vi "FP_Tracker_2.2.vi"() -> ()   [LabVIEW 2018, in "Tracker.lvlib"]
uses:
  Tracker.lvlib
  SubVi's/Controls/CTL_IO_status_indicator.ctl
  SubVi's/Controls/CTL_Zones_control_and_indicator.ctl
  SubVi's/Controls/CTL_Zone_indicator.ctl
  SubVi's/Controls/CTL_All_References.ctl
  Common/Typedefs/CTL_Controls_References.ctl
  Common/Typedefs/CTL_Indicators_References.ctl
  Common/Typedefs/CTL_Panes_and_VIs_References.ctl
  SubVi's/Controls/CTL_Cage_radial_segmentation.ctl
  SubVi's/Controls/CTL_Image_Geometrical_and_scaling_parameters.ctl
  <vilib>/ProgressBar/Progress Bar Dialog.lvclass
  SubVi's/Controls/CTL_Calibration_parameters.ctl
  SubVi's/Controls/CTL_Dispenser_calibration_info.ctl
  SubVi's/Controls/CTL_Pre-filter_params.ctl
  SubVi's/Controls/CTL_Mouse_Draw_Params.ctl
  SubVi's/Controls/CTL_IO_params_cluster.ctl
  SubVi's/Controls/CTL_Overlays_cluster.ctl
  SubVi's/Controls/CTL_Animal_Coordinates_and_Speed.ctl
  SubVi's/Controls/CTL_Settings_cluster.ctl
  SubVi's/Controls/CTL_Histogram_parameters.ctl
  SubVi's/Controls/CTL_Filter_selector.ctl
  SubVi's/Controls/CTL_Acquisition_speed_selector.ctl
  Common/Typedefs/CTL_Segmented_plot_parameters_2.ctl
  Libraries/Cage Diagram/Typedefs/CTL_Cage_type.ctl
  SubVi's/Controls/CTL_Cage_all_segmentation_params_set.ctl
  SubVi's/Controls/CTL_Conditions_Array.ctl
  SubVi's/Controls/CTL_Conditions_Cluster.ctl
  SubVi's/Controls/CTL_Condition_type.ctl
  SubVi's/Controls/CTL_Comparison_type.ctl
  SubVi's/Controls/CTL_Validity_check_criteria.ctl
  SubVi's/Controls/CTL_Response_info.ctl
  SubVi's/Controls/CTL_Condition_response_type.ctl
  SubVi's/Controls/CTL_Reponse_port_info.ctl
  SubVi's/Controls/CTL_Pixel_to_Zone_array.ctl
  SubVi's/Controls/CTL_Stats_parameters_(online).ctl
  SubVi's/Controls/CTL_Control_States.ctl
  SubVi's/Controls/CTL_States_cluster.ctl
  <vilib>/Platform/TimedLoop/XDataNode/timing_clust.ctl
  <vilib>/Platform/TimedLoop/XDataNode/nitl_modes.ctl
  <vilib>/Platform/TimedLoop/XDataNode/wakeup.ctl
  <vilib>/Utility/error.llb/DialogType.ctl
  SubVi's/Controls/CTL_Settings_parameters_groups.ctl
  Libraries/TTL IO/Typedefs/CTL_Parameter_transfer_name.ctl
  SubVi's/Controls/CTL_Post-processing_params.ctl
  <vilib>/vision/Image Controls.llb/IMAQ Image.ctl
  <vilib>/Utility/miscctls.llb/LVBoundsTypeDef.ctl
  SubVi's/Controls/CTL_Color_ramp.ctl
  <vilib>/Instr/_visa.llb/VISA Flush IO Buffer Mask.ctl
  SubVi's/Controls/CTL_Full_data_frame.ctl
  SubVi's/Controls/CTL_Measurements_and_Statistics.ctl
  <extravilib>/ChannelInstances/Stream-t'Tracker.lvlib-CTL_Full_data_frame.ctl'/Read With Abort.vi
  <extravilib>/ChannelInstances/Lossy Stream-t'Tracker.lvlib-CTL_Measurements_and_Statistics.ctl'/Write With Abort.vi
  <extravilib>/ChannelInstances/Lossy Stream-t'Tracker.lvlib-CTL_Animal_Coordinates_and_Speed.ctl'/Read With Abort.vi
  <extravilib>/ChannelInstances/Lossy Stream-a[.](dbl)/Read With Abort.vi
  <extravilib>/ChannelInstances/Lossy Stream-t'Tracker.lvlib-CTL_Measurements_and_Statistics.ctl'/Read With Abort.vi
  <extravilib>/ChannelInstances/Lossy Stream-a[.](dbl)/Write With Abort.vi
  <extravilib>/ChannelInstances/Lossy Stream-t'Tracker.lvlib-CTL_Animal_Coordinates_and_Speed.ctl'/Write With Abort.vi
  <extravilib>/ChannelInstances/Stream-t'Tracker.lvlib-CTL_Full_data_frame.ctl'/Write With Abort.vi
  <extravilib>/ChannelInstances/Stream-t'Tracker.lvlib-CTL_Full_data_frame.ctl'/EndpointRead.vi
  <extravilib>/ChannelInstances/Lossy Stream-t'Tracker.lvlib-CTL_Measurements_and_Statistics.ctl'/Endpoint.vi
  <extravilib>/ChannelInstances/Lossy Stream-t'Tracker.lvlib-CTL_Animal_Coordinates_and_Speed.ctl'/EndpointRead.vi
  <extravilib>/ChannelInstances/Lossy Stream-a[.](dbl)/EndpointRead.vi
  <extravilib>/ChannelInstances/Lossy Stream-t'Tracker.lvlib-CTL_Measurements_and_Statistics.ctl'/EndpointRead.vi
  <extravilib>/ChannelInstances/Lossy Stream-a[.](dbl)/Endpoint.vi
  <extravilib>/ChannelInstances/Lossy Stream-t'Tracker.lvlib-CTL_Animal_Coordinates_and_Speed.ctl'/Endpoint.vi
  <extravilib>/ChannelInstances/Stream-t'Tracker.lvlib-CTL_Full_data_frame.ctl'/Endpoint.vi
  <extravilib>/ChannelInstances/Lossy Stream-t'Tracker.lvlib-CTL_Measurements_and_Statistics.ctl'/Instantiate.vi
  <extravilib>/ChannelInstances/Stream-t'Tracker.lvlib-CTL_Full_data_frame.ctl'/Instantiate.vi
  <extravilib>/ChannelInstances/Lossy Stream-t'Tracker.lvlib-CTL_Animal_Coordinates_and_Speed.ctl'/Instantiate.vi
  <extravilib>/ChannelInstances/Lossy Stream-a[.](dbl)/Instantiate.vi
  SubVi's/SW_Globals_2.2+.vi
  <vilib>/Platform/TimedLoop/scheduler/LVUserAPI/_suppVIs/Create_1kHz_TSource.vi
  <extravilib>/ChannelInstances/Stream-t'Tracker.lvlib-CTL_Full_data_frame.ctl'/)Channel.vi
  <resource>/ChannelSupport/_ChannelSupport/WaitIfNeeded.vi
  <extravilib>/ChannelInstances/Lossy Stream-t'Tracker.lvlib-CTL_Measurements_and_Statistics.ctl'/)Channel.vi
  <extravilib>/ChannelInstances/Lossy Stream-t'Tracker.lvlib-CTL_Animal_Coordinates_and_Speed.ctl'/)Channel.vi
  <extravilib>/ChannelInstances/Lossy Stream-a[.](dbl)/)Channel.vi
  <vilib>/nisyscfg/Close (Resources).vi
  <vilib>/nisyscfg/Close (System).vi
  <userlib>/_OpenG.lib/file/file.llb/Valid Path - Traditional__ogtk.vi
  <vilib>/Utility/file.llb/Write Delimited Spreadsheet (DBL).vi
  <userlib>/_OpenG.lib/file/file.llb/File Exists - Scalar__ogtk.vi
  <vilib>/Platform/TimedLoop/XDataNode/XDataNode.xnode
  <vilib>/Platform/TimedLoop/XDataNode/XDNodeRunTimeDep.lvlib
  Common_Resources.lvlib
  <vilib>/nisyscfg/nisyscfg.lvlib
  <resource>/objmgr/nicontrollersysapi.rc
  <vilib>/Utility/config.llb/NI_LVConfig.lvlib
  <resource>/objmgr/nisysapi.rc
  Device low-level comms.lvlib
  <vilib>/Analysis/NI_AALBase.lvlib
  <extravilib>/ChannelInstances/Lossy Stream-a[.](dbl).lvlib
  <extravilib>/ChannelInstances/Stream-t'Tracker.lvlib-CTL_Full_data_frame.ctl'.lvlib
  <extravilib>/ChannelInstances/Lossy Stream-t'Tracker.lvlib-CTL_Animal_Coordinates_and_Speed.ctl'.lvlib
  <extravilib>/ChannelInstances/Lossy Stream-t'Tracker.lvlib-CTL_Measurements_and_Statistics.ctl'.lvlib
  <vilib>/ptbypt/NI_PtbyPt.lvlib
  Libraries/Tracks Repair/Tracks Repair.lvlib
  Libraries/Stream Data/Stream Data.lvlib
  Libraries/TTL IO/TTL IO.lvlib
  Libraries/Cage Diagram/Cage Diagram.lvlib
panel:
  out "VISA resource name out":refnum<visa-resource-name>
  in  "Load custom? (F)":bool
  out "Settings path to load":path
  out "Loaded.TDMS.path":path
  out "Frame #":u32
  in  "Start over":bool
  out "Active speed chunk":dbl[](array[numeric])
  out "Active part of track":cluster{"Numeric":dbl, "Numeric":dbl}[](array[cluster])
  in  "Stats parameters (online)":T1={"Mouse drawing parameters"={"Trace length, samples"=0, "Rainbow track"=FALSE, "Rainbow track is speed"=FALSE, "Bright mouse lineout"=FALSE, "Colors array"=[], "Pixels per mm"=0.0}, "Size of the image (480x480)"={"Numeric Control"=480.0, "Numeric Control"=480.0}, "Array of the pixel to zone correspondences"=[], "Hist. bins array"=[], "Histogram parameters"={"max"=300.0, "min"=0.0, "# bins"=10, "threshold"=8.0, "thr. type"=enum."higher accepted"}}
  out "Hist. X axis":dbl[](array[numeric])
  out "Loaded.zones":i8[](array[numeric])
  out "Pixel to zone":T3
  out "Current zone":T5
  in  "Save settings":bool
  in  "Reset zones":bool
  in  "Reset stimuli":bool
  out "Array of conditions":T6 {"Specifier(s)"."Validity criteria(s)"."Validity value" min=0.0 step=0.1 format="%.2g"; "Specifier(s)"."Value" step=1.0 format="%#.2g"}
  out "Ready":bool=TRUE
  in  "Check HW connection":bool
  in  "Set IO config":bool
  in  "Cage radial segmentation":T14={"CENTER"={"Radius, mm CENTER"=30}, "MIDFIELD"={"Radius, mm MIDFIELD"=75, "N segments MIDFIELD"=2, "Starting angle MIDFIELD"=0}, "BORDER"={"N segments BORDER"=4, "Starting angle BORDER"=0}} caption="Radial segmentation" {"BORDER"."N segments BORDER" min=1 max=12; "MIDFIELD"."N segments MIDFIELD" max=8; "CENTER"."Radius, mm CENTER" min=5 step=1}
  in  "Diagram (generated)":T15(plugin-control)=refnum
  out "Act. frame time, s":dbl
  out "Settings cluster (local)":T16={"Defaults"={"Default User"=0.0, "VISA Resource Name "="", "Histogram parameters"={"max"=300.0, "min"=0.0, "# bins"=10, "threshold"=8.0, "thr. type"=enum."higher accepted"}}, "Recording and saving"={"Researcher name"="", "Name prefix"="", "Data post-processing"={"Filter type"=enum."Savitzky-Golay", "Length"=31, "Order"=3}, "Stop at"=0.0, "\"Stop at\" enabled"=FALSE, "Default save folder path"=path "", "Acquisition FPS"=enum."Max"}, "Geometry"={"Sensor board size"=enum."", "Bridge swap"=FALSE, "Twisted neck"=FALSE, "Bridge H. offset"=0.0, "Bridge V. offset"=0.0, "Magnets orientation"=0.0, "Cage type"=0, "Cage parameters"={"Round"=variant(i16 0), "Square"=variant(u16 0), "Donut-maze"=variant(u16 0), "T-maze"=variant(u8 0), "Sociability-maze"=variant(u8 0)}}, "IO parameters"={"IO general config."=0, "IO 1 configuration"=0, "IO 2 configuration"=0, "IO 3 configuration"=0, "IO 4 configuration"=0, "Activate ext. RS-232"=0, "IO inversion config."=0, "Sync capability"=1}, "Conditions presets array"=[{"Enabled"=FALSE, "Name"="", "Specifier(s)"=[], "Response"={"Response type"=enum."Air puff", "TTL port"=enum."Port 1", "TTL pulse length, ms"=0.0}, "Has been set"=FALSE}, {"Enabled"=FALSE, "Name"="", "Specifier(s)"=[], "Response"={"Response type"=enum."Air puff", "TTL port"=enum."Port 1", "TTL pulse length, ms"=0.0}, "Has been set"=FALSE}, {"Enabled"=FALSE, "Name"="", "Specifier(s)"=[], "Response"={"Response type"=enum."Air puff", "TTL port"=enum."Port 1", "TTL pulse length, ms"=0.0}, "Has been set"=FALSE}, {"Enabled"=FALSE, "Name"="", "Specifier(s)"=[], "Response"={"Response type"=enum."Air puff", "TTL port"=enum."Port 1", "TTL pulse length, ms"=0.0}, "Has been set"=FALSE}, {"Enabled"=FALSE, "Name"="", "Specifier(s)"=[], "Response"={"Response type"=enum."Air puff", "TTL port"=enum."Port 1", "TTL pulse length, ms"=0.0}, "Has been set"=FALSE}, {"Enabled"=FALSE, "Name"="", "Specifier(s)"=[], "Response"={"Response type"=enum."Air puff", "TTL port"=enum."Port 1", "TTL pulse length, ms"=0.0}, "Has been set"=FALSE}, {"Enabled"=FALSE, "Name"="", "Specifier(s)"=[], "Response"={"Response type"=enum."Air puff", "TTL port"=enum."Port 1", "TTL pulse length, ms"=0.0}, "Has been set"=FALSE}, {"Enabled"=FALSE, "Name"="", "Specifier(s)"=[], "Response"={"Response type"=enum."Air puff", "TTL port"=enum."Port 1", "TTL pulse length, ms"=0.0}, "Has been set"=FALSE}, {"Enabled"=FALSE, "Name"="", "Specifier(s)"=[], "Response"={"Response type"=enum."Air puff", "TTL port"=enum."Port 1", "TTL pulse length, ms"=0.0}, "Has been set"=FALSE}, {"Enabled"=FALSE, "Name"="", "Specifier(s)"=[], "Response"={"Response type"=enum."Air puff", "TTL port"=enum."Port 1", "TTL pulse length, ms"=0.0}, "Has been set"=FALSE}, {"Enabled"=FALSE, "Name"="", "Specifier(s)"=[], "Response"={"Response type"=enum."Air puff", "TTL port"=enum."Port 1", "TTL pulse length, ms"=0.0}, "Has been set"=FALSE}, {"Enabled"=FALSE, "Name"="", "Specifier(s)"=[], "Response"={"Response type"=enum."Air puff", "TTL port"=enum."Port 1", "TTL pulse length, ms"=0.0}, "Has been set"=FALSE}, {"Enabled"=FALSE, "Name"="", "Specifier(s)"=[], "Response"={"Response type"=enum."Air puff", "TTL port"=enum."Port 1", "TTL pulse length, ms"=0.0}, "Has been set"=FALSE}, {"Enabled"=FALSE, "Name"="", "Specifier(s)"=[], "Response"={"Response type"=enum."Air puff", "TTL port"=enum."Port 1", "TTL pulse length, ms"=0.0}, "Has been set"=FALSE}], "Calibration parameters"={"Timing calibration sw/hw"=1.0, "True FPS"=80.0, "True frame time, s"=80.0, "Disp. calibration info"=[]}, "Settings loaded OK"=FALSE} {"Calibration parameters"."True frame time, s" format="%.10g"; "Calibration parameters"."Disp. calibration info"."Speed, µl per ms" format="%.3g"; "Calibration parameters"."True FPS" format="%.10g"; "Calibration parameters"."Timing calibration sw/hw" format="%.10g"; "Conditions presets array"."Specifier(s)"."Validity criteria(s)"."Validity value" min=0.0 step=0.1 format="%.2g"; "Conditions presets array"."Specifier(s)"."Value" step=1.0 format="%#.2g"; "Recording and saving"."Data post-processing"."Order" min=3 max=11 step=2; "Recording and saving"."Data post-processing"."Length" min=5 max=301 step=2; "Geometry"."Cage type" items=["Round", "Square", "Donut-maze", "T-maze", "Sociability maze", ""]}
  out "Loaded.TTL IO and Key":string[][](array[string])
  out "Loaded.HW ts and Frame HW time":u32[][](array[numeric])
  out "Loaded.Properties":string[][](array[string])
  out "Current position":T25
  out "Update timeline index?":bool
  out "Cur. pos. slider index":i32
  out "Timeline absolute min&max indices":T26
  out "Timeline absolute min&max":cluster{"Tl. min":dbl, "TL. max":dbl}
  out "Timeline min&max indices":T26
  out "Loaded.timeline":dbl[](array[numeric])
  out "Loaded.speed":dbl[](array[numeric])
  out "Loaded.alpha":dbl[](array[numeric])
  out "Loaded.Y":dbl[](array[numeric])
  out "Loaded.X":dbl[](array[numeric])
  out "Timeline min&max":cluster{"Tl. min":dbl, "TL. max":dbl}
  in  "Reset buffers?":bool
  out "Overlays cluster":T27
  out "Track show state":u32
  out "Start time (HW)":u32
  out "TTL in time (HW)":u32
  out "Key_pressed":string caption="Key"
  out "TDMS ref.":refnum<k34>
  out "TTL in time (SW)":timestamp
  out "IO parameters":T22
  out "Start time (SW)":timestamp
  out "Mouse drawing parameters":T2
  out "Pre-filter params.":T28
  out "Sensor board size":string
  out "FPS status":i32=80
  out "Rainbow is speed":bool=TRUE
  out "Calibration parameters":T23={"Timing calibration sw/hw"=1.0, "True FPS"=80.0, "True frame time, s"=80.0, "Disp. calibration info"=[]} {"True frame time, s" format="%.10g"; "Disp. calibration info"."Speed, µl per ms" format="%.3g"; "True FPS" format="%.10g"; "Timing calibration sw/hw" format="%.10g"}
  in  "Calibration samples":i32=2000
  out "Calibration SW timings":dbl[](array[numeric])
  out "Calibration HW timings":u32[](array[numeric])
  out "Progress Bar Dialog":refnum<class "Progress Bar Dialog.lvclass">
  out "VISA Resources found":string[](array[string])
  out "CPU load":sgl(slide) scale=0.0..100.0
  in  "ROIs list":i32(listbox)
  out "ROIs":T29
  out "Rainbow track":bool=TRUE
  out "Colors array":u32[](array[colorbox])
  out "UI update period":i64=53
  out "Trace length, samples":u16(slide)=20 scale=0.0..2000.0
  out "Bright mouse lineout":bool
  out "Img geom and scaling":T30
  out "Ports IO config":bool[](array[boolean])
  out "SB size":u8
  out "VISA resource name":refnum<visa-resource-name>
  out "Cage size":string="Large" caption="Cage diameter"
  in  "Set/Rec and Analyse Tab":enum32{"Settings", "Recording and Analysis"}(tab)
  in  "Reward and stimulation":string(tree) caption="Reward and stimulation conditions"
  in  "Add Reward":bool=TRUE
  in  "Modify Reward":bool=TRUE
  in  "Remove Reward":bool=TRUE
  out "Active rules":T31
  out "Average speed, mm/s":dbl caption="Avg., mm/s" format="%05.1f"
  out "Run distance, m":dbl caption="Distance, m" format="%0.3f"
  in  "Speed threshold":dbl=8.0 caption="@ mm/s >" format="%05.1f"
  in  "Rainbow (speed)":bool caption="Spdcode"
  in  "Rainbow (time)":bool caption="Timecode"
  in  "Show magnets":bool=TRUE caption="Magnets"
  in  "Playback speed":u16(ring)=3 caption="Speed" items=["5"=24, "4"=30, "3"=40, "2"=60, "1"=120, "1/2"=240, "1/3"=360, "1/4"=480, "1/5"=600]
  in  "Show heatmap":bool caption="Heat map"
  in  "Show full track":bool caption="Full track"
  in  "Show zones":bool=TRUE caption="Zones"
  in  "Trace, s":u16(slide)=5 max=30 step=1 scale=0.0..30.0
  in  "Multiplyer of chart RX":u8(slide)=1 max=9 step=1 scale=0.0..9.0
  out "Running, perc. of time":dbl caption="Run time, %" format="%05.2f"
  out "Histograms":T32(graph) caption="Speed histogram"
  in  "Reset barplot":bool
  out "Mouse speed":waveform(dbl)(graph)
  out "Mouse speed, mm/s":dbl caption="Speed, mm/s" format="%05.1f"
  out "Timing Source":string
  in  "Panes references":T33
  in  "Indicators references":T34
  in  "Controls references":T35
  in  "All references":T36
  in  "Diagram (display)":T15(plugin-control)=refnum
  out "HW info":string
  out "Port":string="Large"
  in  "Timeline":T37(slide)={"Slider"=0.0, "Slider"=648.2670807453416, "Slider"=2749.5465838509317} scale=0.0..60.0 scale format="%<%H:%M:%S>t"
  in  "Play/Pause":bool
  in  "Open File":bool
  out "Since track start":dbl format="%<%H:%M:%S%1u>t"
  out "Current Time":timestamp=timestamp(3680686800.229 s since 1904-01-01) format="%<%H:%M:%S %d.%m.%Y>T"
  in  "Record/Stop":bool
  in  "By Zone stim. setup":T38=enum."Zone 13"
  out "IO status indicator":T39
  in  "error in (no error)":errorcluster
  out "error out":errorcluster={"status"=TRUE, "code"=1, "source"="Dequeue Element in NI_LVConfig.lvlib:Read Value Without Comment.vi->NI_LVConfig.lvlib:Read Key (I32).vi->SW_Load_settings_to_main_tab.vi"}
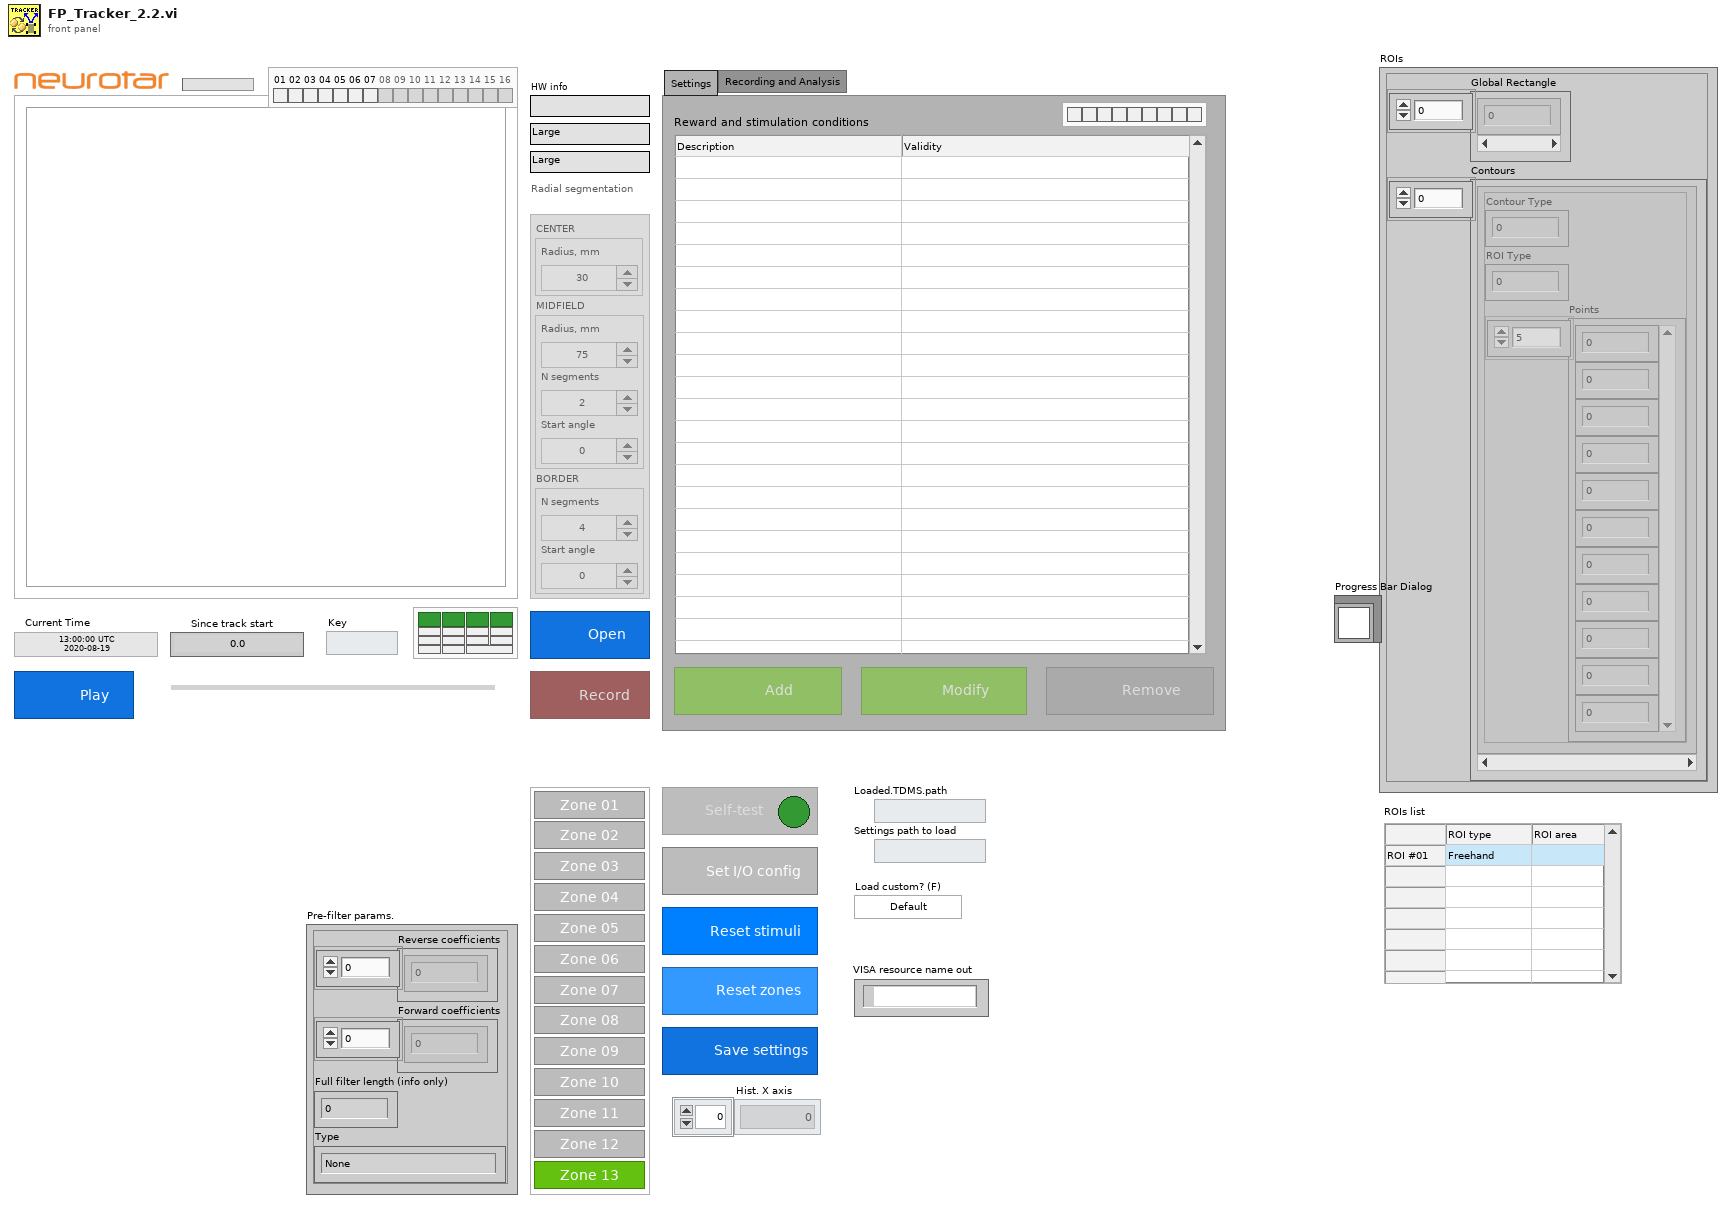
[diagram p1: front panel]
types:
  T1 = typedef "Common_Resources.lvlib/CTL_Stats_parameters_(online).ctl" = cluster{"Mouse drawing parameters":T2, "Size of the image (480x480)":cluster{"Numeric Control":dbl, "Numeric Control":dbl}, "Array of the pixel to zone correspondences":T3, "Hist. bins array":dbl[], "Histogram parameters":T4}
  T2 = typedef "Common_Resources.lvlib/CTL_Mouse_Draw_Params.ctl" = cluster{"Trace length, samples":u16, "Rainbow track":bool, "Rainbow track is speed":bool, "Bright mouse lineout":bool, "Colors array":u32[], "Pixels per mm":dbl}
  T3 = typedef "Common_Resources.lvlib/CTL_Pixel_to_Zone_array.ctl" = i8[][]
  T4 = typedef "Common_Resources.lvlib/CTL_Histogram_parameters.ctl" = cluster{"max":dbl, "min":dbl, "# bins":i32, "threshold":dbl, "thr. type":enum16{"higher accepted", "lower accepted"}}
  T5 = typedef "Common_Resources.lvlib/CTL_Zone_indicator.ctl" = cluster{"01":bool, "02":bool, "03":bool, "04":bool, "05":bool, "06":bool, "07":bool, "08":bool, "09":bool, "10":bool, "11":bool, "12":bool, "13":bool, "14":bool, "15":bool, "16":bool}
  T6 = typedef "Common_Resources.lvlib/CTL_Conditions_Array.ctl" = T7[]
  T7 = typedef "Common_Resources.lvlib/CTL_Conditions_Cluster.ctl" = cluster{"Enabled":bool, "Name":string, "Specifier(s)":cluster{"Specifier enabled":bool, "Condition type":T8, "Comparison type":T9, "Value":dbl, "Validity criteria(s)":cluster{"V. check enabled":bool, "Criteria":T10, "Validity value":dbl}[]}[], "Response":T11, "Has been set":bool}
  T8 = typedef "Common_Resources.lvlib/CTL_Condition_type.ctl" = enum16{"Speed", "Zone", "Angle to wall"}
  T9 = typedef "Common_Resources.lvlib/CTL_Comparison_type.ctl" = enum16{"Less", "Less or Equal", "Equal", "Greater or Equal", "Greater", "Not Equal"}
  T10 = typedef "Common_Resources.lvlib/CTL_Validity_check_criteria.ctl" = enum16{"Running bout (seconds)", "Running bout (meters)"}
  T11 = typedef "Common_Resources.lvlib/CTL_Response_info.ctl" = cluster{"Response type":T12, "TTL port":T13, "TTL pulse length, ms":dbl}
  T12 = typedef "Common_Resources.lvlib/CTL_Condition_response_type.ctl" = enum16{"None", "Air puff", "Liquid reward", "TTL pulse", "TTL pulse (ubr)", "TTL signal"}
  T13 = typedef "Common_Resources.lvlib/CTL_Reponse_port_info.ctl" = enum16{"Port 1", "Port 2", "Port 3", "Port 4"}
  T14 = typedef "Common_Resources.lvlib/CTL_Cage_radial_segmentation.ctl" = cluster{"CENTER":cluster{"Radius, mm CENTER":u16}, "MIDFIELD":cluster{"Radius, mm MIDFIELD":u16, "N segments MIDFIELD":u8, "Starting angle MIDFIELD":i16}, "BORDER":cluster{"N segments BORDER":u8, "Starting angle BORDER":i16}}
  T15 = typedef "IMAQ Image.ctl" = refnum<image>
  T16 = typedef "Common_Resources.lvlib/CTL_Settings_cluster.ctl" = cluster{"Defaults":cluster{"Default User":dbl, "VISA Resource Name ":string, "Histogram parameters":T4}, "Recording and saving":cluster{"Researcher name":string, "Name prefix":string, "Data post-processing":T17, "Stop at":dbl, "\"Stop at\" enabled":bool, "Default save folder path":path, "Acquisition FPS":T18}, "Geometry":T19, "IO parameters":T22, "Conditions presets array":T6, "Calibration parameters":T23, "Settings loaded OK":bool}
  T17 = typedef "Common_Resources.lvlib/CTL_Filter_selector.ctl" = cluster{"Filter type":enum16{"None", "Savitzky-Golay"}, "Length":i32, "Order":i32}
  T18 = typedef "Common_Resources.lvlib/CTL_Acquisition_speed_selector.ctl" = enum16{"Max", "Optimal", "Eco"}
  T19 = typedef "Common_Resources.lvlib/CTL_Segmented_plot_parameters_2.ctl" = cluster{"Sensor board size":enum16{"", "Large"}, "Bridge swap":bool, "Twisted neck":bool, "Bridge H. offset":sgl, "Bridge V. offset":sgl, "Magnets orientation":sgl, "Cage type":T20, "Cage parameters":T21}
  T20 = typedef "Cage Diagram.lvlib/CTL_Cage_type.ctl" = u16
  T21 = typedef "Common_Resources.lvlib/CTL_Cage_all_segmentation_params_set.ctl" = cluster{"Round":variant, "Square":variant, "Donut-maze":variant, "T-maze":variant, "Sociability-maze":variant}
  T22 = typedef "Common_Resources.lvlib/CTL_IO_params_cluster.ctl" = cluster{"IO general config.":u16, "IO 1 configuration":u16, "IO 2 configuration":u16, "IO 3 configuration":u16, "IO 4 configuration":u16, "Activate ext. RS-232":u16, "IO inversion config.":u16, "Sync capability":u8}
  T23 = typedef "Common_Resources.lvlib/CTL_Calibration_parameters.ctl" = cluster{"Timing calibration sw/hw":dbl, "True FPS":dbl, "True frame time, s":dbl, "Disp. calibration info":T24}
  T24 = typedef "Common_Resources.lvlib/CTL_Dispenser_calibration_info.ctl" = cluster{"Channel":u8, "Speed, µl per ms":dbl}[]
  T25 = typedef "Common_Resources.lvlib/CTL_Animal_Coordinates_and_Speed.ctl" = cluster{"R from center":dbl, "phi (mouse angular position in the cage)":dbl, "alpha (mouse rot. angle)":dbl, "X":dbl, "Y":dbl, "theta (from center towards mouse)":dbl, "beta (cage rot. against mouse)":dbl, "w (mouse angle to wall)":dbl, "Speed (filtered)":dbl}
  T26 = cluster{"Tl. min index":i32, "Tl. max index":i32}
  T27 = typedef "Common_Resources.lvlib/CTL_Overlays_cluster.ctl" = cluster{"Time-coded track overlay (array)":u32[][], "Speed-coded track overlay (array)":u32[][], "Plain track overlay pixmap":u32[][], "Location density map image":u32[][], "Speed density map image":u32[][], "Location density map":dbl[][], "Speed density map":dbl[][]}
  T28 = typedef "Common_Resources.lvlib/CTL_Pre-filter_params.ctl" = cluster{"Reverse coefficients":dbl[], "Forward coefficients":dbl[], "Full filter length (info only)":i32, "Type":enum16{"None", "FIR (PtbyPt)", "IIR (PtbyPt)"}}
  T29 = cluster{"Global Rectangle":i32[], "Contours":cluster{"Contour Type":u32, "ROI Type":u32, "Points":i32[]}[]}
  T30 = typedef "Common_Resources.lvlib/CTL_Image_Geometrical_and_scaling_parameters.ctl" = cluster{"Fonts scale factor":dbl, "Pixels per mm":dbl, "Radius of displayed outer segments, pix":dbl, "Radius of displayed midfield segments, pix":dbl, "Radius of displayed central segment, pix":dbl}
  T31 = cluster{"01":bool, "02":bool, "03":bool, "04":bool, "05":bool, "06":bool, "07":bool, "08":bool, "09":bool}
  T32 = cluster{"X Values":dbl[], "Histogram: h(x)":dbl[]}
  T33 = typedef "Common_Resources.lvlib/CTL_Panes_and_VIs_References.ctl" = cluster{"Pane":refnum<vi>, "This VI":refnum<vi>, "Menu":refnum<k9>}
  T34 = typedef "Common_Resources.lvlib/CTL_Indicators_References.ctl" = cluster{"HW info":refnum<vi>, "Port":refnum<vi>, "Ready":refnum<vi>, "IO status indicator":refnum<vi>, "Current Time":refnum<vi>, "Record timestamp":refnum<vi>, "Mouse speed":refnum<vi>, "Mouse speed, mm/s":refnum<vi>, "Running, perc. of time":refnum<vi>, "Histograms":refnum<vi>, "Cage size":refnum<vi>, "Reward":refnum<vi>, "Current zone":refnum<vi>, "Run length, m":refnum<vi>}
  T35 = typedef "Common_Resources.lvlib/CTL_Controls_References.ctl" = cluster{"Check HW connection":refnum<vi>, "Save settings":refnum<vi>, "Reset zones":refnum<vi>, "Reset stimuli":refnum<vi>, "Record/Stop":refnum<vi>, "Reset barplot":refnum<vi>, "Multiplyer of chart RX":refnum<vi>, "Show zones":refnum<vi>, "Show magnets":refnum<vi>, "Show heatmap":refnum<vi>, "Show full track":refnum<vi>, "Open File":refnum<vi>, "Play/Pause":refnum<vi>, "Trace, s":refnum<vi>, "Playback speed":refnum<vi>, "Timeline":refnum<vi>, "By Zone stim. setup":refnum<vi>, "Set/Rec and Analyse Tab":refnum<vi>, "Cage radial segmentation":refnum<vi>, "Set IO config":refnum<vi>, "Rainbow (time)":refnum<vi>, "Rainbow (speed)":refnum<vi>, "Add Reward":refnum<vi>, "Modify Reward":refnum<vi>, "Delete Reward":refnum<vi>, "Speed threshold, mm/s":refnum<vi>, "Start Over":refnum<vi>}
  T36 = typedef "Common_Resources.lvlib/CTL_All_References.ctl" = cluster{"Controls references":T35, "Indicators references":T34, "Service references":T33}
  T37 = cluster{"Slider":dbl, "Slider":dbl, "Slider":dbl}
  T38 = typedef "Common_Resources.lvlib/CTL_Zones_control_and_indicator.ctl" = enum32{"No Selection", "Zone 01", "Zone 02", "Zone 03", "Zone 04", "Zone 05", "Zone 06", "Zone 07", "Zone 08", "Zone 09", "Zone 10", "Zone 11", "Zone 12", "Zone 13"}
  T39 = typedef "Common_Resources.lvlib/CTL_IO_status_indicator.ctl" = cluster{"IO1":bool, "IO2":bool, "IO3":bool, "IO4":bool, "St1":bool, "St2":bool, "St3":bool, "St4":bool, "Z1":bool, "Z2":bool, "Z3":bool, "Z4":bool, "Syn1":bool, "Syn2":bool, "RS-232 ext. activated":bool}
  T40 = cluster{"[0]":bool, "[1]":bool, "[2]":bool, "[3]":bool, "[4]":bool, "[5]":bool, "[6]":bool, "[7]":bool, "[8]":bool}
  T41 = cluster{"Boolean Round":bool, "code":i32, "source":string}
  T42 = typedef "Tracks Repair.lvlib/Broadcast Events--cluster.ctl" = cluster{"Module Did Init":refnum<user-event>, "Status Updated":refnum<user-event>, "Error Reported":refnum<user-event>, "Module Did Stop":refnum<user-event>, "Update Module Execution Status":refnum<user-event>}
  T43 = typedef "Stream Data.lvlib/Broadcast Events--cluster.ctl" = cluster{"Module Did Init":refnum<user-event>, "Status Updated":refnum<user-event>, "Error Reported":refnum<user-event>, "Module Did Stop":refnum<user-event>, "Update Module Execution Status":refnum<user-event>}
  T44 = typedef "TTL IO.lvlib/Broadcast Events--cluster.ctl" = cluster{"Module Did Init":refnum<user-event>, "Status Updated":refnum<user-event>, "Error Reported":refnum<user-event>, "Module Did Stop":refnum<user-event>, "Update Module Execution Status":refnum<user-event>, "Conditions that are TRUE (active rules)":refnum<user-event>}
  T45 = typedef "Cage Diagram.lvlib/Broadcast Events--cluster.ctl" = cluster{"Module Did Init":refnum<user-event>, "Status Updated":refnum<user-event>, "Error Reported":refnum<user-event>, "Module Did Stop":refnum<user-event>, "Update Module Execution Status":refnum<user-event>, "Broadcast New Layout":refnum<user-event>}
  T46 = typedef "Common_Resources.lvlib/CTL_States_cluster.ctl" = cluster{"Acq. is ON":bool, "Playing loaded":bool, "Recording now":bool, "Has been recorded":bool, "Data saved":bool, "Data loaded":bool, "Calibration mode":bool, "Offline mode":bool, "Stop and Exit":bool, "Updating layout":bool}
  T47 = typedef "Common_Resources.lvlib/CTL_Control_States.ctl" = enum16{"SW Init", "HW Init", "Close App", "Update port info (Init OK)", "Unlock UI (init OK)", "Save HW Settings", "Re-check HW (init failed)", "Configure port(s)", "Switch to Offline mode", "Switch to Online mode", "Zones layout update", "Set I/O config (silent)", "Set I/O config", "Play Start", "Play Stop", "Upd. FPS", "Upd. trace length", "Cage and recording settings", "Update filter", "Timings calibration start", "Timings calibration finish", "Dispension calibration", "Save all settings to custom location", "Save all settings", "Start Recording", "Stop Recording", "Recording post-processing", "Timeline update", "Overlay tracks update", "Load custom settings", "Load recorded data", "Save density map(s)", "Process loaded settings", "Prepare loaded data playback", "Add Reward condition", "Modify Reward condition", "Delete Reward condition", "Check Reward condition(s)", "Location map update", "Speed map update", "Start over", "Default (test)", "IDL Error", "Recalculate track with new settings"}
  T48 = typedef "XDNodeRunTimeDep.lvlib/timing_clust.ctl" = cluster{"Expected End [f-1]":u64, "Actual End [f-1]":u64, "Finished Late? [f-1]":bool, "Expected End [i-1]":u64, "Actual End [i-1]":u64, "Finished Late? [i-1]":bool, "Expected Start [i]":u64, "Actual Start [i]":u64, "Expected Start [f]":u64, "Actual Start [f]":u64, "Source Name":string, "Structure Name":string, "Period":i64, "Deadline":i64, "Offset":i64, "Start":i64, "Priority":i32, "Timeout":i32, "Mode":T49, "Wakeup Reason":T50, "Error":errorcluster, "Source Type":string, "Secondary Source Type":string, "Global End Time":u64, "Global Start Time":u64, "Frame Duration":u64, "Iteration Duration":u64, "Assigned CPU":i32, "I/O Scan Engine Mode":u32}
  T49 = typedef "XDNodeRunTimeDep.lvlib/nitl_modes.ctl" = enum32{"No Change", "Process missed periods, maintain original phase", "Discard missed periods, maintain original phase", "Process missed periods, ignore original phase", "Discard missed periods, ignore original phase"}
  T50 = typedef "XDNodeRunTimeDep.lvlib/wakeup.ctl" = enum32{"Normal", "Aborted", "Asynchronous wakeup", "Timing source error", "Timed loop error", "Timeout"}
  T51 = cluster{"Numeric Control":u32, "Numeric Control":u32}[]
  T52 = typedef "Common_Resources.lvlib/CTL_Settings_parameters_groups.ctl" = string
  T53 = enum32{"Page Enabled", "Page Disabled", "Page Disabled & Grayed"}
  T54 = enum8{"Enabled", "Disabled", "Disabled and Grayed Out"}
  T55 = typedef "TTL IO.lvlib/CTL_Parameter_transfer_name.ctl" = enum16{"None", "All parameters", "IO parameters", "Conditions"}
  T56 = typedef "Common_Resources.lvlib/CTL_Post-processing_params.ctl" = cluster{"Defragment TDMS? (F)":bool, "Start time (SW)":timestamp, "Start time (HW)":u32, "Data filtering":T17, "Mouse drawing parameters":T2, "Size of the image (480x480)":cluster{"X size":dbl, "Y size":dbl}, "Image ref. in":T15, "Calibration parameters":T23, "Pixel to zone":T3}
  T57 = cluster{"TL. min index":i32, "TL. max index":i32}
  T58 = typedef "LVBoundsTypeDef.ctl" = cluster{"Width":u32, "Height":u32}
  T59 = typedef "DialogType.ctl" = u16
  T60 = cluster{"Previous step":T47, "error IO":errorcluster}
  T61 = enum32{"invalid app kind", "Development System", "Run Time System", "Student Edition", "Embedded LabVIEW", "Evaluation", "Custom"}
  T62 = typedef "Cage Diagram.lvlib/New Layout (instant) (Reply Payload)--cluster.ctl" = cluster{"Cage Diagram ref":T15, "Pixel <> Zone":T3, "Cage drawing parameters out":T63, "New Layout (instant)_error":errorcluster}
  T63 = typedef "Cage Diagram.lvlib/CTL_Cage_drawing_params.ctl" = cluster{"Draw Area Size":T64, "Cage External Dims.":T65, "Background color":u32, "Image Scaling info":T66, "Segments Colors":T67}
  T64 = typedef "Common_Resources.lvlib/CTL_Draw_Area_Size.ctl" = cluster{"Width, pix":i32, "Height, pix":i32}
  T65 = typedef "Cage Diagram.lvlib/CTL_Cage_External_dimensions.ctl" = cluster{"Width, mm":dbl, "Height, mm":dbl}
  T66 = typedef "Cage Diagram.lvlib/CTL_Image_Scaling_info.ctl" = cluster{"Fonts scale factor":dbl, "Pixels per mm":dbl}
  T67 = typedef "Common_Resources.lvlib/CTL_Segments_Colors_(pie).ctl" = cluster{"Colors array for outer segments":u32[], "Colors array for midfield segments":u32[], "Color for central segment":u32, "Fill color for no segments image":u32}
  T68 = typedef "Common_Resources.lvlib/CTL_Paths_cluster.ctl" = cluster{"Program settings":path, "Folder":path, "TDMS file reference":refnum<k34>, "TDMS track":path, "Track settings":path, "Layout picture":path, "Density map matrix (time)":path, "Density map picture (time)":path, "Density map matrix (speed)":path, "Density map picture (speed)":path, "ZIP":path}
  T69 = typedef "NI_LVConfig.lvlib/Config Data RefNum.ctl" = refnum<k1>
  T70 = enum16{"Left Button", "Center Button", "Right Button", "Window Close"}
  T71 = cluster{"Geometry out":T19, "Value":bool, "Value":bool}
  T72 = cluster{"Slider 1":dbl, "Slider 2":dbl, "Slider 3":dbl}
  T73 = cluster{"Numeric Control":dbl, "Numeric Control":dbl}
  T74 = typedef "Common_Resources.lvlib/CTL_Loaded_data_output_(offline).ctl" = cluster{"HW ts and Frame HW time":u32[][], "SW timestamp":dbl[], "TTL IO and Key":string[][], "Track properties":string[][], "Coords data":dbl[][], "Zone":i8[]}
  T75 = typedef "Cage Diagram.lvlib/Get Layout Image as Array (Reply Payload)--cluster.ctl" = cluster{"Layout image array (U32)":u32[][], "Get Layout Image as Array_error":errorcluster}
  T76 = typedef "imagedata.ctl" = cluster{"image type":i32, "image depth":i32, "image":u8[], "mask":u8[], "colors":u32[], "Rectangle":cluster{"left":i16, "top":i16, "right":i16, "bottom":i16}}
  T77 = typedef "Common_Resources.lvlib/CTL_Color_ramp.ctl" = u32[]
  T78 = typedef "LVNodeAndColumnTypeDef.ctl" = cluster{"Node":string, "Column":i32}
  T79 = typedef "VISA Flush IO Buffer Mask.ctl" = u16
  T80 = typedef "Common_Resources.lvlib/CTL_Full_data_frame.ctl" = cluster{"Times":cluster{"ms since ON":u32, "delta time":u32, "Frame timestamp":timestamp}, "TTLs":cluster{"TTL input":i16, "TTL output":i16}, "Animal coordinates":T25, "Magnets coords raw":cluster{"X1 raw":dbl, "Y1 raw":dbl, "X2 raw":dbl, "Y2 raw":dbl}, "Measurements and statistics":T81}
  T81 = typedef "Common_Resources.lvlib/CTL_Measurements_and_Statistics.ctl" = cluster{"Zone #":i8, "Histogram":dbl[], "Running, perc. of time":dbl, "Run, meters":dbl, "Avg. speed":dbl}
  T82 = typedef "Lossy Stream-a[.](dbl).lvlib/)Channel.ctl" = refnum<queue>
  T83 = typedef "Common_Resources.lvlib/CTL_Decoded_data_frame.ctl" = cluster{"ms since ON":u32, "delta time":u32, "X1":sgl, "Y1":sgl, "X2":sgl, "Y2":sgl, "TTL input":i16, "TTL output":i16, "Frame timestamp":timestamp, "Frame OK":bool}
  T84 = cluster{"X1 raw":dbl, "Y1 raw":dbl, "X2 raw":dbl, "Y2 raw":dbl}
  T85 = cluster{"ms since ON":u32, "delta time":u32, "Frame timestamp":timestamp}
  T86 = typedef "Common_Resources.lvlib/CTL_Cage_Coords.ctl" = cluster{"R from center":dbl, "sin(a)":dbl, "Mouse Xc":dbl, "Mouse Yc":dbl, "X1-X2":dbl, "Y1-Y2":dbl, "Cage Xc":dbl, "Cage Yc":dbl, "Frame time, s":dbl}
  T87 = typedef "Lossy Stream-t'Tracker.lvlib-CTL_Animal_Coordinates_and_Speed.ctl'.lvlib/)Channel.ctl" = refnum<queue>
  T88 = typedef "Stream-t'Tracker.lvlib-CTL_Full_data_frame.ctl'.lvlib/)Channel.ctl" = refnum<queue>
  T89 = typedef "Tracker.lvlib/CTL_States_cluster.ctl" = cluster{"Acq. is ON":bool, "Playing loaded":bool, "Recording now":bool, "Has been recorded":bool, "Data saved":bool, "Data loaded":bool, "Calibration mode":bool, "Offline mode":bool, "Stop and Exit":bool, "Updating layout":bool}
  T90 = typedef "Lossy Stream-t'Tracker.lvlib-CTL_Measurements_and_Statistics.ctl'.lvlib/)Channel.ctl" = refnum<queue>
  T91 = cluster{"Tl. min":dbl, "TL. max":dbl, "Numeric":dbl}
  T92 = cluster{"array[0]":bool, "array[1]":bool, "array[2]":bool, "array[3]":bool, "array[4]":bool, "array[5]":bool, "array[6]":bool, "array[7]":bool, "array[8]":bool, "array[9]":bool, "array[10]":bool, "array[11]":bool, "array[12]":bool, "array[13]":bool, "array[14]":bool, "array[15]":bool}
  T93 = cluster{"Contour Type":u32, "ROI Type":u32, "Points":i32[]}[]
  T94 = cluster{"Active rules[0]":bool, "Active rules[1]":bool, "Active rules[2]":bool, "Active rules[3]":bool, "Active rules[4]":bool, "Active rules[5]":bool, "Active rules[6]":bool, "Active rules[7]":bool, "Active rules[8]":bool}
  T95 = typedef "eventvkey.ctl" = enum16{"ASCII", "Enter", "Return", "Shift", "Ctrl", "Alt", "Cmd", "Opt", "Caps", "NumLock", "Clear", "Break", "Up", "Down", "Left", "Right", "Insert", "Delete", "Home", "End", "PageUp", "PageDown", "Escape", "Help", "Pause", "ScrollLock", "F1", "F2", "F3", "F4", "F5", "F6", "F7", "F8", "F9", "F10", "F11", "F12", "F13", "F14", "F15", "F16", "F17", "F18", "F19", "F20", "F21", "F22", "F23", "F24", "Play", "VolumeUp", "VolumeDown", "Mute", "Two Byte Char"}
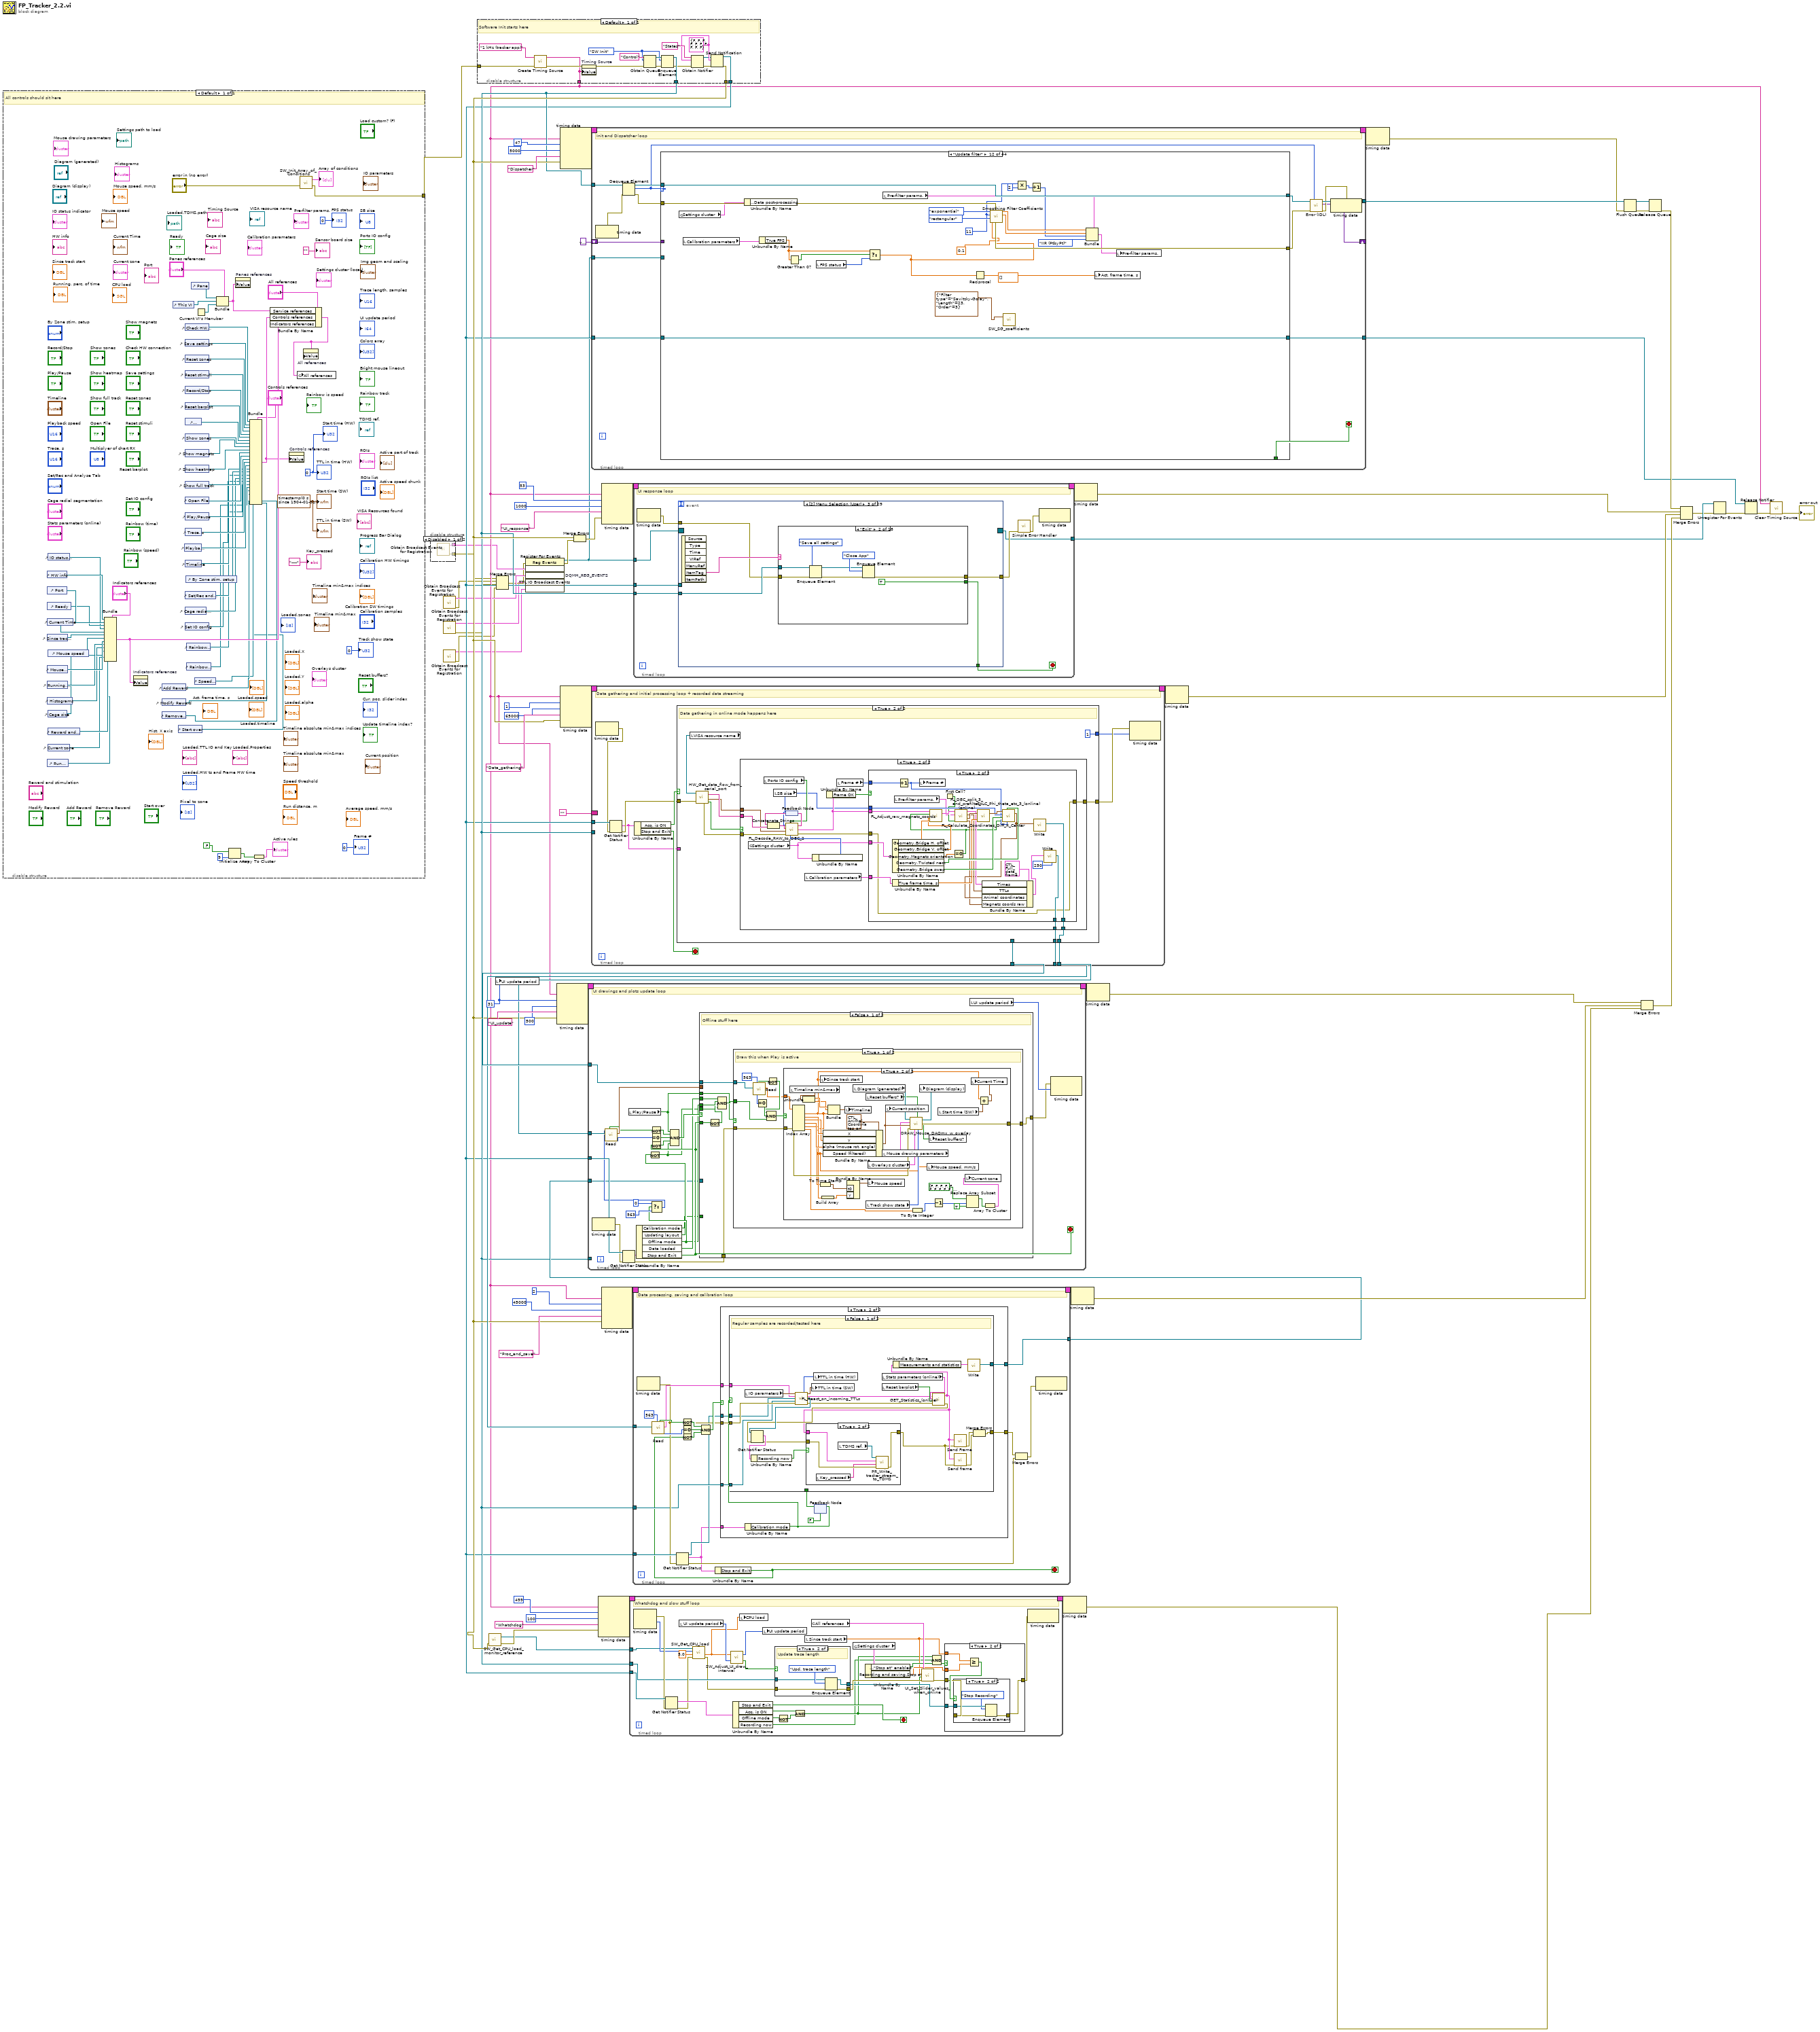
[diagram p0: block diagram]
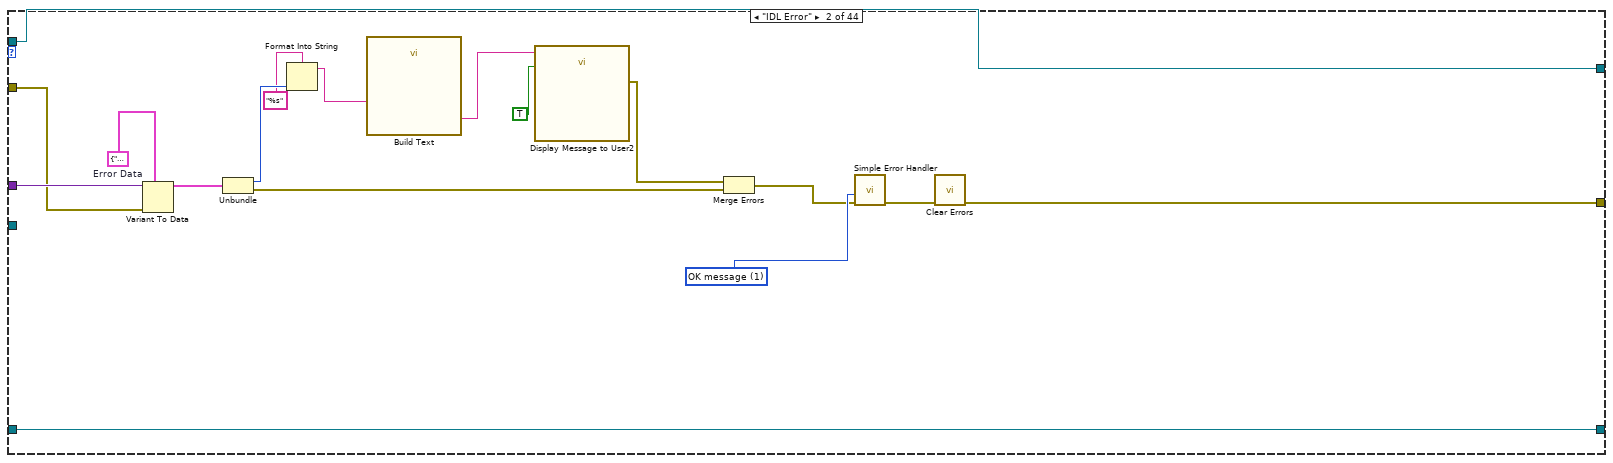
[diagram p4: hidden frame]
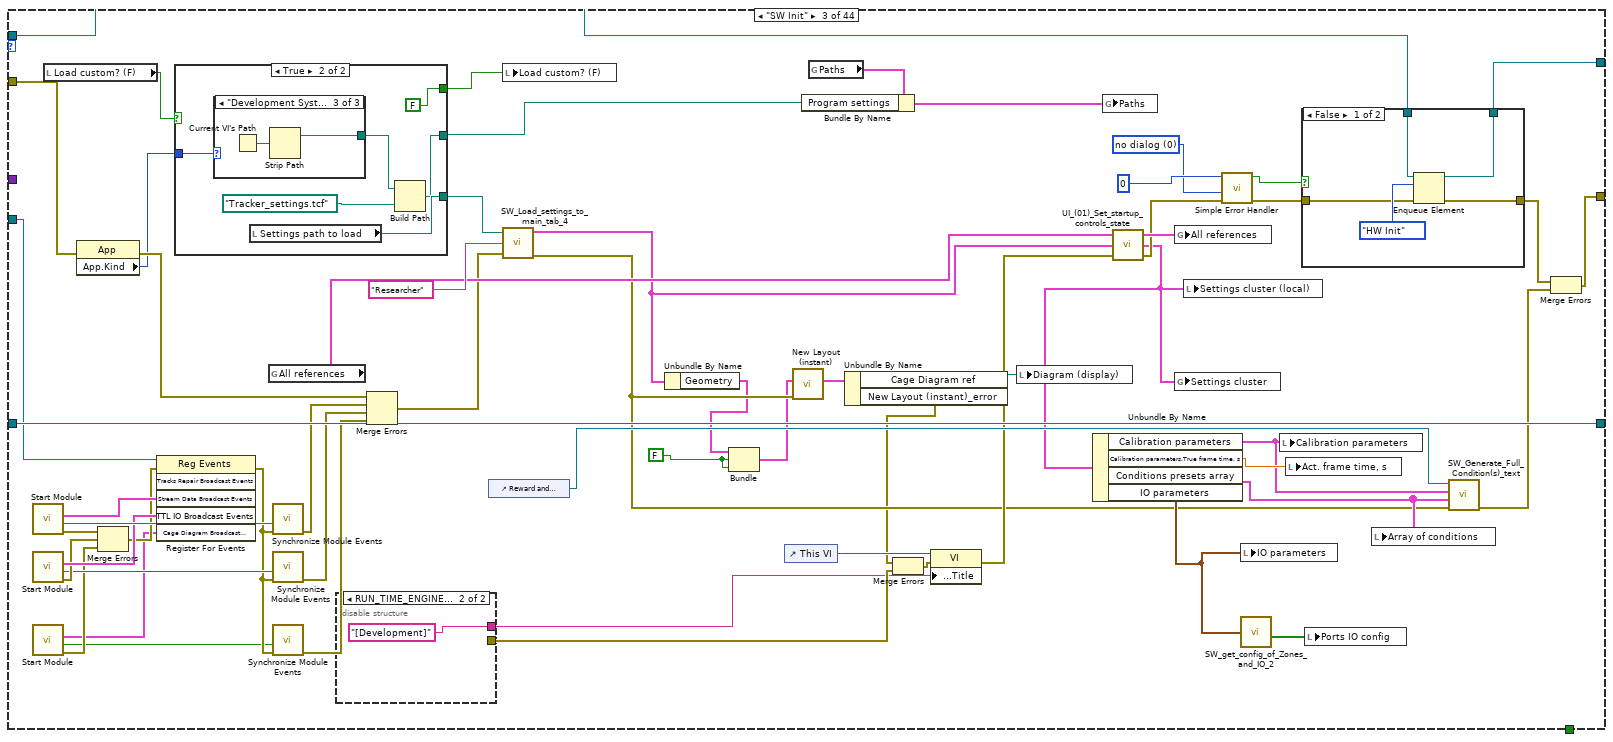
[diagram p5: hidden frame]
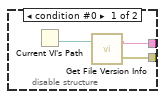
[diagram p6: hidden frame]
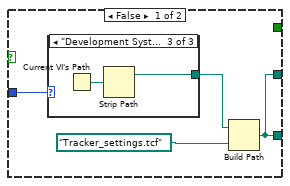
[diagram p7: hidden frame]
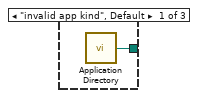
[diagram p8: hidden frame]
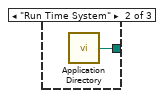
[diagram p9: hidden frame]
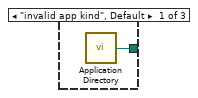
[diagram p10: hidden frame]
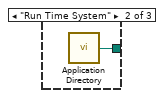
[diagram p11: hidden frame]
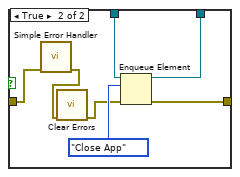
[diagram p12: hidden frame]
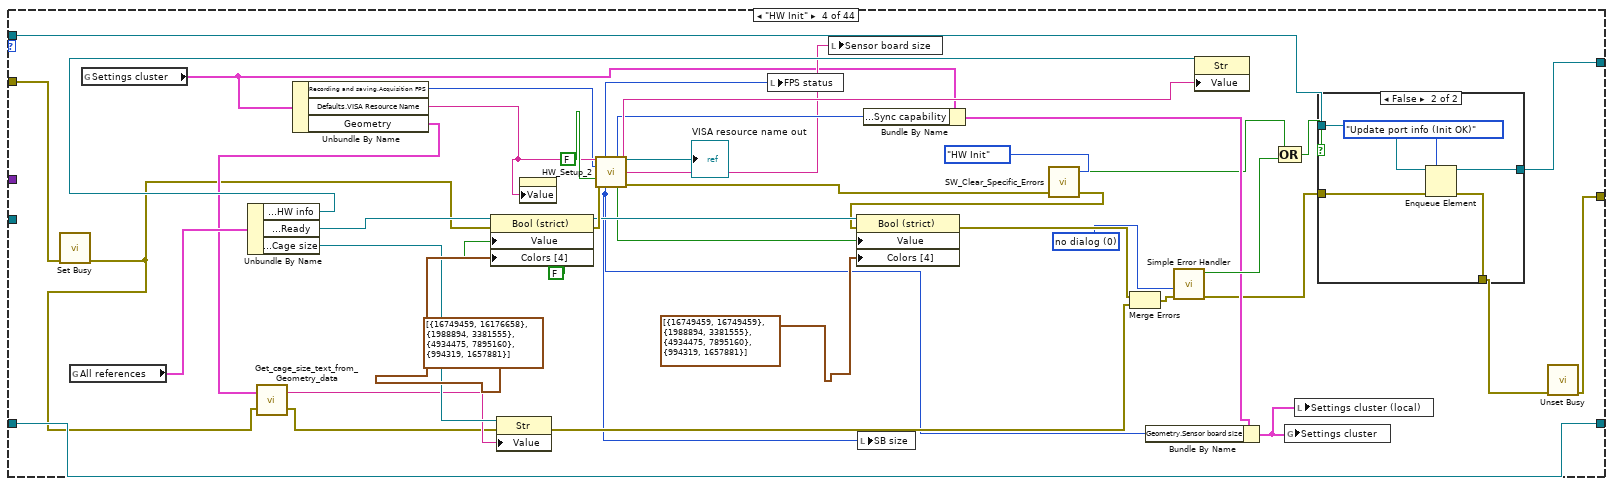
[diagram p13: hidden frame]
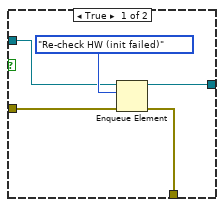
[diagram p14: hidden frame]
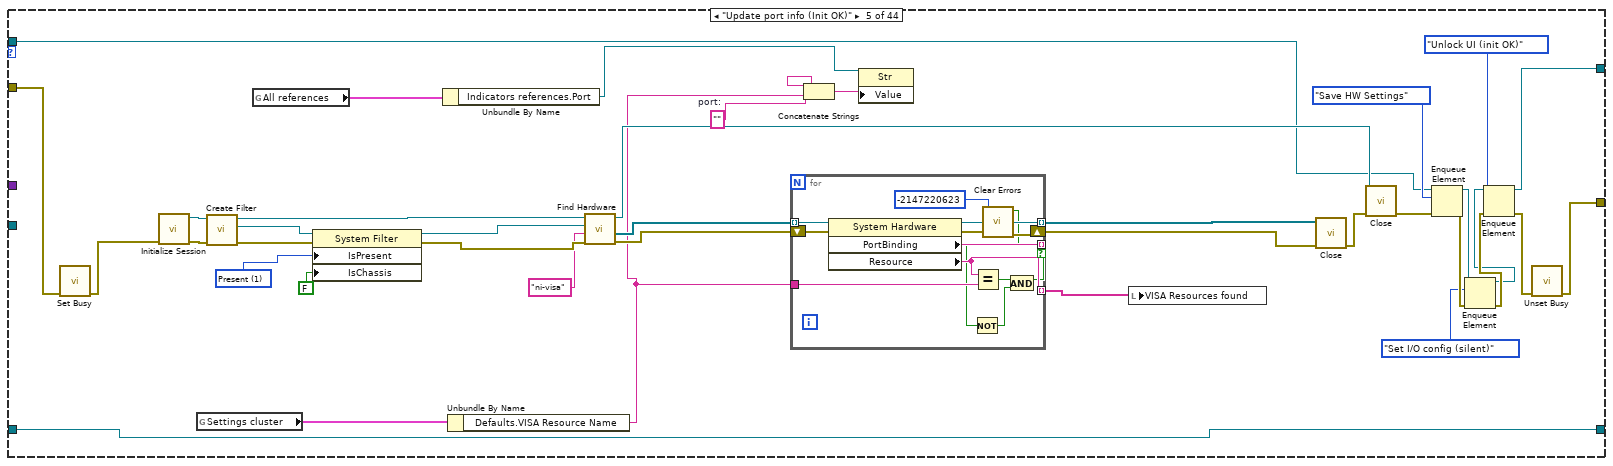
[diagram p15: hidden frame]
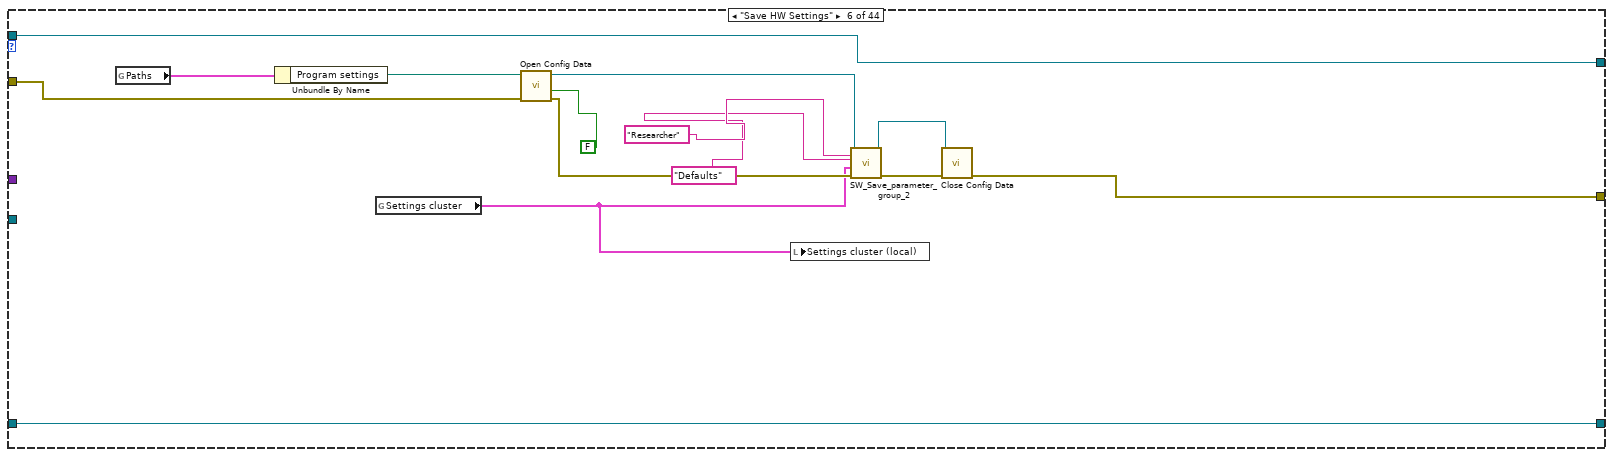
[diagram p16: hidden frame]
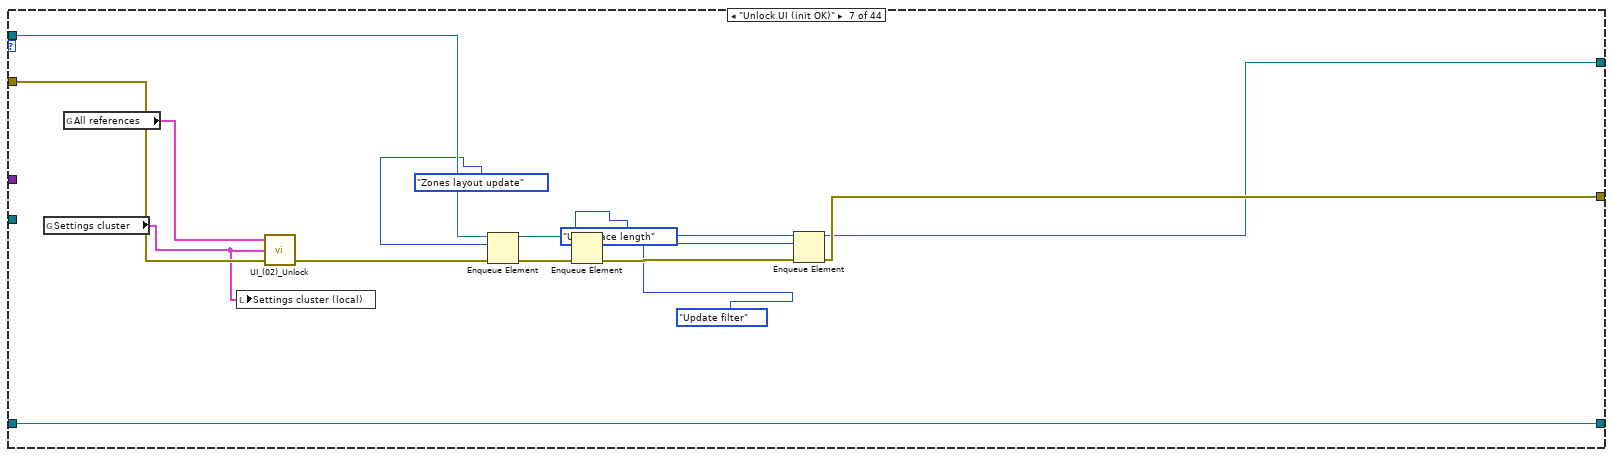
[diagram p17: hidden frame]
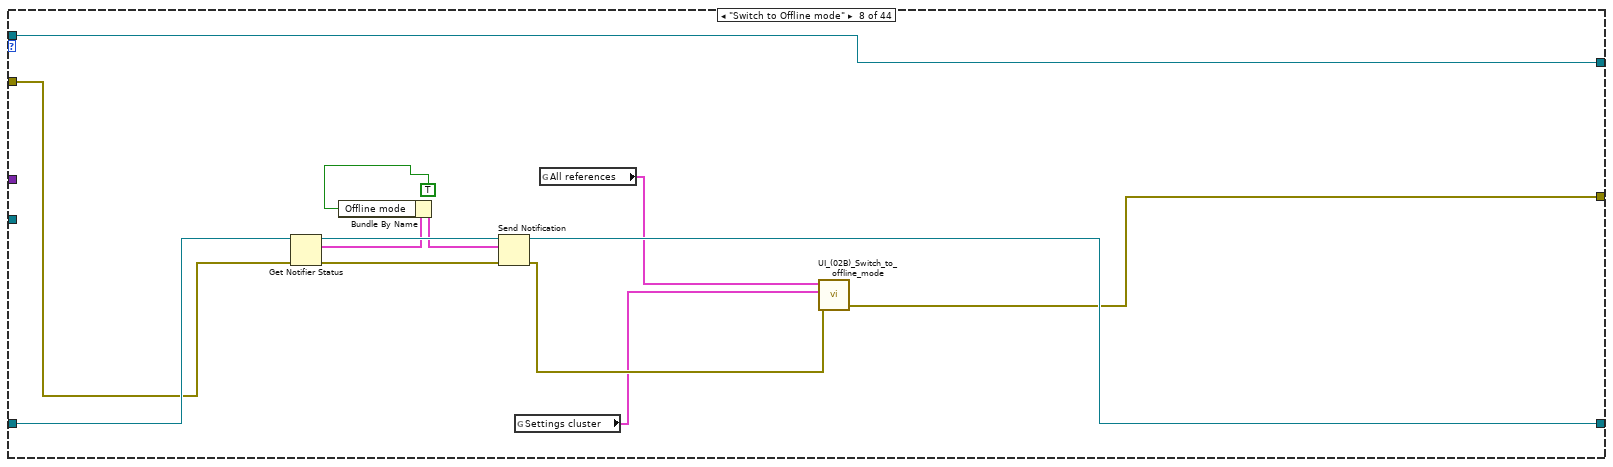
[diagram p18: hidden frame]
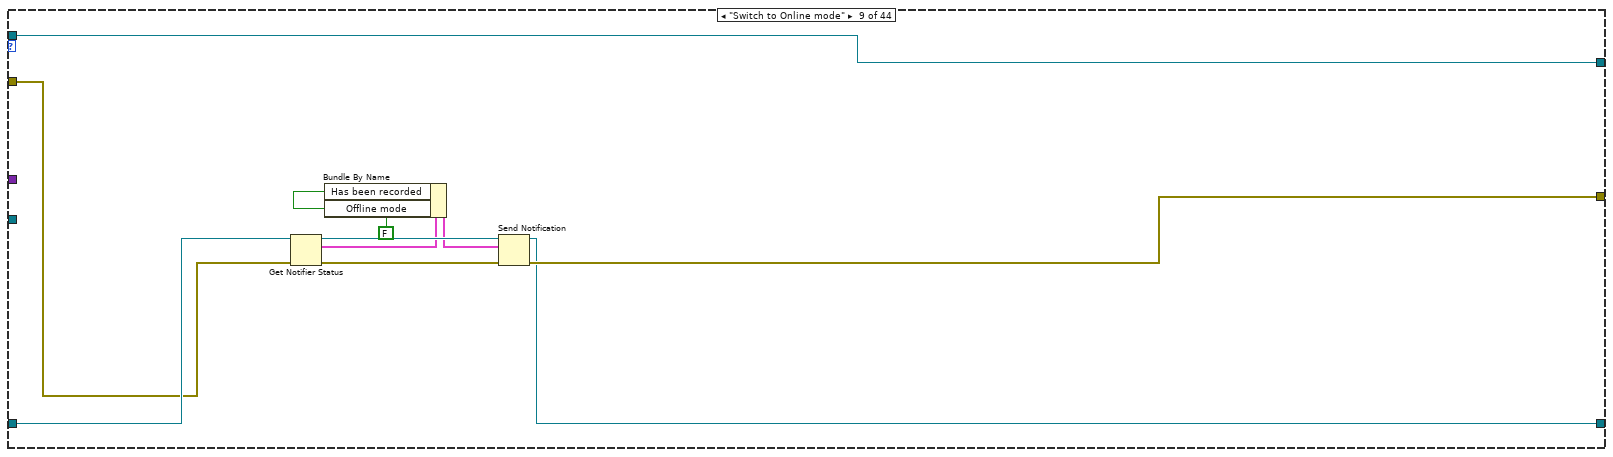
[diagram p19: hidden frame]
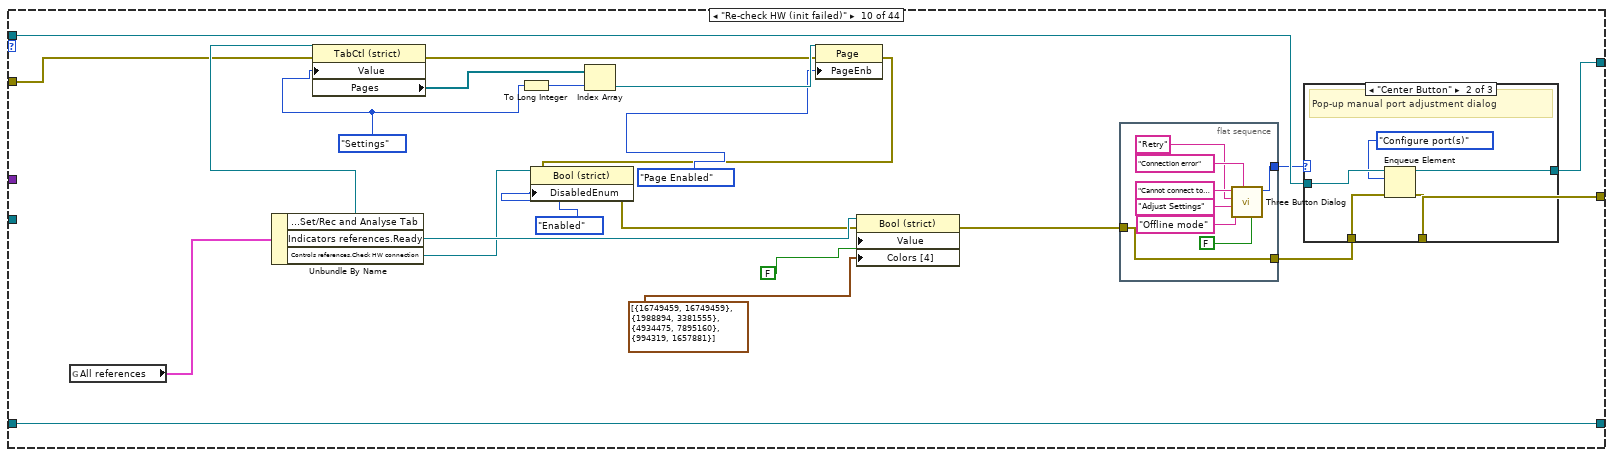
[diagram p20: hidden frame]
diagram:
  w50 = i64 31 ("Period")
  n1 = disable-structure shown="Default" {
    disable-tunnel: [w85] -> w4
    frame Enabled {
      w97 = timestamp(0 s since 1904-01-01) ("Start time (SW)")
      w96 = u32 0 ("TTL in time (HW)")
      # "All controls should sit here"
      n2 = control-ref of="Since track start"() -> (w118:refnum<vi>)
      n3 = control-ref of="Mouse speed, mm/s"() -> (w117:refnum<vi>)
      n4 = control-ref of="Running, perc. of time"() -> (w116:refnum<vi>)
      n5 = control-ref of="Histograms"() -> (w83:refnum<vi>)
      n6 = control-ref of="HW info"() -> (w122:refnum<vi>)
      n7 = control-ref of="Port"() -> (w121:refnum<vi>)
      n8 = control-ref of="Ready"() -> (w120:refnum<vi>)
      n9 = control-ref of="Current Time"() -> (w119:refnum<vi>)
      n10 = control-ref of="Run distance, m"() -> (w82:refnum<vi>)
      n11 = control-ref of="Cage size"() -> (w104:refnum<vi>)
      n12 = control-ref of="Reward and stimulation"() -> (w87:refnum<vi>)
      n13 = control-ref of="Current zone"() -> (w84:refnum<vi>)
      n14 = control-ref of="IO status indicator"() -> (w112:refnum<vi>)
      n15 = control-ref of="Mouse speed"() -> (w80:refnum<vi>)
      n16 = Bundle(cluster="Indicators references", "HW info"=w122, "Port"=w121, "Ready"=w120, "IO status indicator"=w112, "Current Time"=w119, "Record timestamp"=w118, "Mouse speed"=w80, "Mouse speed, mm/s"=w117, "Running, perc. of time"=w116, "Histograms"=w83, "Cage size"=w104, "Reward"=w87, "Current zone"=w84, "Run length, m"=w82) -> (w109:T34)
      n17 = property on="Indicators references" class="Clust (strict)"("Value"=w109) -> ()  [unwired: 2 in, 2 out]
      n18 = control-ref of="Add Reward"() -> (w90:refnum<vi>)
      n19 = control-ref of="Modify Reward"() -> (w89:refnum<vi>)
      n20 = control-ref of="Remove Reward"() -> (w88:refnum<vi>)
      n21 = control-ref of="This VI"() -> (w114:refnum<vi>)
      n22 = control-ref of="Start over"() -> (w79:refnum<vi>)
      n23 = control-ref of="Playback speed"() -> (w125:refnum<vi>)
      n24 = control-ref of="Check HW connection"() -> (w138:refnum<vi>)
      n25 = control-ref of="Save settings"() -> (w137:refnum<vi>)
      n26 = control-ref of="Reset zones"() -> (w136:refnum<vi>)
      n27 = control-ref of="Reset stimuli"() -> (w135:refnum<vi>)
      n28 = control-ref of="Record/Stop"() -> (w134:refnum<vi>)
      n29 = control-ref of="Reset barplot"() -> (w133:refnum<vi>)
      n30 = control-ref of="Multiplyer of chart RX"() -> (w132:refnum<vi>)
      n31 = control-ref of="Show zones"() -> (w131:refnum<vi>)
      n32 = control-ref of="Show magnets"() -> (w113:refnum<vi>)
      n33 = control-ref of="Show heatmap"() -> (w130:refnum<vi>)
      n34 = control-ref of="Show full track"() -> (w129:refnum<vi>)
      n35 = control-ref of="Open File"() -> (w128:refnum<vi>)
      n36 = control-ref of="Play/Pause"() -> (w127:refnum<vi>)
      n37 = control-ref of="Trace, s"() -> (w126:refnum<vi>)
      n38 = control-ref of="Timeline"() -> (w124:refnum<vi>)
      n39 = control-ref of="Cage radial segmentation"() -> (w106:refnum<vi>)
      n40 = control-ref of="Set IO config"() -> (w105:refnum<vi>)
      n41 = control-ref of="Set/Rec and Analyse Tab"() -> (w107:refnum<vi>)
      n42 = control-ref of="By Zone stim. setup"() -> (w123:refnum<vi>)
      n43 = control-ref of="Rainbow (time)"() -> (w102:refnum<vi>)
      n44 = control-ref of="Rainbow (speed)"() -> (w101:refnum<vi>)
      n45 = control-ref of="Pane"() -> (w115:refnum<vi>)
      n46 = control-ref of="Speed threshold"() -> (w81:refnum<vi>)
      n47 = Current VI's Menubar() -> (w103:refnum<k9>)
      n48 = Bundle(cluster="Panes references", "Pane"=w115, "This VI"=w114, "Menu"=w103) -> (w110:T33)
      n49 = Initialize Array(FALSE ("Activation"), 9 ("dimension size")) -> (w74:bool[])
      n50 = property on="Panes references" class="Clust (strict)"("Value"=w110) -> ()  [unwired: 2 in, 2 out]
      n51 = Bundle(cluster="Controls references", "Check HW connection"=w138, "Save settings"=w137, "Reset zones"=w136, "Reset stimuli"=w135, "Record/Stop"=w134, "Reset barplot"=w133, "Multiplyer of chart RX"=w132, "Show zones"=w131, "Show magnets"=w113, "Show heatmap"=w130, "Show full track"=w129, "Open File"=w128, "Play/Pause"=w127, "Trace, s"=w126, "Playback speed"=w125, "Timeline"=w124, "By Zone stim. setup"=w123, "Set/Rec and Analyse Tab"=w107, "Cage radial segmentation"=w106, "Set IO config"=w105, "Rainbow (time)"=w102, "Rainbow (speed)"=w101, "Add Reward"=w90, "Modify Reward"=w89, "Delete Reward"=w88, "Speed threshold, mm/s"=w81, "Start Over"=w79) -> (w94:T35)
      n52 = Array To Cluster(array=w74) -> (cluster=→"Active rules":T40)
      n53 = Bundle By Name(cluster="All references", "Service references"=w110, "Controls references"=w94, "Indicators references"=w109) -> (w108:T36)
      n54 = property on="Controls references" class="Clust (strict)"("Value"=w94) -> ()  [unwired: 2 in, 2 out]
      n55 = global write "SW_Globals_2.2+.vi" "All references"(w108) -> ()
      n56 = call "SW_Init_Array_of_Conditions.vi"("error in (no error)"="error in (no error)") -> ("error out"=w85:T41, "Array of conditions"=→"Array of conditions":T6)  [unwired: 1 in]
      n57 = property on="All references" class="Clust (strict)"("Value"=w108) -> ()  [unwired: 2 in, 2 out]
      "FPS status" <- 0 ("FPS status")
      "Sensor board size" <- "" ("Sensor board size")
      "Start time (SW)" <- w97
      "TTL in time (SW)" <- w97
      "Key_pressed" <- "----" ("Key_pressed")
      "TTL in time (HW)" <- w96
      "Start time (HW)" <- w96
      "Track show state" <- u32 0 ("Track show state")
      "Frame #" <- u32 0 ("Frame #")
    }
  }
  n58 = disable-structure shown="Disabled" {
    disable-tunnel: [w140 _] -> w16
    disable-tunnel: [w139 _] -> w15
    frame Disabled {
      n59 = call "Obtain Broadcast Events for Registration.vi"() -> ("error out"=w139:errorcluster, "Tracks Repair Broadcast Events"=w140:T42)  [unwired: 9 in, 1 out]
    }
    frame Enabled {
    }
  }
  n60 = call "Obtain Broadcast Events for Registration.vi"() -> ("error out"=w7:errorcluster, "Stream Data Broadcast Events"=w9:T43)  [unwired: 9 in, 1 out]
  n61 = call "Obtain Broadcast Events for Registration.vi"() -> ("error out"=w5:errorcluster, "TTL IO Broadcast Events"=w6:T44)  [unwired: 9 in, 1 out]
  n62 = call "Obtain Broadcast Events for Registration.vi"() -> ("error out"=w2:errorcluster, "Cage Diagram Broadcast Events"=w1:T45)  [unwired: 9 in, 1 out]
  n63 = disable-structure shown="Default" {
    disable-tunnel: w4 -> [w150]
    disable-tunnel: [w149] -> w23
    disable-tunnel: [w148] -> w19
    disable-tunnel: [w142] -> w22
    disable-tunnel: [w141] -> w24
    frame Enabled {
      w144 = T46 {"Acq. is ON"=FALSE, "Playing loaded"=FALSE, "Recording now"=FALSE, "Has been recorded"=FALSE, "Data saved"=FALSE, "Data loaded"=FALSE, "Calibration mode"=FALSE, "Offline mode"=FALSE, "Stop and Exit"=FALSE, "Updating layout"=FALSE} ("States cluster")
      w151 = CTL_Control_States."SW Init"
      # "Software Init starts here"
      n64 = call-poly <vilib>:"Create Timing Source.vi"("error in (no error)"=w150, "name (in)"="1 kHz (tracker app)") -> ("error out"=w157:errorcluster, "name (out)"=w148:string)  [unwired: 8 in]
      n65 = property on="Timing Source" class="Str"(error in=w157, "Value"=w148) -> (error out=w155:errorcluster)  [unwired: 1 in, 1 out]
      n66 = Obtain Queue(name (unnamed)="Control", element data type=w151, error in (no error)=w155) -> (queue out=w152:refnum<queue>, error out=w153:errorcluster)  [unwired: 2 in, 1 out]
      n67 = Enqueue Element(queue=w152, element=w151, error in (no error)=w153) -> (queue out=w149:refnum<queue>, error out=w147:errorcluster)  [unwired: 1 in, 1 out]
      n68 = Obtain Notifier(name (unnamed)="States", notification data type=w144, error in (no error)=w147) -> (notifier out=w143:refnum<notifier>, error out=w145:errorcluster)  [unwired: 1 in, 1 out]
      n69 = Send Notification(notification=w144, notifier=w143, error in (no error)=w145) -> (notifier out=w142:refnum<notifier>, error out=w141:errorcluster)
    }
  }
  n70 = call "SW_Get_CPU_load_monitor_reference.vi"("error in (no error)"=w24) -> ("error out"=w37:errorcluster, "CPU monitor .NET reference"=w36:refnum<k24>)  [unwired: 1 in]
  n71 = local write "UI update period"(w50) -> ()
  n72 = Merge Errors(w15, w7, w5, w2) -> (w8:errorcluster)
  n73 = register-events "DQMH_REG_EVENTS"(error in=w8, w16, w9, w6, w1) -> (reference out=w13:refnum<event-registration>, error out=w14:errorcluster)  [unwired: 1 in]
  n74 = node-c288(w19, w50, 500 ("Priority"), "UI_update" ("Structure Name"), w24) -> (w54:T48)
  n75 = node-c288(w19, i64 47 ("Period"), 5000 ("Priority"), "Dispatcher" ("Structure Name"), w24) -> (w72:T48)
  n76 = node-c288(w19, i64 1 ("Period"), 65000 ("Priority"), "Data_gathering" ("Structure Name"), w24) -> (w60:T48)
  n77 = Merge Errors(w24, w14) -> (w17:errorcluster)
  n78 = timed-loop {
    timing: w72 -> [_]
    timing-out: [_] -> w71
    tunnel: w23 -> [w172]
    tunnel: [w166] -> w67
    tunnel: w22 -> [w169]
    tunnel: [w168] -> w44
    shift-right: [w162] -> _
    shift-left: variant ("Error data") -> [w159]
    tunnel: w13 -> [w158]
    stop <- w170 stop-if-true
    # "Init and Dispatcher loop"
    n79 = node-c288() -> (w161:errorcluster)  [unwired: 1 in]
    n80 = Dequeue Element(queue=w172, error in (no error)=w161) -> (queue out=w171:refnum<queue>, element=w163:T47, error out=w160:errorcluster)  [unwired: 1 in, 1 out]
    n81 = case shown="\"Update filter\"" w163 {
      tunnel: [w175 w191 w242 w314 w353 w393 w408 w431 w441 w456 w504 w534 w586 w597 w630 w674 w715 w761 w791 w833 w881 w902 w961 w1052 w1092 w1192 w1234 w1277 w1345 w1358 w1407 w1487 w1518 w1574 w1583 w1608 w1655 w1665 w1691 w1707 w1736 w1768 w1785 w1834] -> w167
      tunnel: w171 -> [w175 w191 w231 w315 w354 w393 w415 w431 w441 w457 w505 w534 w586 w598 w630 w669 w715 w761 w791 w834 w880 w903 w962 w1053 w1093 w1193 w1235 w1278 w1345 w1359 w1426 w1487 w1519 w1574 w1583 w1609 w1655 w1666 w1692 w1708 w1736 w1768 w1785 w1834]
      tunnel: [_ _ _ _ _ _ _ _ _ _ _ _ _ _ _ _ _ _ _ _ _ _ _ _ _ _ _ _ _ _ _ _ _ _ _ _ _ _ _ _ _ _ _ TRUE] -> w170
      tunnel: [w174 w181 w233 w321 w375 w394 w409 w421 w436 w455 w503 w535 w566 w595 w629 w662 w711 w760 w786 w832 w879 w904 w958 w1054 w1094 w1194 w1236 w1279 w1343 w1357 w1408 w1451 w1521 w1572 w1586 w1612 w1649 w1664 w1683 w1709 w1727 w1765 w1782 w1807] -> w165
      tunnel: w160 -> [w174 w188 w239 w322 w376 w399 w418 w429 w439 w450 w498 w535 w572 w607 w642 w676 w716 w762 w792 w839 w877 w908 w966 w1058 w1098 w1198 w1240 w1292 w1344 w1373 w1439 w1457 w1529 w1575 w1589 w1615 w1654 w1674 w1699 w1718 w1734 w1761 w1783 w1815]
      tunnel: w169 -> [w173 w192 w238 w303 w357 w403 w405 w430 w440 w445 w493 w532 w581 w594 w634 w670 w717 w763 w793 w840 w872 w909 w967 w1059 w1099 w1199 w1241 w1286 w1346 w1367 w1406 w1477 w1530 w1554 w1590 w1616 w1656 w1675 w1700 w1724 w1728 w1762 w1779 w1826]
      tunnel: [w173 w192 w238 w303 w357 w403 w405 w426 w435 w445 w493 w532 w565 w594 w634 w670 w712 w756 w787 w835 w873 w905 w963 w1055 w1095 w1195 w1237 w1286 w1346 w1367 w1406 w1477 w1520 w1554 w1585 w1611 w1656 w1675 w1700 w1724 w1728 w1762 w1779 w1819] -> w168
      tunnel: w159 -> [_ w189 _ _ _ _ _ _ _ _ _ _ _ _ _ _ _ _ _ _ _ _ _ _ _ _ _ _ _ _ _ _ _ _ _ _ _ _ _ _ _ _ _ _]
      tunnel: w158 -> [_ _ w222 _ _ _ _ _ _ _ _ _ _ _ _ _ _ _ _ _ _ _ _ _ _ _ _ _ w1342 _ _ _ _ _ _ _ _ _ _ _ _ _ _ _]
      frame Default {
      }
      frame "IDL Error" {
        w185 = T59 1 items=["no dialog", "OK message", "continue or stop message", "OK message + warnings", "continue/stop + warnings"] ("type of dialog (OK msg:1)")
        w190 = T60 {"Previous step"=enum."SW Init", "error IO"={"status"=FALSE, "code"=0, "source"=""}}  # Error Data
        n82 = Variant To Data(error in=w188, type=w190, Variant=w189) -> (data=w187:T60)  [unwired: 1 out]
        n83 = Unbundle(w187) -> ("Previous step"=w184:T47, "error IO"=w186:errorcluster)
        n84 = Format Into String(format string="%s", w184) -> (resulting string=w180:string)  [unwired: 2 in, 1 out]
        n85 = call "Build Text"("stage"=w180) -> ("Result"=w179:string)  [unwired: 13 in, 1 out]
        n86 = call "Display Message to User2"("Enable"=TRUE, "Message"=w179) -> ("error out"=w176:errorcluster)  [unwired: 8 in, 1 out]
        n87 = Merge Errors(w176, w186) -> (w177:errorcluster)
        n88 = call <vilib>:"Simple Error Handler.vi"("type of dialog (OK msg:1)"=w185, "error in (no error)"=w177) -> ("error out"=w182:errorcluster)  [unwired: 3 in, 4 out]
        n89 = call <vilib>:"Clear Errors.vi"("error in (no error)"=w182) -> ("error out"=w181:errorcluster)  [unwired: 5 in, 1 out]
      }
      frame "SW Init" {
        w198 = FALSE
        w244 = T59 0 items=["no dialog", "OK message", "continue or stop message", "OK message + warnings", "continue/stop + warnings"] ("type of dialog (OK msg:1)")
        n90 = call "Start Module.vi"() -> ("error out"=w218:errorcluster, "Wait for Event Sync?"=w219:bool, "Stream Data Broadcast Events"=w220:T43)  [unwired: 8 in, 1 out]
        n91 = call "Start Module.vi"() -> ("error out"=w214:errorcluster, "Wait for Event Sync?"=w213:bool, "TTL IO Broadcast Events"=w216:T44)  [unwired: 8 in, 1 out]
        n92 = call "Start Module.vi"() -> ("error out"=w209:errorcluster, "Wait for Event Sync?"=w206:bool, "Cage Diagram Broadcast Events"=w208:T45)  [unwired: 8 in, 1 out]
        n93 = local read "Load custom? (F)"() -> (w197:bool)
        n94 = property class="App"(error in=w239) -> (error out=w250:errorcluster, "App.Kind"=w246:T61)  [unwired: 1 in, 1 out]
        n95 = Merge Errors(w218, w214, w209) -> (w215:errorcluster)
        n96 = register-events(reference=w222, error in=w215, w220, w216, w208) -> (error out=w207:errorcluster)  [unwired: 1 in, 1 out]
        n97 = case shown="True" w197 {
          tunnel: [w256 w265] -> w230
          tunnel: w246 -> [w258 w268]
          tunnel: [_ FALSE] -> w196
          tunnel: [w256 w264] -> w195
          frame False {
            n98 = case shown="\"Development System\"" w258 {
              tunnel: [w260 w261 w262] -> w259
              frame "invalid app kind", Default {
                n99 = call <vilib>:"Application Directory.vi"() -> ("Application Directory"=w260:path)
              }
              frame "Run Time System" {
                n100 = call <vilib>:"Application Directory.vi"() -> ("Application Directory"=w261:path)
              }
              frame "Development System" {
                n101 = Current VI's Path() -> (path=w263:path)
                n102 = Strip Path(path=w263) -> (stripped path=w262:path)  [unwired: 1 out]
              }
            }
            n103 = Build Path(base path=w259, name or relative path=path "Tracker_settings.tcf") -> (appended path=w256:path)
          }
          frame True {
            n104 = case shown="\"Development System\"" w268 {
              tunnel: [w270 w271 w272] -> w269
              frame "invalid app kind", Default {
                n105 = call <vilib>:"Application Directory.vi"() -> ("Application Directory"=w270:path)
              }
              frame "Run Time System" {
                n106 = call <vilib>:"Application Directory.vi"() -> ("Application Directory"=w271:path)
              }
              frame "Development System" {
                n107 = Current VI's Path() -> (path=w273:path)
                n108 = Strip Path(path=w273) -> (stripped path=w272:path)  [unwired: 1 out]
              }
            }
            n109 = local read "Settings path to load"() -> (w265:path)
            n110 = Build Path(base path=w269, name or relative path=path "Tracker_settings.tcf") -> (appended path=w264:path)
          }
        }
        n111 = global read "SW_Globals_2.2+.vi" "All references"() -> (w236:T36)
        n112 = call "Synchronize Module Events.vi"("error in (no error)"=w207, "Wait for Event Sync?"=w219) -> ("error out"=w217:errorcluster)  [unwired: 9 in]
        n113 = call "Synchronize Module Events.vi"("error in (no error)"=w207, "Wait for Event Sync?"=w213) -> ("error out"=w212:errorcluster)  [unwired: 9 in]
        n114 = call "Synchronize Module Events.vi"("error in (no error)"=w207, "Wait for Event Sync?"=w206) -> ("error out"=w205:errorcluster)  [unwired: 9 in]
        n115 = disable-structure shown="RUN_TIME_ENGINE==False" {
          disable-tunnel: [w254 "[Development]" ("App Version Info")] -> w193
          disable-tunnel: [w253 _] -> w223
          frame condition #0 {
            n116 = Current VI's Path() -> (path=w252:path)
            n117 = call "Get File Version Info.vi"("File path"=w252) -> ("error out"=w253:errorcluster, "File Version"=w254:string)  [unwired: 1 in]
          }
          frame condition #1 (active) {
          }
        }
        n118 = Merge Errors(w250, w217, w212, w205) -> (w221:errorcluster)
        n119 = control-ref of="Reward and stimulation"() -> (w234:refnum<vi>)
        n120 = local write "Load custom? (F)"(w196) -> ()
        n121 = call "SW_Load_settings_to_main_tab_4.vi"("Settings path in"=w230, "Researcher name"="Researcher", "error in (no error)"=w221) -> ("Settings cluster out"=w200:T16, "Error Out"=w204:errorcluster)  [unwired: 5 in, 1 out]
        n122 = Unbundle By Name(w200) -> ("Geometry"=w194:T19)
        n123 = Bundle("Geometry"=w194, w198, w198) -> (w199:cluster{"Geometry":T19, bool, bool})  [unwired: 1 in]
        n124 = control-ref of="This VI"() -> (w226:refnum<vi>)
        n125 = call "New Layout (instant).vi"("error in (no error)"=w204, "Cage parameters"=w199) -> ("Reply Payload"=w203:T62)  [unwired: 7 in, 2 out]
        n126 = global read "SW_Globals_2.2+.vi" "Paths"() -> (w249:T68)
        n127 = Bundle By Name(cluster=w249, "Program settings"=w195) -> (w248:T68)
        n128 = Unbundle By Name(w203) -> ("Cage Diagram ref"=w202:T15, "New Layout (instant)_error"=w201:errorcluster)
        n129 = Merge Errors(w201, w223) -> (w224:errorcluster)
        n130 = property class="VI"(reference=w226, error in=w224, "Front Panel.Title"=w193) -> (error out=w225:errorcluster)  [unwired: 1 out]
        n131 = local write "Diagram (display)"(w202) -> ()
        n132 = global write "SW_Globals_2.2+.vi" "Paths"(w248) -> ()
        n133 = call "UI_(01)_Set_startup_controls_state.vi"("error in (no error)"=w225, "Settings cluster in"=w200, "All references in"=w236) -> ("error out"=w227:errorcluster, "Settings cluster out"=w211:T16, "All references out"=w251:T36)
        n134 = Unbundle By Name(w211) -> ("Calibration parameters"=w235:T23, "Calibration parameters.True frame time, s"=w237:dbl, "Conditions presets array"=w232:T6, "IO parameters"=w228:T22)
        n135 = global write "SW_Globals_2.2+.vi" "All references"(w251) -> ()
        n136 = global write "SW_Globals_2.2+.vi" "Settings cluster"(w211) -> ()
        n137 = local write "Settings cluster (local)"(w211) -> ()
        n138 = call <vilib>:"Simple Error Handler.vi"("error code (no error:0)"=0, "type of dialog (OK msg:1)"=w244, "error in (no error)"=w227) -> ("error?"=w243:bool, "error out"=w241:errorcluster)  [unwired: 2 in, 3 out]
        n139 = local write "IO parameters"(w228) -> ()
        n140 = call "SW_get_config_of_Zones_and_IO_2.vi"("Sync parameters cluster input"=w228) -> ("Ports IO config (OUT is FALSE)"=w229:bool[])  [unwired: 3 out]
        n141 = local write "Calibration parameters"(w235) -> ()
        n142 = local write "Act. frame time, s"(w237) -> ()
        n143 = case shown="False" w243 {
          tunnel: w231 -> [w278 w285]
          tunnel: [w277 w284] -> w242
          tunnel: w241 -> [w275 w281]
          tunnel: [w274 w282] -> w240
          frame False {
            n144 = Enqueue Element(queue=w278, element=CTL_Control_States."HW Init", error in (no error)=w275) -> (queue out=w277:refnum<queue>, error out=w274:errorcluster)  [unwired: 1 in, 1 out]
          }
          frame True {
            n145 = call <vilib>:"Simple Error Handler.vi"("error in (no error)"=w281) -> ("error out"=w280:errorcluster)  [unwired: 4 in, 4 out]
            n146 = call <vilib>:"Clear Errors.vi"("error in (no error)"=w280) -> ("error out"=w279:errorcluster)  [unwired: 5 in, 1 out]
            n147 = Enqueue Element(queue=w285, element=CTL_Control_States."Close App", error in (no error)=w279) -> (queue out=w284:refnum<queue>, error out=w282:errorcluster)  [unwired: 1 in, 1 out]
          }
        }
        n148 = local write "Ports IO config"(w229) -> ()
        n149 = local write "Array of conditions"(w232) -> ()
        n150 = call "SW_Generate_Full_Condition(s)_text.vi"("error in (no error)"=w204, "Array of conditions in"=w232, "Calibration parameters"=w235, "TreeControl ref in"=w234) -> ("error out"=w210:errorcluster)  [unwired: 6 in, 1 out]
        n151 = Merge Errors(w240, w210) -> (w233:errorcluster)
      }
      frame "HW Init" {
        w310 = T59 0 items=["no dialog", "OK message", "continue or stop message", "OK message + warnings", "continue/stop + warnings"] ("type of dialog (OK msg:1)")
        n152 = call <vilib>:"Set Busy.vi"("error in (no error)"=w322) -> ("error out"=w287:errorcluster)  [unwired: 9 in, 1 out]
        n153 = global read "SW_Globals_2.2+.vi" "All references"() -> (w328:T36)
        n154 = global read "SW_Globals_2.2+.vi" "Settings cluster"() -> (w296:T16)
        n155 = Unbundle By Name(w328) -> ("Indicators references.HW info"=w327:refnum<vi>, "Indicators references.Ready"=w325:refnum<vi>, "Indicators references.Cage size"=w308:refnum<vi>)
        n156 = Unbundle By Name(w296) -> ("Recording and saving.Acquisition FPS"=w301:T18, "Defaults.VISA Resource Name"=w304:string, "Geometry"=w288:T19)
        n157 = call "Get_cage_size_text_from_Geometry_data.vi"("Error In"=w287, "Geometry"=w288) -> ("Error Out"=w286:errorcluster, "Cage size text"=w307:string)
        n158 = property class="Bool (strict)"(reference=w325, error in=w287, "Value"=FALSE, "Colors [4]"=T51 [{"Numeric Control"=16749459, "Numeric Control"=16176658}, {"Numeric Control"=1988894, "Numeric Control"=3381555}, {"Numeric Control"=4934475, "Numeric Control"=7895160}, {"Numeric Control"=994319, "Numeric Control"=1657881}]) -> (reference out=w320:refnum<vi>, error out=w324:errorcluster)
        n159 = property class="Str"(reference=w308, error in=w286, "Value"=w307) -> (error out=w305:errorcluster)  [unwired: 1 out]
        n160 = property on="VISA resource name" class="VISAName"("Value"=w304) -> ()  [unwired: 2 in, 2 out]
        n161 = call "HW_Setup_2.vi"("VISA resource name in"=w304, "Acquisition FPS"=w301, "Close port? (F)"=FALSE, "error in"=w324) -> ("FPS status"=w300:i32, "Sync capability"=w319:u8, "VISA resource name out"=→"VISA resource name out":refnum<visa-resource-name>, "HW information"=w326:string, "Sensor board size"=w299:string, "SB size"=w297:u8, "Instrument OK?"=w312:bool, "error out"=w294:errorcluster)  [unwired: 3 in, 1 out]
        n162 = local write "FPS status"(w300) -> ()
        n163 = local write "Sensor board size"(w299) -> ()
        n164 = local write "SB size"(w297) -> ()
        n165 = Bundle By Name(cluster=w296, "IO parameters.Sync capability"=w319) -> (w298:T16)
        n166 = call "SW_Clear_Specific_Errors.vi"("Error In"=w294, "Code section"=enum16{"Not Specified", "HW Init"}."HW Init") -> ("Error Out"=w293:errorcluster, "specific error cleared?"=w292:bool)  [unwired: 2 in]
        n167 = property class="Bool (strict)"(reference=w320, error in=w293, "Value"=w312, "Colors [4]"=T51 [{"Numeric Control"=16749459, "Numeric Control"=16749459}, {"Numeric Control"=1988894, "Numeric Control"=3381555}, {"Numeric Control"=4934475, "Numeric Control"=7895160}, {"Numeric Control"=994319, "Numeric Control"=1657881}]) -> (error out=w316:errorcluster)  [unwired: 1 out]
        n168 = Merge Errors(w316, w305) -> (w306:errorcluster)
        n169 = Bundle By Name(cluster=w298, "Geometry.Sensor board size"=w297) -> (w289:T16)
        n170 = call <vilib>:"Simple Error Handler.vi"("type of dialog (OK msg:1)"=w310, "error in (no error)"=w306) -> ("error?"=w311:bool, "error out"=w291:errorcluster)  [unwired: 3 in, 3 out]
        n171 = property on="Property Node" class="Str"(reference=w327, "Value"=w326) -> ()  [unwired: 1 in, 2 out]
        n172 = Compound Arithmetic op=OR(w292, w311) -> (w302:bool)
        n173 = global write "SW_Globals_2.2+.vi" "Settings cluster"(w289) -> ()
        n174 = local write "Settings cluster (local)"(w289) -> ()
        n175 = case shown="False" w302 {
          tunnel: [w331 w335] -> w317
          tunnel: w291 -> [w332 w336]
          tunnel: w315 -> [w329 w338]
          tunnel: [w333 w337] -> w314
          frame True {
            n176 = Enqueue Element(queue=w329, element=CTL_Control_States."Re-check HW (init failed)", error in (no error)=w332) -> (queue out=w333:refnum<queue>, error out=w331:errorcluster)  [unwired: 1 in, 1 out]
          }
          frame False {
            n177 = Enqueue Element(queue=w338, element=CTL_Control_States."Update port info (Init OK)", error in (no error)=w336) -> (queue out=w337:refnum<queue>, error out=w335:errorcluster)  [unwired: 1 in, 1 out]
          }
        }
        n178 = call <vilib>:"Unset Busy.vi"("error in (no error)"=w317) -> ("error out"=w321:errorcluster)  [unwired: 10 in]
      }
      frame "Update port info (Init OK)" {
        w360 = ""  # port:
        w372 = 1 items=["Initializing"=-2, "Unknown"=-1, "Not Present"=0, "Present"=1] ("Devices & Chassis:Is Present")
        n179 = call <vilib>:"Set Busy.vi"("error in (no error)"=w376) -> ("error out"=w367:errorcluster)  [unwired: 9 in, 1 out]
        n180 = call <vilib>:"Initialize Session.vi"("error in (no error)"=w367) -> ("error out"=w370:errorcluster, "Session out"=w371:refnum<k21>)  [unwired: 9 in]
        n181 = global read "SW_Globals_2.2+.vi" "Settings cluster"() -> (w347:T16)
        n182 = call <vilib>:"Create Filter.vi"("error in (no error)"=w370, "Session in"=w371) -> ("error out"=w374:errorcluster, "Filter out"=w373:refnum<k20>, "Session out"=w350:refnum<k21>)  [unwired: 7 in]
        n183 = global read "SW_Globals_2.2+.vi" "All references"() -> (w361:T36)
        n184 = property class="System Filter"(reference=w373, error in=w374, "IsPresent"=w372, "IsChassis"=FALSE ("Is Chassis")) -> (reference out=w368:refnum<k20>, error out=w369:errorcluster)
        n185 = Unbundle By Name(w361) -> ("Indicators references.Port"=w359:refnum<vi>)
        n186 = Unbundle By Name(w347) -> ("Defaults.VISA Resource Name"=w346:string)
        n187 = call <vilib>:"Find Hardware.vi"("error in (no error)"=w369, "Experts"="ni-visa", "Filter in"=w368, "Session in"=w350) -> ("error out"=w365:errorcluster, "Resources out"=w366:refnum<k20>[], "Session out"=w363:refnum<k21>)  [unwired: 4 in, 1 out]
        n188 = for {
          tunnel: w366 -> [w389] mode=indexing
          tunnel: [w383] -> _ mode=indexing if=w382
          tunnel: w346 -> [w387]
          tunnel: [w386] -> w364 mode=indexing
          tunnel: [w385] -> w348 mode=indexing
          shift-right: [w380] -> w340
          shift-left: w365 -> [w388]
          n189 = property class="System Hardware"(reference=w389, error in=w388) -> (reference out=w386:refnum<k20>, error out=w379:errorcluster, "PortBinding"=w383:string, "Resource"=w385:string)
          n190 = Equal?(x=w385, y=w387) -> (x = y?=w384:bool)
          n191 = call <vilib>:"Clear Errors.vi"("error in (no error)"=w379, "specific error code to clear (0: all)"=-2147220623) -> ("error out"=w380:errorcluster, "specific error cleared?"=w377:bool)  [unwired: 4 in]
          n192 = Not(x=w377) -> (.not. x?=w381:bool)
          n193 = And(x=w384, y=w381) -> (x .and. y?=w382:bool)
        }
        n194 = Concatenate Strings(w360, w346) -> (w358:string)
        n195 = property class="Str"(reference=w359, "Value"=w358) -> ()  [unwired: 1 in, 2 out]
        n196 = local write "VISA Resources found"(w348) -> ()
        n197 = call-poly <vilib>:"Close.vi"("error in (no error)"=w340, "Resources in"=w364) -> ("error out"=w362:errorcluster)  [unwired: 9 in]
        n198 = call-poly <vilib>:"Close.vi"("error in (no error)"=w362, "Session in"=w363) -> ("error out"=w356:errorcluster)  [unwired: 9 in]
        n199 = Enqueue Element(queue=w354, element=CTL_Control_States."Save HW Settings", error in (no error)=w356) -> (queue out=w343:refnum<queue>, error out=w345:errorcluster)  [unwired: 1 in, 1 out]
        n200 = Enqueue Element(queue=w343, element=CTL_Control_States."Set I/O config (silent)", error in (no error)=w345) -> (queue out=w342:refnum<queue>, error out=w344:errorcluster)  [unwired: 1 in, 1 out]
        n201 = Enqueue Element(queue=w342, element=CTL_Control_States."Unlock UI (init OK)", error in (no error)=w344) -> (queue out=w353:refnum<queue>, error out=w352:errorcluster)  [unwired: 1 in, 1 out]
        n202 = call <vilib>:"Unset Busy.vi"("error in (no error)"=w352) -> ("error out"=w375:errorcluster)  [unwired: 10 in]
      }
      frame "Save HW Settings" {
        n203 = global read "SW_Globals_2.2+.vi" "Paths"() -> (w402:T68)
        n204 = Unbundle By Name(w402) -> ("Program settings"=w401:path)
        n205 = global read "SW_Globals_2.2+.vi" "Settings cluster"() -> (w390:T16)
        n206 = call <vilib>:"Open Config Data.vi"("error in (no error)"=w399, "create file if necessary (T)"=FALSE, "configuration file path"=w401) -> ("error out"=w397:errorcluster, "refnum"=w398:T69)  [unwired: 6 in, 1 out]
        n207 = local write "Settings cluster (local)"(w390) -> ()
        n208 = call "SW_Save_parameter_group_2.vi"("Researcher name"="Researcher", "error in"=w397, "Settings cluster in"=w390, "Parameter group"=T52 "Defaults", "Settings file refnum in"=w398) -> ("error out"=w396:errorcluster, "Settings file refnum out"=w395:T69)  [unwired: 4 in, 1 out]
        n209 = call <vilib>:"Close Config Data.vi"("error in (no error)"=w396, "refnum"=w395) -> ("error out"=w394:errorcluster)  [unwired: 8 in, 1 out]
      }
      frame "Unlock UI (init OK)" {
        n210 = global read "SW_Globals_2.2+.vi" "Settings cluster"() -> (w404:T16)
        n211 = global read "SW_Globals_2.2+.vi" "All references"() -> (w417:T36)
        n212 = local write "Settings cluster (local)"(w404) -> ()
        n213 = call "UI_(02)_Unlock.vi"("error in (no error)"=w418, "Settings cluster in"=w404, "All references in"=w417) -> ("error out"=w416:errorcluster)  [unwired: 2 out]
        n214 = Enqueue Element(queue=w415, element=CTL_Control_States."Zones layout update", error in (no error)=w416) -> (queue out=w412:refnum<queue>, error out=w413:errorcluster)  [unwired: 1 in, 1 out]
        n215 = Enqueue Element(queue=w412, element=CTL_Control_States."Upd. trace length", error in (no error)=w413) -> (queue out=w407:refnum<queue>, error out=w410:errorcluster)  [unwired: 1 in, 1 out]
        n216 = Enqueue Element(queue=w407, element=CTL_Control_States."Update filter", error in (no error)=w410) -> (queue out=w408:refnum<queue>, error out=w409:errorcluster)  [unwired: 1 in, 1 out]
      }
      frame "Switch to Offline mode" {
        n217 = Get Notifier Status(notifier=w430, error in (no error)=w429) -> (notifier out=w428:refnum<notifier>, current notification=w425:T46, error out=w427:errorcluster)  [unwired: 2 out]
        n218 = Bundle By Name(cluster=w425, "Offline mode"=TRUE) -> (w423:T46)
        n219 = Send Notification(notification=w423, notifier=w428, error in (no error)=w427) -> (notifier out=w426:refnum<notifier>, error out=w422:errorcluster)
        n220 = global read "SW_Globals_2.2+.vi" "Settings cluster"() -> (w419:T16)
        n221 = global read "SW_Globals_2.2+.vi" "All references"() -> (w420:T36)
        n222 = call "UI_(02B)_Switch_to_offline_mode.vi"("error in (no error)"=w422, "Settings cluster in"=w419, "All references in"=w420) -> ("error out"=w421:errorcluster)  [unwired: 5 in, 2 out]
      }
      frame "Switch to Online mode" {
        w432 = FALSE ("Offline mode")
        n223 = Get Notifier Status(notifier=w440, error in (no error)=w439) -> (notifier out=w438:refnum<notifier>, current notification=w434:T46, error out=w437:errorcluster)  [unwired: 2 out]
        n224 = Bundle By Name(cluster=w434, "Has been recorded"=w432, "Offline mode"=w432) -> (w433:T46)
        n225 = Send Notification(notification=w433, notifier=w438, error in (no error)=w437) -> (notifier out=w435:refnum<notifier>, error out=w436:errorcluster)
      }
      frame "Re-check HW (init failed)" {
        w453 = enum32{"Settings", "Recording and Analysis"}."Settings" ("Value")
        n226 = global read "SW_Globals_2.2+.vi" "All references"() -> (w464:T36)
        n227 = Unbundle By Name(w464) -> ("Controls references.Set/Rec and Analyse Tab"=w454:refnum<vi>, "Indicators references.Ready"=w461:refnum<vi>, "Controls references.Check HW connection"=w460:refnum<vi>)
        n228 = property class="TabCtl (strict)"(reference=w454, error in=w450, "Value"=w453) -> (error out=w447:errorcluster, "Pages"=w451:refnum<vi>[])  [unwired: 1 out]
        n229 = To Long Integer(number=w453) -> (32bit integer=w452:i32)
        n230 = Index Array(array=w451, index=w452) -> (element=w449:refnum<vi>)
        n231 = property class="Page"(reference=w449, error in=w447, "PageEnb"=T53."Page Enabled" ("Page Enabled State")) -> (error out=w446:errorcluster)  [unwired: 1 out]
        n232 = property class="Bool (strict)"(reference=w460, error in=w446, "DisabledEnum"=T54."Enabled" ("Disabled")) -> (error out=w458:errorcluster)  [unwired: 1 out]
        n233 = property class="Bool (strict)"(reference=w461, error in=w458, "Value"=FALSE, "Colors [4]"=T51 [{"Numeric Control"=16749459, "Numeric Control"=16749459}, {"Numeric Control"=1988894, "Numeric Control"=3381555}, {"Numeric Control"=4934475, "Numeric Control"=7895160}, {"Numeric Control"=994319, "Numeric Control"=1657881}]) -> (error out=w443:errorcluster)  [unwired: 1 out]
        n234 = flat-sequence {
          tunnel: [w466] -> w444
          tunnel: w443 -> [w465]
          tunnel: [w465] -> w442
          frame #0 {
            n235 = call <vilib>:"Three Button Dialog.vi"("Allow user to close window? (TRUE)"=FALSE, "Window Title (\"\")"="Connection error" ("Window Title (\"\")"), "Right Button Text (\"Cancel\")"="Offline mode" ("Right Button Text (\"Cancel\")"), "Center Button Text (\"No\")"="Adjust Settings" ("Center Button Text (\"No\")"), "Left Button Text (\"Yes\")"="Retry" ("Left Button Text (\"Yes\")"), "message"="Cannot connect to hardware!") -> ("Which Button?"=w466:T70)  [unwired: 5 in]
          }
        }
        n236 = case shown="\"Center Button\"" w444 {
          tunnel: w457 -> [w477 w482 w487]
          tunnel: [w476 w481 w486] -> w456
          tunnel: w442 -> [w475 w480 w485]
          tunnel: [w474 w479 w484] -> w455
          frame "Left Button", Default {
            # "Re-check automatically"
            n237 = Enqueue Element(queue=w477, element=CTL_Control_States."HW Init", error in (no error)=w475) -> (queue out=w476:refnum<queue>, error out=w474:errorcluster)  [unwired: 1 in, 1 out]
          }
          frame "Center Button" {
            # "Pop-up manual port adjustment dialog"
            n238 = Enqueue Element(queue=w482, element=CTL_Control_States."Configure port(s)", error in (no error)=w480) -> (queue out=w481:refnum<queue>, error out=w479:errorcluster)  [unwired: 1 in, 1 out]
          }
          frame "Right Button" {
            # "Switch to offline mode"
            n239 = Enqueue Element(queue=w487, element=CTL_Control_States."Switch to Offline mode", error in (no error)=w485) -> (queue out=w486:refnum<queue>, error out=w484:errorcluster)  [unwired: 1 in, 1 out]
          }
        }
      }
      frame "Configure port(s)" {
        w501 = enum32{"Settings", "Recording and Analysis"}."Settings" ("Value")
        n240 = global read "SW_Globals_2.2+.vi" "All references"() -> (w512:T36)
        n241 = Unbundle By Name(w512) -> ("Controls references.Set/Rec and Analyse Tab"=w502:refnum<vi>, "Indicators references.Ready"=w509:refnum<vi>, "Controls references.Check HW connection"=w508:refnum<vi>)
        n242 = property class="TabCtl (strict)"(reference=w502, error in=w498, "Value"=w501) -> (error out=w495:errorcluster, "Pages"=w499:refnum<vi>[])  [unwired: 1 out]
        n243 = To Long Integer(number=w501) -> (32bit integer=w500:i32)
        n244 = Index Array(array=w499, index=w500) -> (element=w497:refnum<vi>)
        n245 = property class="Page"(reference=w497, error in=w495, "PageEnb"=T53."Page Enabled" ("Page Enabled State")) -> (error out=w494:errorcluster)  [unwired: 1 out]
        n246 = property class="Bool (strict)"(reference=w508, error in=w494, "DisabledEnum"=T54."Enabled" ("Disabled")) -> (error out=w506:errorcluster)  [unwired: 1 out]
        n247 = global read "SW_Globals_2.2+.vi" "Settings cluster"() -> (w490:T16)
        n248 = property class="Bool (strict)"(reference=w509, error in=w506, "Value"=FALSE, "Colors [4]"=T51 [{"Numeric Control"=16749459, "Numeric Control"=16749459}, {"Numeric Control"=1988894, "Numeric Control"=3381555}, {"Numeric Control"=4934475, "Numeric Control"=7895160}, {"Numeric Control"=994319, "Numeric Control"=1657881}]) -> (error out=w492:errorcluster)  [unwired: 1 out]
        n249 = call "HW_Configure_port(s).vi"("Settings cluster in"=w490, "error in (no error)"=w492) -> ("Settings cluster out"=w488:T16, "error out"=w491:errorcluster)  [unwired: 1 out]
        n250 = global write "SW_Globals_2.2+.vi" "Settings cluster"(w488) -> ()
        n251 = local write "Settings cluster (local)"(w488) -> ()
        n252 = Enqueue Element(queue=w505, element=CTL_Control_States."HW Init", error in (no error)=w491) -> (queue out=w504:refnum<queue>, error out=w503:errorcluster)  [unwired: 1 in, 1 out]
      }
      frame "Update filter" {
        (unwired) dbl[] [] ("Reverse coefficients")
        w516 = 11 ("half-width")
        n253 = global read "SW_Globals_2.2+.vi" "Settings cluster"() -> (w533:T16)
        n254 = local read "Calibration parameters"() -> (w529:T23)
        n255 = Unbundle By Name(w533) -> ()  [unwired: 1 out]
        n256 = Unbundle By Name(w529) -> ("True FPS"=w522:dbl)
        n257 = Greater Than 0?(x=w522) -> (x > 0?=w521:bool)
        n258 = local read "FPS status"() -> (w520:i32)
        n259 = Select(t=w522, s=w521, f=w520) -> (s? t:f=w519:dbl)
        n260 = local read "Pre-filter params."() -> (w527:T28)
        n261 = Reciprocal(x=w519) -> (1/x=w518:dbl)
        n262 = call <vilib>:"Smoothing Filter Coefficients.vi"("fs"=w519, "time constant"=0.1, "shape"=enum16{"rectangular", "triangular"}."rectangular", "half-width"=w516, "type"=enum16{"moving average", "exponential"}."exponential") -> ("forward coefficients"=w523:dbl[], "reverse coefficients"=w524:dbl[])  [unwired: 4 in, 1 out]
        n263 = call "SW_SG_coefficients.vi"("Filter parameters"=T17 {"Filter type"=enum."Savitzky-Golay", "Length"=23, "Order"=3}) -> ()  [unwired: 2 in, 1 out]
        n264 = Multiply(x=w516, y=2) -> (x*y=w514:i32)
        n265 = Increment(x=w514) -> (x+1=w513:i32)
        n266 = Bundle(cluster=w527, "Reverse coefficients"=w524, "Forward coefficients"=w523, "Full filter length (info only)"=w513, "Type"=enum16{"None", "FIR (PtbyPt)", "IIR (PtbyPt)"}."IIR (PtbyPt)") -> (w526:T28)
        n267 = local write "Act. frame time, s"(w518) -> ()
        n268 = local write "Pre-filter params."(w526) -> ()
      }
      frame "Zones layout update" {
        n269 = global read "SW_Globals_2.2+.vi" "All references"() -> (w577:T36)
        n270 = local read "Settings cluster (local)"() -> (w579:T16)
        n271 = Unbundle By Name(w577) -> ("Indicators references.Current zone"=w576:refnum<vi>)
        n272 = Get Notifier Status(notifier=w581, error in (no error)=w572) -> (notifier out=w569:refnum<notifier>, current notification=w571:T46, error out=w567:errorcluster)  [unwired: 2 out]
        n273 = Unbundle By Name(w577) -> ("Controls references.Show zones"=w588:refnum<vi>, "Controls references.Show magnets"=w587:refnum<vi>)
        n274 = Unbundle By Name(w579) -> ("Geometry"=w549:T19)
        n275 = Bundle By Name(cluster=w571, "Updating layout"=TRUE) -> (w568:T46)
        n276 = call "SW_Check_segments_parameters_2.vi"("Geometry in"=w549) -> ("Error Out"=w547:errorcluster, "Segmentation out"=w578:T14, "Geometry out"=w536:T19)  [unwired: 2 in]
        n277 = property class="Bool (strict)"(reference=w588) -> ("Value"=w542:bool)  [unwired: 1 in, 2 out]
        n278 = Select(t=T54."Disabled and Grayed Out" ("Disabled"), s=w542, f=T54."Enabled" ("Disabled")) -> (s? t:f=w584:T54)
        n279 = property class="Bool (strict)"(reference=w587, "DisabledEnum"=w584) -> ("Value"=w541:bool)  [unwired: 1 in, 2 out]
        n280 = Send Notification(notification=w568, notifier=w569, error in (no error)=w567) -> (notifier out=w562:refnum<notifier>, error out=w557:errorcluster)
        n281 = local write "Cage radial segmentation"(w578) -> ()
        n282 = call "2 ms delay"("error in (no error)"=w557) -> ("error out"=w546:errorcluster)  [unwired: 10 in]
        n283 = Merge Errors(w547, w546) -> (w548:errorcluster)
        n284 = call "UI_update_Zone_indicator_params_(univ).vi"("error in (no error)"=w548, "Geometry"=w549, "Zone indicator ref. in"=w576) -> ("error out"=w575:errorcluster)  [unwired: 7 in, 1 out]
        n285 = Bundle("Geometry out"=w536, "Value"=w542, "Value"=w541) -> (w539:T71)  [unwired: 1 in]
        n286 = call "New Layout (instant).vi"("error in (no error)"=w546, "Cage parameters"=w539) -> ("Reply Payload"=w545:T62)  [unwired: 7 in, 2 out]
        n287 = Unbundle By Name(w545) -> ("Cage Diagram ref"=w544:T15, "Pixel <> Zone"=w543:T3, "Cage drawing parameters out.Image Scaling info.Pixels per mm"=w537:dbl, "New Layout (instant)_error"=w538:errorcluster)
        n288 = local read "Speed threshold"() -> (w551:dbl)
        n289 = Not(x=w542) -> (.not. x?=w582:bool)
        n290 = local write "Diagram (generated)"(w544) -> ()
        n291 = disable-structure shown="Disabled" {
          disable-tunnel: [w589 _] -> _
          frame Disabled {
            n292 = call "SW_Generate_Segmented_Plot_v4_DAQmx.vi"() -> ("Image geometrical and scaling parameters"=w590:T30)  [unwired: 9 in, 6 out]
            n293 = local write "Img geom and scaling"(w590) -> ()
            n294 = Unbundle By Name(w590) -> ("Pixels per mm"=w589:dbl)
          }
          frame Enabled {
          }
        }
        n295 = local write "Bright mouse lineout"(w582) -> ()
        n296 = Bundle By Name(cluster=T4 {"max"=300.0, "min"=0.0, "# bins"=10, "threshold"=8.0, "thr. type"=enum."higher accepted"} ("Histogram parameters"), "threshold"=w551) -> (w550:T4)
        n297 = Bundle By Name(cluster=w579, "Geometry"=w536, "Defaults.Histogram parameters"=w550) -> (w540:T16)
        n298 = local write "Settings cluster (local)"(w540) -> ()
        n299 = global write "SW_Globals_2.2+.vi" "Settings cluster"(w540) -> ()
        n300 = local write "Pixel to zone"(w543) -> ()
        n301 = local read "Stats parameters (online)"() -> (w556:T1)
        n302 = local read "Mouse drawing parameters"() -> (w583:T2)
        n303 = Merge Errors(w538, w575) -> (w573:errorcluster)
        n304 = Bundle By Name(cluster=w583, "Bright mouse lineout"=w582, "Pixels per mm"=w537) -> (w555:T2)
        n305 = call "GEN_Histo_Bins_And_X_axis.vi"("Error In"=w573, "Histogram parameters"=w550) -> ("Error Out"=w561:errorcluster, "Bins"=w554:dbl[], "X axis values"=w574:dbl[])  [unwired: 6 in, 1 out]
        n306 = Bundle By Name(cluster=w556, "Mouse drawing parameters"=w555, "Array of the pixel to zone correspondences"=w543, "Hist. bins array"=w554, "Histogram parameters"=w550) -> (w553:T1)
        n307 = Get Notifier Status(notifier=w562, error in (no error)=w561) -> (notifier out=w559:refnum<notifier>, current notification=w558:T46, error out=w560:errorcluster)  [unwired: 2 out]
        n308 = local write "Mouse drawing parameters"(w555) -> ()
        n309 = Bundle By Name(cluster=w558, "Updating layout"=FALSE) -> (w563:T46)
        n310 = local write "Hist. X axis"(w574) -> ()
        n311 = local write "Stats parameters (online)"(w553) -> ()
        n312 = Send Notification(notification=w563, notifier=w559, error in (no error)=w560) -> (notifier out=w565:refnum<notifier>, error out=w566:errorcluster)
      }
      frame "Set I/O config" {
        n313 = global read "SW_Globals_2.2+.vi" "Settings cluster"() -> (w600:T16)
        n314 = global read "SW_Globals_2.2+.vi" "All references"() -> (w610:T36)
        n315 = Unbundle By Name(w600) -> ("Defaults.VISA Resource Name"=w606:string, "IO parameters"=w611:T22, "IO parameters.Sync capability"=w602:u8)
        n316 = Unbundle By Name(w610) -> ("Indicators references.IO status indicator"=w609:refnum<vi>)
        n317 = call "HW_set_IO_ports_3-pos_2.vi"("IO parameters cluster"=w611) -> ("IO parameters cluster output"=w592:T22, "IO changed"=w599:bool)
        n318 = call "SW_get_IO_ports_representation_2.vi"("Sync parameters cluster input"=w592) -> ("IO status indicator"=w608:T39)
        n319 = call "SW_get_config_of_Zones_and_IO_2.vi"("Sync parameters cluster input"=w592) -> ("Ports IO config (OUT is FALSE)"=w593:bool[], "IO inversion config."=w605:u16)  [unwired: 2 out]
        n320 = property class="Clust"(reference=w609, error in=w607, "Value"=w608) -> (error out=w604:errorcluster)  [unwired: 1 out]
        n321 = local write "Ports IO config"(w593) -> ()
        n322 = Bundle By Name(cluster=w600, "IO parameters"=w592) -> (w591:T16)
        n323 = call "HW_Set_IO_Dir_on_ECU.vi"("Error In"=w604, "IO ports config"=w593, "VISA resource name"=w606, "IO inversion config."=w605) -> ("error out"=w601:errorcluster, "VISA resource name out"=w603:refnum<visa-resource-name>)
        n324 = local write "IO parameters"(w592) -> ()
        n325 = case shown="1.." w602 {
          tunnel: w603 -> [_ w628]
          tunnel: w601 -> [w619 w627]
          tunnel: w592 -> [_ w626]
          tunnel: [w619 w622] -> w596
          frame 0, Default {
          }
          frame 1.. {
            w623 = u16 4
            n326 = Unbundle By Name(w626) -> ("IO 1 configuration"=w625:u16, "IO 2 configuration"=w624:u16)
            n327 = Equal?(x=w625, y=w623) -> (x = y?=w621:bool)
            n328 = Equal?(x=w624, y=w623) -> (x = y?=w620:bool)
            n329 = call "HW_Set_SYNC_Status.vi"("error in (no error)"=w627, "SYNC 2"=w621, "SYNC 1"=w620, "VISA Resource name IN"=w628) -> ("error out"=w622:errorcluster)  [unwired: 6 in, 1 out]
          }
        }
        n330 = local write "Settings cluster (local)"(w591) -> ()
        n331 = global write "SW_Globals_2.2+.vi" "Settings cluster"(w591) -> ()
        n332 = case shown="True" w599 {
          tunnel: w598 -> [w613 w614]
          tunnel: [w613 w616] -> w597
          tunnel: w596 -> [w612 w618]
          tunnel: [w612 w615] -> w595
          frame False {
            # "IO not changed"
          }
          frame True {
            # "IO changed"
            n333 = Enqueue Element(queue=w614, element=CTL_Control_States."Save all settings", error in (no error)=w618) -> (queue out=w616:refnum<queue>, error out=w615:errorcluster)  [unwired: 1 in, 1 out]
          }
        }
      }
      frame "Set I/O config (silent)" {
        n334 = global read "SW_Globals_2.2+.vi" "Settings cluster"() -> (w635:T16)
        n335 = global read "SW_Globals_2.2+.vi" "All references"() -> (w645:T36)
        n336 = Unbundle By Name(w635) -> ("Defaults.VISA Resource Name"=w641:string, "IO parameters"=w631:T22, "IO parameters.Sync capability"=w637:u8)
        n337 = Unbundle By Name(w645) -> ("Indicators references.IO status indicator"=w644:refnum<vi>)
        n338 = call "SW_get_IO_ports_representation_2.vi"("Sync parameters cluster input"=w631) -> ("IO status indicator"=w643:T39)
        n339 = call "SW_get_config_of_Zones_and_IO_2.vi"("Sync parameters cluster input"=w631) -> ("Ports IO config (OUT is FALSE)"=w633:bool[], "IO inversion config."=w640:u16)  [unwired: 2 out]
        n340 = property class="Clust"(reference=w644, error in=w642, "Value"=w643) -> (error out=w639:errorcluster)  [unwired: 1 out]
        n341 = local write "Ports IO config"(w633) -> ()
        n342 = Bundle By Name(cluster=w635, "IO parameters"=w631) -> (w632:T16)
        n343 = call "HW_Set_IO_Dir_on_ECU.vi"("Error In"=w639, "IO ports config"=w633, "VISA resource name"=w641, "IO inversion config."=w640) -> ("error out"=w636:errorcluster, "VISA resource name out"=w638:refnum<visa-resource-name>)
        n344 = local write "IO parameters"(w631) -> ()
        n345 = case shown="1.." w637 {
          tunnel: w638 -> [_ w655]
          tunnel: w636 -> [w646 w654]
          tunnel: w631 -> [_ w653]
          tunnel: [w646 w649] -> w629
          frame 0, Default {
          }
          frame 1.. {
            w650 = u16 4
            n346 = Unbundle By Name(w653) -> ("IO 1 configuration"=w652:u16, "IO 2 configuration"=w651:u16)
            n347 = Equal?(x=w652, y=w650) -> (x = y?=w648:bool)
            n348 = Equal?(x=w651, y=w650) -> (x = y?=w647:bool)
            n349 = call "HW_Set_SYNC_Status.vi"("error in (no error)"=w654, "SYNC 2"=w648, "SYNC 1"=w647, "VISA Resource name IN"=w655) -> ("error out"=w649:errorcluster)  [unwired: 6 in, 1 out]
          }
        }
        n350 = local write "Settings cluster (local)"(w632) -> ()
        n351 = global write "SW_Globals_2.2+.vi" "Settings cluster"(w632) -> ()
      }
      frame "Cage and recording settings" {
        n352 = global read "SW_Globals_2.2+.vi" "Paths"() -> (w665:T68)
        n353 = call "SW_Set_Cage_and_Recording_Settings.vi"("error in (no error)"=w676) -> ("Update FPS?"=w668:bool, "Save Config?"=w656:bool, "error out"=w667:errorcluster)  [unwired: 1 in]
        n354 = global read "SW_Globals_2.2+.vi" "Settings cluster"() -> (w663:T16)
        n355 = call "SW_Get_Save_Paths_2.vi"("Settings cluster in"=w663, "Paths in"=w665, "error in (no error)"=w667) -> ("Paths out"=w664:T68, "error out"=w666:errorcluster)  [unwired: 2 in, 2 out]
        n356 = global write "SW_Globals_2.2+.vi" "Paths"(w664) -> ()
        n357 = case shown="True" w668 {
          tunnel: w666 -> [w684 w693]
          tunnel: [w684 w692] -> w658
          tunnel: w669 -> [w685 w691]
          tunnel: [w685 w690] -> w660
          frame False {
          }
          frame True {
            n358 = Enqueue Element(queue=w691, element=CTL_Control_States."Play Stop", error in (no error)=w693) -> (queue out=w687:refnum<queue>, error out=w688:errorcluster)  [unwired: 1 in, 1 out]
            n359 = Enqueue Element(queue=w687, element=CTL_Control_States."Upd. FPS", error in (no error)=w688) -> (queue out=w690:refnum<queue>, error out=w692:errorcluster)  [unwired: 1 in, 1 out]
          }
        }
        n360 = case shown="True" w656 {
          tunnel: w660 -> [w678 w681]
          tunnel: [w678 w680] -> w659
          tunnel: w658 -> [w677 w682]
          tunnel: [w677 w679] -> w657
          frame False {
          }
          frame True {
            n361 = Enqueue Element(queue=w681, element=CTL_Control_States."Save all settings", error in (no error)=w682) -> (queue out=w680:refnum<queue>, error out=w679:errorcluster)  [unwired: 1 in, 1 out]
          }
        }
        n362 = flat-sequence {
          tunnel: w657 -> [w696]
          tunnel: [w703] -> w661
          frame #0 {
            n363 = global read "SW_Globals_2.2+.vi" "Settings cluster"() -> (w702:T16)
            n364 = Unbundle By Name(w702) -> ("Geometry"=w701:T19)
            n365 = global read "SW_Globals_2.2+.vi" "All references"() -> (w706:T36)
            n366 = Unbundle By Name(w706) -> ("Indicators references.Cage size"=w705:refnum<vi>)
            n367 = call "SW_Read_Cage's_Geometrical_Parameter.vi"("Error In"=w696, "Parameter to read"=enum16{"None", "Cage diameter/size"}."Cage diameter/size", "Geometry in"=w701) -> ("Error Out"=w697:errorcluster, "Parameter value"=w699:variant)  [unwired: 6 in, 1 out]
            n368 = local write "Settings cluster (local)"(w702) -> ()
            n369 = Variant To Data(error in=w697, type=u16 0, Variant=w699) -> (data=w698:u16, error out=w695:errorcluster)
            n370 = Number To Decimal String(number=w698) -> (decimal integer string=w708:string)  [unwired: 1 in]
            n371 = Concatenate Strings(w708, " mm cage" ("string")) -> (w704:string)
            n372 = property class="Str"(reference=w705, error in=w695, "Value"=w704) -> (error out=w703:errorcluster)  [unwired: 1 out]
          }
        }
        n373 = Enqueue Element(queue=w659, element=CTL_Control_States."Zones layout update", error in (no error)=w661) -> (queue out=w673:refnum<queue>, error out=w675:errorcluster)  [unwired: 1 in, 1 out]
        n374 = Enqueue Element(queue=w673, element=CTL_Control_States."Update filter", error in (no error)=w675) -> (queue out=w674:refnum<queue>, error out=w662:errorcluster)  [unwired: 1 in, 1 out]
      }
      frame "Play Start" {
        n375 = Get Notifier Status(notifier=w717, error in (no error)=w716) -> (notifier out=w714:refnum<notifier>, current notification=w713:T46, error out=w718:errorcluster)  [unwired: 2 out]
        n376 = Unbundle By Name(w713) -> ("Data loaded"=w709:bool, "Offline mode"=w710:bool)
        n377 = case shown="False" w710 {
          tunnel: w718 -> [w730 w739]
          tunnel: [w724 w740] -> w711
          tunnel: w714 -> [w734 w737]
          tunnel: w713 -> [w733 _]
          tunnel: [w722 w736] -> w712
          tunnel: w709 -> [_ w738]
          frame False {
            # "This part is running when working online"
            n378 = global read "SW_Globals_2.2+.vi" "Settings cluster"() -> (w720:T16)
            n379 = Unbundle By Name(w720) -> ("Defaults.VISA Resource Name"=w731:string)
            n380 = call "HW_Acquisition_Start.vi"("Error In"=w730, "VISA resource name in"=w731) -> ("Error Out"=w727:errorcluster)  [unwired: 1 out]
            n381 = call "Set Parameters and data.vi"("Data"=w720, "Parameter"=CTL_Parameter_transfer_name."All parameters") -> ()  [unwired: 9 in, 1 out]
            n382 = global read "SW_Globals_2.2+.vi" "All references"() -> (w723:T36)
            n383 = Unbundle By Name(w723) -> ("Controls references.Play/Pause"=w729:refnum<vi>)
            n384 = property class="Bool (strict)"(reference=w729, error in=w727, "Value"=TRUE) -> (error out=w726:errorcluster)  [unwired: 1 out]
            n385 = Bundle By Name(cluster=w733, "Acq. is ON"=TRUE ("\"Play\" is ON")) -> (w732:T46)
            n386 = Send Notification(notification=w732, notifier=w734, error in (no error)=w726) -> (notifier out=w722:refnum<notifier>, error out=w725:errorcluster)
            n387 = call "UI_(03A)_Set_Play_State.vi"("error in (no error)"=w725, "Settings cluster in"=w720, "All references in"=w723) -> ("error out"=w724:errorcluster)  [unwired: 2 out]
            n388 = Get Date/Time In Seconds() -> (seconds since 1Jan1904=w721:timestamp)
            n389 = local write "Start time (SW)"(w721) -> ()
          }
          frame True {
            # "This part is running when working offline"
            n390 = case shown="True" w738 {
              tunnel: [w742 w751] -> w740
              tunnel: w739 -> [w742 w749]
              tunnel: w737 -> [w741 w747]
              tunnel: [w741 w747] -> w736
              frame False {
              }
              frame True {
                w743 = TRUE ("Value")
                n391 = local read "Settings cluster (local)"() -> (w748:T16)
                n392 = global read "SW_Globals_2.2+.vi" "All references"() -> (w750:T36)
                n393 = Unbundle By Name(w750) -> ("Controls references.Play/Pause"=w752:refnum<vi>, "Controls references.Reset barplot"=w746:refnum<vi>)
                n394 = property class="Bool (strict)"(reference=w752, error in=w749, "Value"=w743) -> (error out=w745:errorcluster)  [unwired: 1 out]
                n395 = property class="Bool (strict)"(reference=w746, error in=w745, "Val(Sgnl)"=w743) -> (error out=w744:errorcluster)  [unwired: 1 out]
                n396 = call "UI_(07A)_Set_Play_State_(offline).vi"("error in (no error)"=w744, "Settings cluster in"=w748, "All references in"=w750) -> ("error out"=w751:errorcluster)  [unwired: 2 out]
              }
            }
          }
        }
      }
      frame "Play Stop" {
        n397 = Get Notifier Status(notifier=w763, error in (no error)=w762) -> (notifier out=w759:refnum<notifier>, current notification=w758:T46, error out=w764:errorcluster)  [unwired: 2 out]
        n398 = Unbundle By Name(w758) -> ("Acq. is ON"=w755:bool, "Offline mode"=w757:bool)
        n399 = Not(x=w757) -> (.not. x?=w753:bool)
        n400 = And(x=w755, y=w753) -> (x .and. y?=w754:bool)
        n401 = case shown="True" w754 {
          tunnel: w764 -> [w769 w780]
          tunnel: [w765 w774] -> w760
          tunnel: w759 -> [w770 w784]
          tunnel: w758 -> [_ w783]
          tunnel: [w770 w772] -> w756
          frame False {
            w766 = T54."Enabled" ("Disabled")
            # "This part is running when working with the recorded data"
            n402 = property on="Timeline" class="Slide (strict)"(error in=w769, "DisabledEnum"=w766) -> (error out=w768:errorcluster)  [unwired: 1 in, 1 out]
            n403 = property on="Open File" class="Bool (strict)"(error in=w768, "DisabledEnum"=w766) -> (error out=w767:errorcluster)  [unwired: 1 in, 1 out]
            n404 = property on="Start over" class="Bool (strict)"(error in=w767, "DisabledEnum"=w766) -> (error out=w765:errorcluster)  [unwired: 1 in, 1 out]
          }
          frame True {
            # "This part is running when working online"
            n405 = Bundle By Name(cluster=w783, "Acq. is ON"=FALSE ("\"Play\" is ON")) -> (w782:T46)
            n406 = global read "SW_Globals_2.2+.vi" "Settings cluster"() -> (w771:T16)
            n407 = Send Notification(notification=w782, notifier=w784, error in (no error)=w780) -> (notifier out=w772:refnum<notifier>, error out=w779:errorcluster)
            n408 = Unbundle By Name(w771) -> ("Defaults.VISA Resource Name"=w781:string)
            n409 = call "HW_Acquisition_Stop.vi"("Error In"=w779, "VISA resource name in"=w781) -> ("Error Out"=w776:errorcluster)  [unwired: 1 out]
            n410 = global read "SW_Globals_2.2+.vi" "All references"() -> (w773:T36)
            n411 = Unbundle By Name(w773) -> ("Controls references.Play/Pause"=w778:refnum<vi>)
            n412 = property class="Bool (strict)"(reference=w778, error in=w776, "Value"=FALSE) -> (error out=w775:errorcluster)  [unwired: 1 out]
            n413 = call "UI_(04A)_Set_Stop_State.vi"("error in (no error)"=w775, "Settings cluster in"=w771, "All references in"=w773) -> ("error out"=w774:errorcluster)  [unwired: 2 out]
          }
        }
      }
      frame "Start Recording" {
        n414 = Get Notifier Status(notifier=w793, error in (no error)=w792) -> (notifier out=w790:refnum<notifier>, current notification=w789:T46, error out=w794:errorcluster)  [unwired: 2 out]
        n415 = Unbundle By Name(w789) -> ("Offline mode"=w788:bool)
        n416 = case shown="False" w788 {
          tunnel: w794 -> [w806 w831]
          tunnel: [w815 w831] -> w786
          tunnel: w790 -> [w825 w830]
          tunnel: w789 -> [w826 _]
          tunnel: [w814 w830] -> w787
          frame False {
            # "This part is running when working online"
            n417 = global read "SW_Globals_2.2+.vi" "Settings cluster"() -> (w809:T16)
            n418 = global read "SW_Globals_2.2+.vi" "All references"() -> (w808:T36)
            n419 = Unbundle By Name(w808) -> ("Controls references.Reset barplot"=w807:refnum<vi>)
            n420 = local read "TTL in time (HW)"() -> (w810:u32)
            n421 = local read "TTL in time (SW)"() -> (w813:timestamp)
            n422 = global read "SW_Globals_2.2+.vi" "Paths"() -> (w823:T68)
            n423 = call "UI_(05A)_Set_Record_Start_State.vi"("error in (no error)"=w806, "Settings cluster in"=w809, "All references in"=w808) -> ("error out"=w824:errorcluster, "Settings cluster out"=w822:T16)  [unwired: 1 out]
            n424 = property class="Bool (strict)"(reference=w807, error in=w806, "Val(Sgnl)"=TRUE ("Value (Signaling)")) -> (error out=w804:errorcluster)  [unwired: 1 out]
            n425 = local write "Start time (HW)"(w810) -> ()
            n426 = local write "Frame #"(u32 0 ("Frame #")) -> ()
            n427 = call "SW_Get_Save_Paths_2.vi"("Settings cluster in"=w822, "Paths in"=w823, "Time stamp in"=w813, "error in (no error)"=w824) -> ("Settings cluster out"=w818:T16, "Paths out"=w819:T68, "Time stamp out"=w820:timestamp, "error out"=w821:errorcluster)  [unwired: 1 in]
            n428 = call "PR_Prepare_TDMS_for_Recording.vi"("Buffer size, samples"=400, "error in (no error)"=w821, "Time Stamp in"=w820, "Paths in"=w819, "Settings cluster in"=w818) -> ("error out"=w816:errorcluster, "Time Stamp out"=w817:timestamp, "Paths out"=w812:T68, "Settings cluster out"=w800:T16)  [unwired: 3 in]
            n429 = Unbundle By Name(w800) -> ("Defaults.VISA Resource Name"=w799:string, "IO parameters"=w797:T22)
            n430 = local write "Start time (SW)"(w817) -> ()
            n431 = global write "SW_Globals_2.2+.vi" "Settings cluster"(w800) -> ()
            n432 = local write "Settings cluster (local)"(w800) -> ()
            n433 = Unbundle By Name(w812) -> ("TDMS file reference"=w811:refnum<k34>)
            n434 = Merge Errors(w816, w804) -> (w802:errorcluster)
            n435 = Bundle By Name(cluster=w826, "Recording now"=TRUE, "Has been recorded"=FALSE) -> (w828:T46)
            n436 = global write "SW_Globals_2.2+.vi" "Paths"(w812) -> ()
            n437 = call "SW_Fire_TTL_on_start_or_stop.vi"("TTL pulse length, ms"=25.0, "error in (no error)"=w802, "Serial Port In"=w799, "Flush receive buffer?"=TRUE, "IO parameters cluster in"=w797) -> ("error out"=w801:errorcluster)  [unwired: 4 in, 2 out]
            n438 = local write "TDMS ref."(w811) -> ()
            n439 = Send Notification(notification=w828, notifier=w825, error in (no error)=w801) -> (notifier out=w814:refnum<notifier>, error out=w815:errorcluster)
          }
          frame True {
            # "This part is running when working with the recorded data"
          }
        }
      }
      frame "Stop Recording" {
        n440 = Get Notifier Status(notifier=w840, error in (no error)=w839) -> (notifier out=w838:refnum<notifier>, current notification=w837:T46, error out=w841:errorcluster)  [unwired: 2 out]
        n441 = Unbundle By Name(w837) -> ("Offline mode"=w836:bool)
        n442 = case shown="False" w836 {
          tunnel: w841 -> [w842 w871]
          tunnel: [w853 w871] -> w832
          tunnel: w838 -> [w868 w870]
          tunnel: w837 -> [w867 _]
          tunnel: [w866 w870] -> w835
          tunnel: w834 -> [w856 w869]
          tunnel: [w854 w869] -> w833
          frame False {
            # "This part is running when working online"
            n443 = Bundle By Name(cluster=w867, "Acq. is ON"=FALSE, "Recording now"=FALSE, "Has been recorded"=FALSE) -> (w864:T46)
            n444 = global read "SW_Globals_2.2+.vi" "Settings cluster"() -> (w850:T16)
            n445 = Unbundle By Name(w850) -> ("Defaults.VISA Resource Name"=w846:string, "IO parameters"=w845:T22)
            n446 = call "SW_Fire_TTL_on_start_or_stop.vi"("TTL pulse length, ms"=50.0, "error in (no error)"=w842, "Serial Port In"=w846, "Flush receive buffer?"=FALSE, "IO parameters cluster in"=w845) -> ("error out"=w843:errorcluster, "Serial Port Out"=w847:refnum<visa-resource-name>)  [unwired: 4 in, 1 out]
            n447 = global read "SW_Globals_2.2+.vi" "All references"() -> (w862:T36)
            n448 = Send Notification(notification=w864, notifier=w868, error in (no error)=w843) -> (notifier out=w866:refnum<notifier>, error out=w844:errorcluster)
            n449 = call "HW_Acquisition_Stop.vi"("Error In"=w844, "VISA resource name in"=w847) -> ("Error Out"=w851:errorcluster)  [unwired: 1 out]
            n450 = local read "TDMS ref."() -> (w858:refnum<k34>)
            n451 = call "UI_(06A)_Set_Record_Stop_State.vi"("error in (no error)"=w851, "Settings cluster in"=w850, "All references in"=w862) -> ("error out"=w861:errorcluster)  [unwired: 2 out]
            n452 = TDMS Flush(4:w861, 7:w858) -> (0:w860:errorcluster, 3:w857:refnum<k34>)
            n453 = TDMS Close(8:w860, 11:w857) -> (0:w859:errorcluster)  [unwired: 1 out]
            n454 = Enqueue Element(queue=w856, element=CTL_Control_States."Recording post-processing", error in (no error)=w859) -> (queue out=w854:refnum<queue>, error out=w853:errorcluster)  [unwired: 1 in, 1 out]
          }
          frame True {
            # "This part is running when working with the recorded data"
          }
        }
      }
      frame "Start over" {
        n455 = Two Button Dialog(message="Do you really want to start over? All unsaved changes will be lost!", 1:"No" ("F button name (\"Cancel\")"), 2:"Yes" ("T button name (\"OK\")")) -> (T button?=w878:bool)
        n456 = case shown="True" w878 {
          tunnel: [w883 w897] -> w881
          tunnel: w880 -> [w883 w893]
          tunnel: w877 -> [w884 w892]
          tunnel: [w884 w886] -> w879
          tunnel: [w882 w885] -> w873
          tunnel: w872 -> [w882 w885]
          frame False {
          }
          frame True {
            n457 = Enqueue Element(queue=w893, element=CTL_Control_States."Switch to Online mode", error in (no error)=w892) -> (queue out=w894:refnum<queue>, error out=w895:errorcluster)  [unwired: 1 in, 1 out]
            n458 = Enqueue Element(queue=w894, element=CTL_Control_States."SW Init", error in (no error)=w895) -> (queue out=w897:refnum<queue>, error out=w891:errorcluster)  [unwired: 1 in, 1 out]
            n459 = invoke on="Overlays cluster" class="Clust (strict)" method="Reinit To Default"(error in=w891) -> (error out=w887:errorcluster)  [unwired: 2 in, 2 out]
            n460 = call <vilib>:"Set Busy.vi"("error in (no error)"=w887) -> ("error out"=w890:errorcluster)  [unwired: 9 in, 1 out]
            n461 = flat-sequence {
              tunnel: w890 -> [w899]
              tunnel: [w899] -> w889
              frame #0 {
                n462 = Request Deallocation(TRUE ("flag")) -> ()
              }
            }
            n463 = call "0,5s delay"("error in (no error)"=w889) -> ("error out"=w888:errorcluster)  [unwired: 10 in]
            n464 = Merge Errors(w888) -> (w886:errorcluster)
          }
        }
      }
      frame "Recording post-processing" {
        n465 = Get Notifier Status(notifier=w909, error in (no error)=w908) -> (notifier out=w907:refnum<notifier>, current notification=w906:T46, error out=w910:errorcluster)  [unwired: 2 out]
        n466 = Unbundle By Name(w906) -> ("Offline mode"=w901:bool)
        n467 = case shown="False" w901 {
          tunnel: w910 -> [w953 w956]
          tunnel: [w913 w956] -> w904
          tunnel: w907 -> [w936 w955]
          tunnel: w906 -> [_ _]
          tunnel: [w936 w955] -> w905
          tunnel: w903 -> [w934 w954]
          tunnel: [w912 w954] -> w902
          frame False {
            # "This part is running when working online"
            n468 = local read "Mouse drawing parameters"() -> (w941:T2)
            n469 = local read "Start time (HW)"() -> (w944:u32)
            n470 = local read "Diagram (display)"() -> (w940:T15)
            n471 = local read "Start time (SW)"() -> (w945:timestamp)
            n472 = call <vilib>:"Set Busy.vi"("error in (no error)"=w953) -> ("error out"=w951:errorcluster)  [unwired: 9 in, 1 out]
            n473 = call <vilib>:"Launch Progress Bar.vi"("error in (no error)"=w951, "Enable Cancellation? (T)"=FALSE, "Main Title (\"Working...\")"="Data post-processing: " ("Main Title (\"Working...\")"), "Total Count"=5) -> ("error out"=w939:errorcluster, "Progress Bar Dialog"=w947:refnum<class "Progress Bar Dialog.lvclass">)  [unwired: 6 in]
            n474 = local read "Pixel to zone"() -> (w920:T3)
            n475 = Bundle By Name(cluster=T56 {"Defragment TDMS? (F)"=FALSE, "Start time (SW)"=timestamp(0 s since 1904-01-01), "Start time (HW)"=0, "Data filtering"={"Filter type"=enum."Savitzky-Golay", "Length"=41, "Order"=3}, "Mouse drawing parameters"={"Trace length, samples"=200, "Rainbow track"=FALSE, "Rainbow track is speed"=FALSE, "Bright mouse lineout"=FALSE, "Colors array"=[255, 1791, 3583, 5119, 6911, 8447, 9983, 11775, 13311, 14847, 16639, 18175, 19711, 21503, 23039, 24831, 26367, 27903, 29695, 31231, 33023, 34559, 36095, 37887, 39423, 40959, 42751, 44287, 45823, 47615, 49151, 50943, 52479, 54015, 55807, 57343, 59135, 60671, 62207, 63999, 65535, 196601, 393202, 524268, 720869, 851935, 1048537, 1245138, 1376204, 1572806, 1703871, 1834937, 2031538, 2162604, 2359206, 2555807, 2686873, 2883475, 3014540, 3211142, 3342208, 3473273, 3669875, 3800940, 3997542, 4128608, 4325209, 4521811, 4652876, 4849478, 4980544, 5111609, 5308211, 5439277, 5635878, 5832480, 5963546, 6094611, 6291213, 6487814, 6618880, 6881024, 7143168, 7405312, 7667456, 7864064, 8126208, 8388352, 8650496, 8912640, 9174784, 9436928, 9633536, 9895680, 10157824, 10419968, 10682112, 10944256, 11206400, 11468544, 11730688, 11927296, 12189440, 12451584, 12713728, 12975872, 13238016, 13500160, 13762304, 13958912, 14221056, 14483200, 14745344, 15007488, 15269632, 15531776, 15793920, 15990528, 16252672, 16514816, 16776960, 16776192, 16775424, 16774400, 16773632, 16772864, 16772096, 16771328, 16770560, 16769536, 16768768, 16768000, 16767232, 16766464, 16765696, 16764672, 16763904, 16763136, 16762368, 16761600, 16760832, 16759808, 16759040, 16758272, 16757504, 16756736, 16755712, 16754944, 16754176, 16753408, 16752640, 16751872, 16750848, 16750080, 16749312, 16748544, 16747776, 16747008, 16745984, 16745216, 16744448, 16743680, 16742912, 16741888, 16741120, 16740352, 16739584, 16738816, 16737792, 16737024, 16736256, 16735488, 16734720, 16733696, 16732928, 16732160, 16731392, 16730624, 16729600, 16728832, 16728064, 16727296, 16726528, 16725504, 16724736, 16723968, 16723200, 16722432, 16721408, 16720640, 16719872, 16719104, 16718336, 16717312, 16716544, 16715776, 16715008, 16714240, 16713216, 16712448], "Pixels per mm"=2.533333333333333}, "Size of the image (480x480)"={"X size"=480.0, "Y size"=480.0}, "Image ref. in"="remote image 00000223CD816B68", "Calibration parameters"={"Timing calibration sw/hw"=1.0, "True FPS"=80.0, "True frame time, s"=0.0125, "Disp. calibration info"=[]}, "Pixel to zone"=[]} ("Processing parameters"), "Defragment TDMS? (F)"=TRUE, "Start time (SW)"=w945, "Start time (HW)"=w944, "Data filtering"=T17 {"Filter type"=enum."Savitzky-Golay", "Length"=41, "Order"=3}, "Mouse drawing parameters"=w941, "Image ref. in"=w940, "Pixel to zone"=w920) -> (w942:T56)
            n476 = global read "SW_Globals_2.2+.vi" "Settings cluster"() -> (w921:T16)
            n477 = local write "Reset buffers?"(TRUE ("Reset buffers?")) -> ()
            n478 = global read "SW_Globals_2.2+.vi" "Paths"() -> (w952:T68)
            n479 = call "PR_Recording_post-processing.vi"("Progress Bar Dialog in"=w947, "error in (no error)"=w939, "Processing parameters"=w942, "Paths"=w952, "Settings cluster"=w921) -> ("error out"=w935:errorcluster, "Loaded array data out"=w928:dbl[][], "Overlays cluster out"=w938:T27)  [unwired: 4 in]
            n480 = local write "Overlays cluster"(w938) -> ()
            n481 = Enqueue Element(queue=w934, element=CTL_Control_States."Prepare loaded data playback", error in (no error)=w935) -> (queue out=w915:refnum<queue>, error out=w914:errorcluster)  [unwired: 1 in, 1 out]
            n482 = Index Array(array=w928, index (row) #1=0 ("index (row)"), index (row) #2=3 ("index (row)"), index (row) #3=4 ("index (row)"), index (row) #4=5 ("index (row)"), index (row) #5=9 ("index (row)"), index (row) #6=10 ("index (row)")) -> (element #1=w926:dbl[], element #2=w925:dbl[], element #3=w924:dbl[], element #4=w923:dbl[], element #5=w922:dbl[], element #6=w917:dbl[])  [unwired: 6 in]
            n483 = To Byte Integer(number=w917) -> (8bit integer=w916:i8[])
            n484 = Enqueue Element(queue=w915, element=CTL_Control_States."Save density map(s)", error in (no error)=w914) -> (queue out=w912:refnum<queue>, error out=w913:errorcluster)  [unwired: 1 in, 1 out]
            n485 = local write "Loaded.timeline"(w926) -> ()
            n486 = local write "Loaded.X"(w924) -> ()
            n487 = local write "Loaded.Y"(w923) -> ()
            n488 = local write "Loaded.alpha"(w925) -> ()
            n489 = local write "Loaded.speed"(w922) -> ()
            n490 = local write "Loaded.zones"(w916) -> ()
          }
          frame True {
            # "This part is running when working with the recorded data"
          }
        }
      }
      frame "Prepare loaded data playback" {
        n491 = Get Notifier Status(notifier=w967, error in (no error)=w966) -> (notifier out=w965:refnum<notifier>, current notification=w964:T46, error out=w968:errorcluster)  [unwired: 2 out]
        n492 = Unbundle By Name(w964) -> ("Offline mode"=w957:bool)
        n493 = case shown="True" w957 {
          tunnel: w968 -> [w1005 w1039]
          tunnel: [w1009 w1043] -> w959
          tunnel: w965 -> [w1008 w1042]
          tunnel: w964 -> [_ _]
          tunnel: [w1006 w1040] -> w963
          tunnel: w962 -> [w1007 w1041]
          tunnel: [w1007 w1041] -> w961
          frame False {
            w993 = 0 ("index")
            w1010 = TRUE ("Has been recorded")
            # "This part is running when working online"
            n494 = local read "Loaded.timeline"() -> (w1001:dbl[])
            n495 = global read "SW_Globals_2.2+.vi" "Settings cluster"() -> (w986:T16)
            n496 = global read "SW_Globals_2.2+.vi" "All references"() -> (w1004:T36)
            n497 = local read "Speed threshold"() -> (w975:dbl)
            n498 = Array Max & Min(array=w1001) -> (max value=w1002:dbl, max index (indices)=w999:i32, min value=w1003:dbl, min index (indices)=w1000:i32)
            n499 = call "UI_(08A)_Prepare_loaded_data_playback.vi"("Timeline max, s"=w1002, "error in (no error)"=w1005, "Timeline min, s"=w1003, "Settings cluster in"=w986, "All references in"=w1004) -> ("error out"=w979:errorcluster)  [unwired: 3 in, 2 out]
            n500 = Bundle(cluster=cluster{"Min":dbl, "Max":dbl} {"Min"=0.0, "Max"=0.0}, "Min"=w1003, "Max"=w1002) -> (w996:cluster{"Min":dbl, "Max":dbl})
            n501 = Bundle(cluster=T57 {"TL. min index"=0, "TL. max index"=0}, "TL. min index"=w1000, "TL. max index"=w999) -> (w995:T57)
            n502 = Bundle By Name(cluster=T4 {"max"=300.0, "min"=0.0, "# bins"=10, "threshold"=8.0, "thr. type"=enum."higher accepted"} ("Histogram parameters"), "threshold"=w975) -> (w982:T4)
            n503 = local write "Timeline absolute min&max indices"(w995) -> ()
            n504 = local write "Timeline absolute min&max"(w996) -> ()
            n505 = local write "Timeline min&max"(w996) -> ()
            n506 = local write "Timeline min&max indices"(w995) -> ()
            n507 = local read "Loaded.X"() -> (w978:dbl[])
            n508 = local read "Loaded.Y"() -> (w977:dbl[])
            n509 = local read "Loaded.alpha"() -> (w994:dbl[])
            n510 = local read "Loaded.speed"() -> (w976:dbl[])
            n511 = call "GET_Travel_(offline).vi"("Loaded.X in"=w978, "Loaded.Y in"=w977, "Loaded.Speed in"=w976, "Speed threshold"=w975, "Error In"=w979) -> ("Run length, m"=w971:dbl, "Loaded.Speed out"=w972:dbl[], "Error Out"=w980:errorcluster)  [unwired: 8 in]
            n512 = local write "Run distance, m"(w971) -> ()
            n513 = call "GET_Statistics_(offline).vi"("Error In"=w980, "Histogram parameters"=w982, "Data vector in"=w972) -> ("Error Out"=w974:errorcluster, "Mean thresholded"=w969:dbl, "Perc. thresholded"=w984:dbl, "Histogram data out"=w983:T32)  [unwired: 3 in]
            n514 = local write "Running, perc. of time"(w984) -> ()
            n515 = local write "Histograms"(w983) -> ()
            n516 = call "250 ms delay"("error in (no error)"=w974) -> ("error out"=w973:errorcluster)  [unwired: 10 in]
            n517 = Get Notifier Status(notifier=w1008, error in (no error)=w973) -> (notifier out=w1013:refnum<notifier>, current notification=w1012:T46, error out=w981:errorcluster)  [unwired: 2 out]
            n518 = Bundle By Name(cluster=w1012, "Data loaded"=w1010, "Has been recorded"=w1010, "Offline mode"=w1010) -> (w1011:T46)
            n519 = local write "Average speed, mm/s"(w969) -> ()
            n520 = Index Array(array=w978, index=w993) -> (element=w991:dbl)
            n521 = Index Array(array=w977, index=w993) -> (element=w990:dbl)
            n522 = Index Array(array=w994, index=w993) -> (element=w989:dbl)
            n523 = Index Array(array=w976, index=w993) -> (element=w988:dbl)
            n524 = Send Notification(notification=w1011, notifier=w1013, error in (no error)=w981) -> (notifier out=w1006:refnum<notifier>, error out=w970:errorcluster)
            n525 = Bundle By Name(cluster=T25 {"R from center"=0.0, "phi (mouse angular position in the cage)"=0.0, "alpha (mouse rot. angle)"=0.0, "X"=0.0, "Y"=0.0, "theta (from center towards mouse)"=0.0, "beta (cage rot. against mouse)"=0.0, "w (mouse angle to wall)"=0.0, "Speed (filtered)"=0.0} ("Animal coordinates and speed"), "X"=w991, "Y"=w990, "alpha (mouse rot. angle)"=w989, "Speed (filtered)"=w988) -> (w987:T25)
            n526 = local write "Current position"(w987) -> ()
            n527 = call <vilib>:"Unset Busy.vi"("error in (no error)"=w970) -> ("error out"=w1009:errorcluster)  [unwired: 10 in]
          }
          frame True {
            w1025 = 0 ("index")
            w1045 = TRUE ("Has been recorded")
            # "This part is running when working with the recorded data"
            n528 = local read "Loaded.timeline"() -> (w1035:dbl[])
            n529 = global read "SW_Globals_2.2+.vi" "Settings cluster"() -> (w1018:T16)
            n530 = global read "SW_Globals_2.2+.vi" "All references"() -> (w1037:T36)
            n531 = Array Max & Min(array=w1035) -> (max value=w1036:dbl, max index (indices)=w1033:i32, min value=w1014:dbl, min index (indices)=w1034:i32)
            n532 = call "UI_(08A)_Prepare_loaded_data_playback.vi"("Timeline max, s"=w1036, "error in (no error)"=w1039, "Timeline min, s"=w1014, "Settings cluster in"=w1018, "All references in"=w1037) -> ("error out"=w1038:errorcluster)  [unwired: 3 in, 2 out]
            n533 = Bundle(cluster=cluster{"Min":dbl, "Max":dbl} {"Min"=0.0, "Max"=0.0}, "Min"=w1014, "Max"=w1036) -> (w1030:cluster{"Min":dbl, "Max":dbl})
            n534 = Bundle(cluster=T57 {"TL. min index"=0, "TL. max index"=0}, "TL. min index"=w1034, "TL. max index"=w1033) -> (w1029:T57)
            n535 = local write "Timeline absolute min&max indices"(w1029) -> ()
            n536 = local write "Timeline absolute min&max"(w1030) -> ()
            n537 = local read "Start time (SW)"() -> (w1016:timestamp)
            n538 = local write "Timeline min&max"(w1030) -> ()
            n539 = local write "Timeline min&max indices"(w1029) -> ()
            n540 = call "250 ms delay"("error in (no error)"=w1038) -> ("error out"=w1044:errorcluster)  [unwired: 10 in]
            n541 = Add(x=w1014, y=w1016) -> (x+y=w1015:timestamp)
            n542 = local write "Since track start"(w1014) -> ()
            n543 = Get Notifier Status(notifier=w1042, error in (no error)=w1044) -> (notifier out=w1049:refnum<notifier>, current notification=w1048:T46, error out=w1046:errorcluster)  [unwired: 2 out]
            n544 = local write "Current Time"(w1015) -> ()
            n545 = local read "Loaded.X"() -> (w1028:dbl[])
            n546 = local read "Loaded.Y"() -> (w1027:dbl[])
            n547 = local read "Loaded.alpha"() -> (w1026:dbl[])
            n548 = local read "Loaded.speed"() -> (w1024:dbl[])
            n549 = Bundle By Name(cluster=w1048, "Data loaded"=w1045, "Offline mode"=w1045) -> (w1047:T46)
            n550 = Index Array(array=w1028, index=w1025) -> (element=w1022:dbl)
            n551 = Index Array(array=w1027, index=w1025) -> (element=w1021:dbl)
            n552 = Index Array(array=w1026, index=w1025) -> (element=w1020:dbl)
            n553 = Index Array(array=w1024, index=w1025) -> (element=w1019:dbl)
            n554 = Bundle By Name(cluster=T25 {"R from center"=0.0, "phi (mouse angular position in the cage)"=0.0, "alpha (mouse rot. angle)"=0.0, "X"=0.0, "Y"=0.0, "theta (from center towards mouse)"=0.0, "beta (cage rot. against mouse)"=0.0, "w (mouse angle to wall)"=0.0, "Speed (filtered)"=0.0} ("Animal coordinates and speed"), "X"=w1022, "Y"=w1021, "alpha (mouse rot. angle)"=w1020, "Speed (filtered)"=w1019) -> (w1017:T25)
            n555 = Send Notification(notification=w1047, notifier=w1049, error in (no error)=w1046) -> (notifier out=w1040:refnum<notifier>, error out=w1050:errorcluster)
            n556 = local write "Current position"(w1017) -> ()
            n557 = call <vilib>:"Unset Busy.vi"("error in (no error)"=w1050) -> ("error out"=w1043:errorcluster)  [unwired: 10 in]
          }
        }
        n558 = property on="Mouse speed" class="WFChart (strict)"(error in=w959, "History Data"=waveform(dbl)[] []) -> (error out=w958:errorcluster)  [unwired: 1 in, 1 out]
      }
      frame "Timeline update" {
        n559 = Get Notifier Status(notifier=w1059, error in (no error)=w1058) -> (notifier out=w1057:refnum<notifier>, current notification=w1056:T46, error out=w1060:errorcluster)  [unwired: 2 out]
        n560 = Unbundle By Name(w1056) -> ("Offline mode"=w1051:bool)
        n561 = case shown="False" w1051 {
          tunnel: w1060 -> [w1069 w1084]
          tunnel: [w1062 w1077] -> w1054
          tunnel: w1057 -> [w1075 w1090]
          tunnel: w1056 -> [_ _]
          tunnel: [w1075 w1090] -> w1055
          tunnel: w1053 -> [w1061 w1076]
          tunnel: [w1061 w1076] -> w1052
          frame True {
            # "This part is running when working offline"
            n562 = local read "Timeline absolute min&max indices"() -> (w1072:T26)
            n563 = local read "Timeline absolute min&max"() -> (w1073:cluster{"Tl. min":dbl, "TL. max":dbl})
            n564 = local read "Timeline min&max indices"() -> (w1070:T26)
            n565 = local read "Timeline min&max"() -> (w1071:cluster{"Tl. min":dbl, "TL. max":dbl})
            n566 = local read "Loaded.timeline"() -> (w1074:dbl[])
            n567 = local read "Timeline"() -> (w1067:T37)
            n568 = call "UI_Update_timeline.vi"("Timeline values in"=w1067, "Loaded.timeline"=w1074, "Timeline absolute min&max in"=w1073, "Timeline absolute min&max indices in"=w1072, "Timeline min&max in"=w1071, "Timeline min&max indices in"=w1070, "Error In"=w1069) -> ("Timeline values out"=w1068:T72, "Cur. pos. slider index"=w1064:i32, "Update timeline index?"=w1063:bool, "Timeline min&max out"=w1066:cluster{"Tl. min":dbl, "TL. max":dbl}, "Error Out"=w1062:errorcluster, "Timeline min&max indices out"=w1065:T26)  [unwired: 3 in]
            n569 = local write "Cur. pos. slider index"(w1064) -> ()
            n570 = local write "Update timeline index?"(w1063) -> ()
            n571 = local write "Timeline"(w1068) -> ()
            n572 = local write "Timeline min&max indices"(w1065) -> ()
            n573 = local write "Timeline min&max"(w1066) -> ()
            n574 = local write "Reset buffers?"(w1063) -> ()
          }
          frame False {
            # "This part is running when working with the recorded data"
            n575 = local read "Timeline absolute min&max indices"() -> (w1087:T26)
            n576 = local read "Timeline absolute min&max"() -> (w1088:cluster{"Tl. min":dbl, "TL. max":dbl})
            n577 = local read "Timeline min&max indices"() -> (w1085:T26)
            n578 = local read "Timeline min&max"() -> (w1086:cluster{"Tl. min":dbl, "TL. max":dbl})
            n579 = local read "Loaded.timeline"() -> (w1089:dbl[])
            n580 = local read "Timeline"() -> (w1082:T37)
            n581 = call "UI_Update_timeline.vi"("Timeline values in"=w1082, "Loaded.timeline"=w1089, "Timeline absolute min&max in"=w1088, "Timeline absolute min&max indices in"=w1087, "Timeline min&max in"=w1086, "Timeline min&max indices in"=w1085, "Error In"=w1084) -> ("Timeline values out"=w1083:T72, "Cur. pos. slider index"=w1079:i32, "Update timeline index?"=w1078:bool, "Timeline min&max out"=w1081:cluster{"Tl. min":dbl, "TL. max":dbl}, "Error Out"=w1077:errorcluster, "Timeline min&max indices out"=w1080:T26)  [unwired: 3 in]
            n582 = local write "Cur. pos. slider index"(w1079) -> ()
            n583 = local write "Update timeline index?"(w1078) -> ()
            n584 = local write "Timeline"(w1083) -> ()
            n585 = local write "Timeline min&max indices"(w1080) -> ()
            n586 = local write "Timeline min&max"(w1081) -> ()
            n587 = local write "Reset buffers?"(w1078) -> ()
          }
        }
      }
      frame "Overlay tracks update" {
        n588 = Get Notifier Status(notifier=w1099, error in (no error)=w1098) -> (notifier out=w1097:refnum<notifier>, current notification=w1096:T46, error out=w1100:errorcluster)  [unwired: 2 out]
        n589 = Unbundle By Name(w1096) -> ("Offline mode"=w1091:bool)
        n590 = case shown="False" w1091 {
          tunnel: w1100 -> [w1137 w1182]
          tunnel: [w1122 w1167] -> w1094
          tunnel: w1097 -> [w1145 w1190]
          tunnel: w1096 -> [_ _]
          tunnel: [w1145 w1190] -> w1095
          tunnel: w1093 -> [w1136 w1181]
          tunnel: [w1136 w1181] -> w1092
          frame True {
            w1133 = cluster{"x":i32, "y":i32} {"x"=480, "y"=480}  # Image size
            # "This part is running when working offline"
            n591 = local read "Mouse drawing parameters"() -> (w1131:T2)
            n592 = local read "Loaded.speed"() -> (w1140:dbl[])
            n593 = call <vilib>:"Set Busy.vi"("error in (no error)"=w1137) -> ("error out"=w1115:errorcluster)  [unwired: 9 in, 1 out]
            n594 = local read "Timeline min&max indices"() -> (w1143:T26)
            n595 = local read "Loaded.X"() -> (w1144:dbl[])
            n596 = local read "Loaded.Y"() -> (w1141:dbl[])
            n597 = local read "Speed threshold"() -> (w1111:dbl)
            n598 = Unbundle By Name(w1131) -> ("Pixels per mm"=w1127:dbl)
            n599 = Unbundle By Name(w1143) -> ("Tl. min index"=w1139:i32, "Tl. max index"=w1142:i32)
            n600 = Bundle By Name(cluster=T4 {"max"=300.0, "min"=0.0, "# bins"=10, "threshold"=8.0, "thr. type"=enum."higher accepted"} ("Histogram parameters"), "threshold"=w1111) -> (w1117:T4)
            n601 = local read "Overlays cluster"() -> (w1101:T27)
            n602 = local read "Stats parameters (online)"() -> (w1107:T1)
            n603 = Subtract(x=w1142, y=w1139) -> (x-y=w1138:i32)
            n604 = Array Subset(array=w1144, index=w1139, length=w1138) -> (w1109:dbl[])
            n605 = Array Subset(array=w1141, index=w1139, length=w1138) -> (w1110:dbl[])
            n606 = Array Subset(array=w1140, index=w1139, length=w1138) -> (w1102:dbl[])
            n607 = Multiply(x=w1109, y=w1127) -> (x*y=w1135:dbl[])
            n608 = Multiply(x=w1110, y=w1127) -> (x*y=w1126:dbl[])
            n609 = call "GET_Travel_(offline).vi"("Loaded.X in"=w1109, "Loaded.Y in"=w1110, "Loaded.Speed in"=w1102, "Speed threshold"=w1111, "Error In"=w1115) -> ("Run length, m"=w1112:dbl, "Loaded.Speed out"=w1113:dbl[], "Error Out"=w1114:errorcluster)  [unwired: 8 in]
            n610 = local write "Run distance, m"(w1112) -> ()
            n611 = call "GET_Statistics_(offline).vi"("Error In"=w1114, "Histogram parameters"=w1117, "Data vector in"=w1113) -> ("Error Out"=w1118:errorcluster, "Mean thresholded"=w1108:dbl, "Perc. thresholded"=w1121:dbl, "Histogram data out"=w1120:T32)  [unwired: 3 in]
            n612 = Unbundle By Name(w1107) -> ("Size of the image (480x480)"=w1106:T73)
            n613 = local write "Histograms"(w1120) -> ()
            n614 = local write "Running, perc. of time"(w1121) -> ()
            n615 = Quotient & Remainder(x=w1133, y=T58 {"Width"=2, "Height"=2}) -> (floor(x/y)=w1132:T58)  [unwired: 1 out]
            n616 = local write "Average speed, mm/s"(w1108) -> ()
            n617 = Unbundle(w1132) -> ("Width"=w1130:u32, "Height"=w1125:u32)
            n618 = Add(x=w1135, y=w1130) -> (x+y=w1129:dbl[])
            n619 = Add(x=w1126, y=w1125) -> (x+y=w1124:dbl[])
            n620 = Round To Nearest(number=w1129) -> (nearest integer value=w1128:dbl[])
            n621 = Round To Nearest(number=w1124) -> (nearest integer value=w1123:dbl[])
            n622 = Build Cluster Array(w1128, w1123) -> (w1103:cluster{dbl, dbl}[])
            n623 = call "DRAW_Track_overlays_(offline).vi"("Image size"=w1106, "Overlays cluster in"=w1101, "Full track array"=w1103, "Speed array"=w1102, "Error In"=w1115) -> ("Overlays cluster out"=w1104:T27, "Error Out"=w1105:errorcluster)  [unwired: 9 in]
            n624 = local write "Active part of track"(w1103) -> ()
            n625 = local write "Overlays cluster"(w1104) -> ()
            n626 = local write "Active speed chunk"(w1102) -> ()
            n627 = Merge Errors(w1105, w1118) -> (w1119:errorcluster)
            n628 = call <vilib>:"Unset Busy.vi"("error in (no error)"=w1119) -> ("error out"=w1122:errorcluster)  [unwired: 10 in]
          }
          frame False {
            w1178 = cluster{"x":i32, "y":i32} {"x"=480, "y"=480}  # Image size
            # "This part is running when working with just recorded data"
            n629 = local read "Mouse drawing parameters"() -> (w1176:T2)
            n630 = local read "Loaded.speed"() -> (w1185:dbl[])
            n631 = call <vilib>:"Set Busy.vi"("error in (no error)"=w1182) -> ("error out"=w1160:errorcluster)  [unwired: 9 in, 1 out]
            n632 = local read "Timeline min&max indices"() -> (w1188:T26)
            n633 = local read "Loaded.X"() -> (w1189:dbl[])
            n634 = local read "Loaded.Y"() -> (w1186:dbl[])
            n635 = local read "Speed threshold"() -> (w1156:dbl)
            n636 = Unbundle By Name(w1176) -> ("Pixels per mm"=w1172:dbl)
            n637 = Bundle By Name(cluster=T4 {"max"=300.0, "min"=0.0, "# bins"=10, "threshold"=8.0, "thr. type"=enum."higher accepted"} ("Histogram parameters"), "threshold"=w1156) -> (w1162:T4)
            n638 = Unbundle By Name(w1188) -> ("Tl. min index"=w1184:i32, "Tl. max index"=w1187:i32)
            n639 = local read "Overlays cluster"() -> (w1146:T27)
            n640 = Subtract(x=w1187, y=w1184) -> (x-y=w1183:i32)
            n641 = Array Subset(array=w1189, index=w1184, length=w1183) -> (w1154:dbl[])
            n642 = Array Subset(array=w1186, index=w1184, length=w1183) -> (w1155:dbl[])
            n643 = Array Subset(array=w1185, index=w1184, length=w1183) -> (w1147:dbl[])
            n644 = Multiply(x=w1154, y=w1172) -> (x*y=w1180:dbl[])
            n645 = Multiply(x=w1155, y=w1172) -> (x*y=w1171:dbl[])
            n646 = call "GET_Travel_(offline).vi"("Loaded.X in"=w1154, "Loaded.Y in"=w1155, "Loaded.Speed in"=w1147, "Speed threshold"=w1156, "Error In"=w1160) -> ("Run length, m"=w1157:dbl, "Loaded.Speed out"=w1158:dbl[], "Error Out"=w1159:errorcluster)  [unwired: 8 in]
            n647 = local read "Stats parameters (online)"() -> (w1152:T1)
            n648 = local write "Run distance, m"(w1157) -> ()
            n649 = call "GET_Statistics_(offline).vi"("Error In"=w1159, "Histogram parameters"=w1162, "Data vector in"=w1158) -> ("Error Out"=w1165:errorcluster, "Mean thresholded"=w1153:dbl, "Perc. thresholded"=w1164:dbl, "Histogram data out"=w1163:T32)  [unwired: 3 in]
            n650 = Unbundle By Name(w1152) -> ("Size of the image (480x480)"=w1151:T73)
            n651 = local write "Histograms"(w1163) -> ()
            n652 = local write "Average speed, mm/s"(w1153) -> ()
            n653 = Quotient & Remainder(x=w1178, y=T58 {"Width"=2, "Height"=2}) -> (floor(x/y)=w1177:T58)  [unwired: 1 out]
            n654 = local write "Running, perc. of time"(w1164) -> ()
            n655 = Unbundle(w1177) -> ("Width"=w1175:u32, "Height"=w1170:u32)
            n656 = Add(x=w1180, y=w1175) -> (x+y=w1174:dbl[])
            n657 = Add(x=w1171, y=w1170) -> (x+y=w1169:dbl[])
            n658 = Round To Nearest(number=w1174) -> (nearest integer value=w1173:dbl[])
            n659 = Round To Nearest(number=w1169) -> (nearest integer value=w1168:dbl[])
            n660 = Build Cluster Array(w1173, w1168) -> (w1148:cluster{dbl, dbl}[])
            n661 = call "DRAW_Track_overlays_(offline).vi"("Image size"=w1151, "Overlays cluster in"=w1146, "Full track array"=w1148, "Speed array"=w1147, "Error In"=w1160) -> ("Overlays cluster out"=w1149:T27, "Error Out"=w1150:errorcluster)  [unwired: 9 in]
            n662 = local write "Active part of track"(w1148) -> ()
            n663 = local write "Overlays cluster"(w1149) -> ()
            n664 = local write "Active speed chunk"(w1147) -> ()
            n665 = Merge Errors(w1150, w1165) -> (w1166:errorcluster)
            n666 = call <vilib>:"Unset Busy.vi"("error in (no error)"=w1166) -> ("error out"=w1167:errorcluster)  [unwired: 10 in]
          }
        }
      }
      frame "Location map update" {
        n667 = Get Notifier Status(notifier=w1199, error in (no error)=w1198) -> (notifier out=w1197:refnum<notifier>, current notification=w1196:T46, error out=w1200:errorcluster)  [unwired: 2 out]
        n668 = Unbundle By Name(w1196) -> ("Offline mode"=w1191:bool)
        n669 = case shown="False" w1191 {
          tunnel: w1200 -> [w1215 w1231]
          tunnel: [w1213 w1229] -> w1194
          tunnel: w1197 -> [w1216 w1232]
          tunnel: w1196 -> [_ _]
          tunnel: [w1216 w1232] -> w1195
          tunnel: w1193 -> [w1214 w1230]
          tunnel: [w1214 w1230] -> w1192
          frame False {
            # "This part is running when working with just recorded data"
            n670 = call <vilib>:"Set Busy.vi"("error in (no error)"=w1215) -> ("error out"=w1205:errorcluster)  [unwired: 9 in, 1 out]
            n671 = local read "Stats parameters (online)"() -> (w1212:T1)
            n672 = Unbundle By Name(w1212) -> ("Size of the image (480x480)"=w1210:T73)
            n673 = local read "Active part of track"() -> (w1207:cluster{"Numeric":dbl, "Numeric":dbl}[])
            n674 = call "GET_Location-based_density_map.vi"("ImageSize"=w1210, "XY data"=w1207, "Log2-transform? (T)"=TRUE, "Normalize to 8 bit? (T)"=TRUE, "error in (no error)"=w1205, "Output as Image? (F)"=TRUE) -> ("8-bit pixmap out"=w1211:u32[][], "Density array out"=w1201:dbl[][], "error out"=w1204:errorcluster)  [unwired: 7 in]
            n675 = local read "Overlays cluster"() -> (w1208:T27)
            n676 = Bundle By Name(cluster=w1208, "Location density map image"=w1211, "Location density map"=w1201) -> (w1209:T27)
            n677 = local write "Overlays cluster"(w1209) -> ()
            n678 = call <vilib>:"Unset Busy.vi"("error in (no error)"=w1204) -> ("error out"=w1213:errorcluster)  [unwired: 10 in]
          }
          frame True {
            # "This part is running when working offline"
            n679 = call <vilib>:"Set Busy.vi"("error in (no error)"=w1231) -> ("error out"=w1218:errorcluster)  [unwired: 9 in, 1 out]
            n680 = local read "Stats parameters (online)"() -> (w1228:T1)
            n681 = local read "Active part of track"() -> (w1223:cluster{"Numeric":dbl, "Numeric":dbl}[])
            n682 = Unbundle By Name(w1228) -> ("Size of the image (480x480)"=w1226:T73)
            n683 = call "GET_Location-based_density_map.vi"("ImageSize"=w1226, "XY data"=w1223, "Log2-transform? (T)"=TRUE, "Normalize to 8 bit? (T)"=TRUE, "error in (no error)"=w1218, "Output as Image? (F)"=TRUE) -> ("8-bit pixmap out"=w1227:u32[][], "Density array out"=w1217:dbl[][], "error out"=w1219:errorcluster)  [unwired: 7 in]
            n684 = local read "Overlays cluster"() -> (w1224:T27)
            n685 = Bundle By Name(cluster=w1224, "Location density map image"=w1227, "Location density map"=w1217) -> (w1225:T27)
            n686 = local write "Overlays cluster"(w1225) -> ()
            n687 = call <vilib>:"Unset Busy.vi"("error in (no error)"=w1219) -> ("error out"=w1229:errorcluster)  [unwired: 10 in]
          }
        }
      }
      frame "Speed map update" {
        n688 = Get Notifier Status(notifier=w1241, error in (no error)=w1240) -> (notifier out=w1239:refnum<notifier>, current notification=w1238:T46, error out=w1242:errorcluster)  [unwired: 2 out]
        n689 = Unbundle By Name(w1238) -> ("Offline mode"=w1233:bool)
        n690 = case shown="False" w1233 {
          tunnel: w1242 -> [w1258 w1275]
          tunnel: [w1256 w1273] -> w1236
          tunnel: w1239 -> [w1259 w1276]
          tunnel: w1238 -> [_ _]
          tunnel: [w1259 w1276] -> w1237
          tunnel: w1235 -> [w1257 w1274]
          tunnel: [w1257 w1274] -> w1234
          frame True {
            # "This part is running when working offline"
            n691 = call <vilib>:"Set Busy.vi"("error in (no error)"=w1258) -> ("error out"=w1248:errorcluster)  [unwired: 9 in, 1 out]
            n692 = local read "Stats parameters (online)"() -> (w1255:T1)
            n693 = Unbundle By Name(w1255) -> ("Size of the image (480x480)"=w1253:T73)
            n694 = local read "Active part of track"() -> (w1250:cluster{"Numeric":dbl, "Numeric":dbl}[])
            n695 = local read "Active speed chunk"() -> (w1244:dbl[])
            n696 = call "GET_Speed-based_density_map.vi"("ImageSize"=w1253, "XY data"=w1250, "Log2-transform? (T)"=TRUE, "Normalize to 8 bit? (T)"=TRUE, "error in (no error)"=w1248, "Output as Image? (F)"=TRUE, "Loaded.speed"=w1244) -> ("8-bit pixmap out"=w1254:u32[][], "Density array out"=w1243:dbl[][], "error out"=w1247:errorcluster)  [unwired: 6 in]
            n697 = local read "Overlays cluster"() -> (w1251:T27)
            n698 = Bundle By Name(cluster=w1251, "Speed density map image"=w1254, "Speed density map"=w1243) -> (w1252:T27)
            n699 = local write "Overlays cluster"(w1252) -> ()
            n700 = call <vilib>:"Unset Busy.vi"("error in (no error)"=w1247) -> ("error out"=w1256:errorcluster)  [unwired: 10 in]
          }
          frame False {
            # "This part is running when working with just recorded data"
            n701 = call <vilib>:"Set Busy.vi"("error in (no error)"=w1275) -> ("error out"=w1265:errorcluster)  [unwired: 9 in, 1 out]
            n702 = local read "Stats parameters (online)"() -> (w1272:T1)
            n703 = local read "Active part of track"() -> (w1267:cluster{"Numeric":dbl, "Numeric":dbl}[])
            n704 = Unbundle By Name(w1272) -> ("Size of the image (480x480)"=w1270:T73)
            n705 = local read "Active speed chunk"() -> (w1261:dbl[])
            n706 = call "GET_Speed-based_density_map.vi"("ImageSize"=w1270, "XY data"=w1267, "Log2-transform? (T)"=TRUE, "Normalize to 8 bit? (T)"=TRUE, "error in (no error)"=w1265, "Output as Image? (F)"=TRUE, "Loaded.speed"=w1261) -> ("8-bit pixmap out"=w1271:u32[][], "Density array out"=w1260:dbl[][], "error out"=w1264:errorcluster)  [unwired: 6 in]
            n707 = local read "Overlays cluster"() -> (w1268:T27)
            n708 = Bundle By Name(cluster=w1268, "Speed density map image"=w1271, "Speed density map"=w1260) -> (w1269:T27)
            n709 = local write "Overlays cluster"(w1269) -> ()
            n710 = call <vilib>:"Unset Busy.vi"("error in (no error)"=w1264) -> ("error out"=w1273:errorcluster)  [unwired: 10 in]
          }
        }
      }
      frame "Load recorded data" {
        n711 = global read "SW_Globals_2.2+.vi" "Paths"() -> (w1293:T68)
        n712 = call <vilib>:"Set Busy.vi"("error in (no error)"=w1292) -> ("error out"=w1280:errorcluster)  [unwired: 9 in, 1 out]
        n713 = Unbundle By Name(w1293) -> ("Folder"=w1282:path)
        n714 = Strip Path(path=w1282) -> (stripped path=w1281:path)  [unwired: 1 out]
        n715 = call "File Dialog"("start path"=w1281, "prompt"="Open previously recorded track", "button label"="Open", "error in"=w1280, "pattern (all files)"="*.tdms", "pattern label"="MHC track") -> ("selected path"=w1283:path, "exists"=w1284:bool, "cancelled"=w1285:bool, "error out"=w1287:errorcluster)  [unwired: 6 in]
        n716 = case shown="No Error" w1287 {
          selector: w1287 -> [w1297 w1337]
          tunnel: w1285 -> [w1302 _]
          tunnel: w1284 -> [w1300 _]
          tunnel: w1283 -> [w1298 _]
          tunnel: [w1296 w1341] -> w1279
          tunnel: w1278 -> [w1295 w1340]
          tunnel: [w1294 w1339] -> w1277
          frame No Error {
            n717 = Not(x=w1302) -> (.not. x?=w1301:bool)
            n718 = And(x=w1300, y=w1301) -> (x .and. y?=w1299:bool)
            n719 = case shown="True" w1299 {
              tunnel: w1298 -> [_ w1317]
              tunnel: w1297 -> [w1306 w1334]
              tunnel: [w1308 w1324] -> w1296
              tunnel: w1295 -> [w1305 w1314]
              tunnel: [w1304 w1310] -> w1294
              frame False {
                n720 = Enqueue Element(queue=w1305, element=CTL_Control_States."Switch to Online mode", error in (no error)=w1306) -> (queue out=w1304:refnum<queue>, error out=w1303:errorcluster)  [unwired: 1 in, 1 out]
                n721 = call <vilib>:"Unset Busy.vi"("error in (no error)"=w1303) -> ("error out"=w1308:errorcluster)  [unwired: 10 in]
              }
              frame True {
                n722 = local write "Loaded.TDMS.path"(w1317) -> ()
                n723 = call "SW_Load_proc_data_from_TDMS.vi"("error in (no error)"=w1334, "TDMS track ref. in"=w1317) -> ("error out"=w1315:errorcluster, "Rec start Time Stamp"=w1309:timestamp, "Loaded data output"=w1323:T74)  [unwired: 7 in]
                n724 = Unbundle By Name(w1323) -> ("HW ts and Frame HW time"=w1322:u32[][], "SW timestamp"=w1321:dbl[], "Coords data"=w1320:dbl[][], "TTL IO and Key"=w1319:string[][], "Track properties"=w1311:string[][], "Zone"=w1318:i8[])
                n725 = local write "Start time (SW)"(w1309) -> ()
                n726 = Enqueue Element(queue=w1314, element=CTL_Control_States."Switch to Offline mode", error in (no error)=w1315) -> (queue out=w1313:refnum<queue>, error out=w1316:errorcluster)  [unwired: 1 in, 1 out]
                n727 = local write "Loaded.zones"(w1318) -> ()
                n728 = local write "Loaded.HW ts and Frame HW time"(w1322) -> ()
                n729 = local write "Loaded.timeline"(w1321) -> ()
                n730 = local write "Loaded.Properties"(w1311) -> ()
                n731 = local write "Loaded.TTL IO and Key"(w1319) -> ()
                n732 = Enqueue Element(queue=w1313, element=CTL_Control_States."Process loaded settings", error in (no error)=w1316) -> (queue out=w1310:refnum<queue>, error out=w1324:errorcluster)  [unwired: 1 in, 1 out]
                n733 = Index Array(array=w1320, index (row) #1=0 ("index (row)"), index (row) #2=1 ("index (row)"), index (row) #3=2 ("index (row)"), index (row) #4=3 ("index (row)")) -> (element #1=w1329:dbl[], element #2=w1328:dbl[], element #3=w1327:dbl[], element #4=w1326:dbl[])  [unwired: 4 in]
                n734 = local write "Loaded.X"(w1329) -> ()
                n735 = local write "Loaded.Y"(w1328) -> ()
                n736 = local write "Loaded.alpha"(w1327) -> ()
                n737 = local write "Loaded.speed"(w1326) -> ()
              }
            }
          }
          frame Error {
            n738 = call <vilib>:"Clear Errors.vi"("error in (no error)"=w1337) -> ("error out"=w1336:errorcluster)  [unwired: 5 in, 1 out]
            n739 = Enqueue Element(queue=w1340, element=CTL_Control_States."Switch to Online mode", error in (no error)=w1336) -> (queue out=w1339:refnum<queue>, error out=w1335:errorcluster)  [unwired: 1 in, 1 out]
            n740 = call <vilib>:"Unset Busy.vi"("error in (no error)"=w1335) -> ("error out"=w1341:errorcluster)  [unwired: 10 in]
          }
        }
      }
      frame "Recalculate track with new settings" {
        n741 = disable-structure shown="Disabled" {
          disable-tunnel: w1344 -> [w1356 _]
          disable-tunnel: [w1354 _] -> w1343
          disable-tunnel: w1342 -> [w1353 _]
          frame Disabled {
            n742 = call <vilib>:"Set Busy.vi"("error in (no error)"=w1356) -> ("error out"=w1352:errorcluster)  [unwired: 9 in, 1 out]
            n743 = call "Start Module.vi"("error in (no error)"=w1352) -> ("error out"=w1351:errorcluster, "Wait for Event Sync?"=w1348:bool, "Tracks Repair Broadcast Events"=w1350:T42)  [unwired: 7 in, 1 out]
            n744 = register-events(reference=w1353, error in=w1351, w1350) -> (error out=w1349:errorcluster)  [unwired: 3 in, 1 out]
            n745 = call "Synchronize Module Events.vi"("error in (no error)"=w1349, "Wait for Event Sync?"=w1348) -> ("error out"=w1347:errorcluster)  [unwired: 9 in]
            n746 = call "Show Panel.vi"("error in (no error)"=w1347) -> ("error out"=w1355:errorcluster)  [unwired: 10 in]
            n747 = call <vilib>:"Unset Busy.vi"("error in (no error)"=w1355) -> ("error out"=w1354:errorcluster)  [unwired: 10 in]
          }
          frame Enabled {
          }
        }
      }
      frame "Load custom settings" {
        n748 = global read "SW_Globals_2.2+.vi" "Paths"() -> (w1374:T68)
        n749 = call <vilib>:"Set Busy.vi"("error in (no error)"=w1373) -> ("error out"=w1361:errorcluster)  [unwired: 9 in, 1 out]
        n750 = Unbundle By Name(w1374) -> ("Folder"=w1363:path)
        n751 = Strip Path(path=w1363) -> (stripped path=w1362:path)  [unwired: 1 out]
        n752 = call "Load Settings"("start path"=w1362, "prompt"="Load previously saved settings", "button label"="Load", "error in"=w1361, "pattern (all files)"="*.trset", "pattern label"="Tracker settings") -> ("selected path"=w1364:path, "exists"=w1365:bool, "cancelled"=w1366:bool, "error out"=w1368:errorcluster)  [unwired: 6 in]
        n753 = case shown="No Error" w1368 {
          selector: w1368 -> [w1378 w1394]
          tunnel: w1366 -> [w1383 _]
          tunnel: w1365 -> [w1381 _]
          tunnel: w1364 -> [w1379 _]
          tunnel: [w1377 w1396] -> w1360
          tunnel: w1359 -> [w1376 w1395]
          tunnel: [w1375 w1395] -> w1358
          frame No Error {
            n754 = Not(x=w1383) -> (.not. x?=w1382:bool)
            n755 = And(x=w1381, y=w1382) -> (x .and. y?=w1380:bool)
            n756 = case shown="True" w1380 {
              tunnel: w1379 -> [_ w1387]
              tunnel: w1378 -> [w1384 w1389]
              tunnel: [w1384 w1388] -> w1377
              tunnel: w1376 -> [w1385 w1390]
              tunnel: [w1385 w1391] -> w1375
              frame False {
              }
              frame True {
                n757 = local write "Settings path to load"(w1387) -> ()
                n758 = local write "Load custom? (F)"(TRUE ("Load custom? (F)")) -> ()
                n759 = Enqueue Element(queue=w1390, element=CTL_Control_States."Start over", error in (no error)=w1389) -> (queue out=w1391:refnum<queue>, error out=w1388:errorcluster)  [unwired: 1 in, 1 out]
              }
            }
          }
          frame Error {
            n760 = call <vilib>:"Simple Error Handler.vi"("error in (no error)"=w1394) -> ("error out"=w1393:errorcluster)  [unwired: 4 in, 4 out]
            n761 = call <vilib>:"Clear Errors.vi"("error in (no error)"=w1393) -> ("error out"=w1396:errorcluster)  [unwired: 5 in, 1 out]
          }
        }
        n762 = call <vilib>:"Unset Busy.vi"("error in (no error)"=w1360) -> ("error out"=w1357:errorcluster)  [unwired: 10 in]
      }
      frame "Process loaded settings" {
        w1434 = 1 ("disabled index (col)")
        n763 = local read "Loaded.Properties"() -> (w1437:string[][])
        n764 = global read "SW_Globals_2.2+.vi" "All references"() -> (w1431:T36)
        n765 = local read "Loaded.TDMS.path"() -> (w1403:path)
        n766 = Index Array(array=w1437, index (row) #1=3 ("index (row)"), index (col) #1=w1434, index (row) #2=4 ("index (row)"), index (col) #2=w1434) -> (element #1=w1433:string)  [unwired: 1 out]
        n767 = Unflatten From XML(xml string=w1433, type=T16 {"Defaults"={"Default User"=0.0, "VISA Resource Name "="Tracker", "Histogram parameters"={"max"=300.0, "min"=0.0, "# bins"=10, "threshold"=8.0, "thr. type"=enum."higher accepted"}}, "Recording and saving"={"Researcher name"="Researcher", "Name prefix"="Track", "Data post-processing"={"Filter type"=enum."Savitzky-Golay", "Length"=31, "Order"=3}, "Stop at"=0.0, "\"Stop at\" enabled"=FALSE, "Default save folder path"=path "", "Acquisition FPS"=enum."Max"}, "Geometry"={"Sensor board size"=enum."", "Bridge swap"=FALSE, "Twisted neck"=FALSE, "Bridge H. offset"=0.0, "Bridge V. offset"=0.0, "Magnets orientation"=180.0, "Cage type"=0, "Cage parameters"={"Round"=variant(i16 0), "Square"=variant(u16 30), "Donut-maze"=variant(u16 75), "T-maze"=variant(u8 2), "Sociability-maze"=variant(u8 4)}}, "IO parameters"={"IO general config."=12, "IO 1 configuration"=1, "IO 2 configuration"=1, "IO 3 configuration"=0, "IO 4 configuration"=0, "Activate ext. RS-232"=0, "IO inversion config."=0, "Sync capability"=1}, "Conditions presets array"=[{"Enabled"=FALSE, "Name"="", "Specifier(s)"=[], "Response"={"Response type"=enum."Air puff", "TTL port"=enum."Port 1", "TTL pulse length, ms"=0.0}, "Has been set"=FALSE}, {"Enabled"=FALSE, "Name"="", "Specifier(s)"=[], "Response"={"Response type"=enum."Air puff", "TTL port"=enum."Port 1", "TTL pulse length, ms"=0.0}, "Has been set"=FALSE}, {"Enabled"=FALSE, "Name"="", "Specifier(s)"=[], "Response"={"Response type"=enum."Air puff", "TTL port"=enum."Port 1", "TTL pulse length, ms"=0.0}, "Has been set"=FALSE}, {"Enabled"=FALSE, "Name"="", "Specifier(s)"=[], "Response"={"Response type"=enum."Air puff", "TTL port"=enum."Port 1", "TTL pulse length, ms"=0.0}, "Has been set"=FALSE}, {"Enabled"=FALSE, "Name"="", "Specifier(s)"=[], "Response"={"Response type"=enum."Air puff", "TTL port"=enum."Port 1", "TTL pulse length, ms"=0.0}, "Has been set"=FALSE}, {"Enabled"=FALSE, "Name"="", "Specifier(s)"=[], "Response"={"Response type"=enum."Air puff", "TTL port"=enum."Port 1", "TTL pulse length, ms"=0.0}, "Has been set"=FALSE}, {"Enabled"=FALSE, "Name"="", "Specifier(s)"=[], "Response"={"Response type"=enum."Air puff", "TTL port"=enum."Port 1", "TTL pulse length, ms"=0.0}, "Has been set"=FALSE}, {"Enabled"=FALSE, "Name"="", "Specifier(s)"=[], "Response"={"Response type"=enum."Air puff", "TTL port"=enum."Port 1", "TTL pulse length, ms"=0.0}, "Has been set"=FALSE}, {"Enabled"=FALSE, "Name"="", "Specifier(s)"=[], "Response"={"Response type"=enum."Air puff", "TTL port"=enum."Port 1", "TTL pulse length, ms"=0.0}, "Has been set"=FALSE}, {"Enabled"=FALSE, "Name"="", "Specifier(s)"=[], "Response"={"Response type"=enum."Air puff", "TTL port"=enum."Port 1", "TTL pulse length, ms"=0.0}, "Has been set"=FALSE}, {"Enabled"=FALSE, "Name"="", "Specifier(s)"=[], "Response"={"Response type"=enum."Air puff", "TTL port"=enum."Port 1", "TTL pulse length, ms"=0.0}, "Has been set"=FALSE}, {"Enabled"=FALSE, "Name"="", "Specifier(s)"=[], "Response"={"Response type"=enum."Air puff", "TTL port"=enum."Port 1", "TTL pulse length, ms"=0.0}, "Has been set"=FALSE}, {"Enabled"=FALSE, "Name"="", "Specifier(s)"=[], "Response"={"Response type"=enum."Air puff", "TTL port"=enum."Port 1", "TTL pulse length, ms"=0.0}, "Has been set"=FALSE}, {"Enabled"=FALSE, "Name"="", "Specifier(s)"=[], "Response"={"Response type"=enum."Air puff", "TTL port"=enum."Port 1", "TTL pulse length, ms"=0.0}, "Has been set"=FALSE}], "Calibration parameters"={"Timing calibration sw/hw"=1.0, "True FPS"=80.0, "True frame time, s"=0.0125, "Disp. calibration info"=[]}, "Settings loaded OK"=FALSE} ("Settings cluster"), error in (no error)=w1439) -> (value=w1397:T16, error out=w1400:errorcluster)
        n768 = Unbundle By Name(w1431) -> ("Indicators references.IO status indicator"=w1430:refnum<vi>)
        n769 = Strip Path(path=w1403) -> (stripped path=w1398:path)  [unwired: 1 out]
        n770 = Unbundle By Name(w1397) -> ("Calibration parameters.True frame time, s"=w1427:dbl, "IO parameters"=w1423:T22)
        n771 = Bundle By Name(cluster=w1397, "Recording and saving.Default save folder path"=w1398) -> (w1404:T16)
        n772 = local write "Act. frame time, s"(w1427) -> ()
        n773 = call "SW_get_IO_ports_representation_2.vi"("Sync parameters cluster input"=w1423) -> ("IO status indicator"=w1429:T39)
        n774 = local write "Settings cluster (local)"(w1397) -> ()
        n775 = property class="Clust"(reference=w1430, error in=w1400, "Value"=w1429) -> (error out=w1428:errorcluster)  [unwired: 1 out]
        n776 = global read "SW_Globals_2.2+.vi" "Paths"() -> (w1405:T68)
        n777 = call "SW_Get_Save_Paths_2.vi"("Settings cluster in"=w1404, "Paths in"=w1405, "error in (no error)"=w1400, "Create new? (F)"=FALSE) -> ("Paths out"=w1401:T68, "error out"=w1399:errorcluster)  [unwired: 1 in, 2 out]
        n778 = Merge Errors(w1399, w1400, w1428) -> (w1438:errorcluster)
        n779 = Enqueue Element(queue=w1426, element=CTL_Control_States."Zones layout update", error in (no error)=w1438) -> (queue out=w1419:refnum<queue>, error out=w1421:errorcluster)  [unwired: 1 in, 1 out]
        n780 = global write "SW_Globals_2.2+.vi" "Paths"(w1401) -> ()
        n781 = Enqueue Element(queue=w1419, element=CTL_Control_States."Prepare loaded data playback", error in (no error)=w1421) -> (queue out=w1418:refnum<queue>, error out=w1420:errorcluster)  [unwired: 1 in, 1 out]
        n782 = Enqueue Element(queue=w1418, element=CTL_Control_States."Timeline update", error in (no error)=w1420) -> (queue out=w1410:refnum<queue>, error out=w1409:errorcluster)  [unwired: 1 in, 1 out]
        n783 = Enqueue Element(queue=w1410, element=CTL_Control_States."Overlay tracks update", error in (no error)=w1409) -> (queue out=w1411:refnum<queue>, error out=w1413:errorcluster)  [unwired: 1 in, 1 out]
        n784 = Enqueue Element(queue=w1411, element=CTL_Control_States."Location map update", error in (no error)=w1413) -> (queue out=w1415:refnum<queue>, error out=w1416:errorcluster)  [unwired: 1 in, 1 out]
        n785 = Enqueue Element(queue=w1415, element=CTL_Control_States."Speed map update", error in (no error)=w1416) -> (queue out=w1407:refnum<queue>, error out=w1408:errorcluster)  [unwired: 1 in, 1 out]
      }
      frame "Save density map(s)" {
        n786 = local read "Overlays cluster"() -> (w1452:T27)
        n787 = global read "SW_Globals_2.2+.vi" "Paths"() -> (w1486:T68)
        n788 = call <vilib>:"Set Busy.vi"("error in (no error)"=w1457) -> ("error out"=w1442:errorcluster)  [unwired: 9 in, 1 out]
        n789 = call "Get Layout Image as Array.vi"("error in (no error)"=w1442) -> ("error out"=w1440:errorcluster, "Reply Payload"=w1444:T75)  [unwired: 8 in, 1 out]
        n790 = Merge Errors(w1442, w1440) -> (w1441:errorcluster)
        n791 = Unbundle By Name(w1452) -> ("Location density map image"=w1450:u32[][], "Speed density map image"=w1447:u32[][])
        n792 = Unbundle By Name(w1444) -> ("Layout image array (U32)"=w1443:u32[][])
        n793 = Unbundle By Name(w1486) -> ("Density map matrix (time)"=w1466:path, "Density map matrix (speed)"=w1456:path, "Density map picture (time)"=w1454:path, "Density map picture (speed)"=w1453:path)
        n794 = Unbundle By Name(w1452) -> ("Location density map"=w1462:dbl[][], "Speed density map"=w1455:dbl[][])
        n795 = call <vilib>:"Check if File or Folder Exists.vi"("error in (no error)"=w1441, "path"=w1466) -> ("error out"=w1474:errorcluster, "file or folder exists?"=w1485:bool, "dup path"=w1484:path)  [unwired: 7 in]
        n796 = call <vilib>:"Check if File or Folder Exists.vi"("error in (no error)"=w1441, "path"=w1456) -> ("error out"=w1473:errorcluster, "file or folder exists?"=w1478:bool, "dup path"=w1475:path)  [unwired: 7 in]
        n797 = call <vilib>:"Check if File or Folder Exists.vi"("error in (no error)"=w1441, "path"=w1454) -> ("error out"=w1465:errorcluster, "file or folder exists?"=w1469:bool, "dup path"=w1463:path)  [unwired: 7 in]
        n798 = call <vilib>:"Check if File or Folder Exists.vi"("error in (no error)"=w1441, "path"=w1453) -> ("error out"=w1448:errorcluster, "file or folder exists?"=w1458:bool, "dup path"=w1446:path)  [unwired: 7 in]
        n799 = Not(x=w1485) -> (.not. x?=w1483:bool)
        n800 = Not(x=w1478) -> (.not. x?=w1479:bool)
        n801 = Not(x=w1469) -> (.not. x?=w1468:bool)
        n802 = Not(x=w1458) -> (.not. x?=w1459:bool)
        n803 = call-poly <userlib>:"Valid Path__ogtk.vi"("path"=w1466) -> ("valid"=w1481:bool)
        n804 = call-poly <userlib>:"Valid Path__ogtk.vi"("path"=w1456) -> ("valid"=w1480:bool)
        n805 = call-poly <userlib>:"Valid Path__ogtk.vi"("path"=w1454) -> ("valid"=w1467:bool)
        n806 = call-poly <userlib>:"Valid Path__ogtk.vi"("path"=w1453) -> ("valid"=w1460:bool)
        n807 = And(x=w1483, y=w1481) -> (x .and. y?=w1482:bool)
        n808 = And(x=w1479, y=w1480) -> (x .and. y?=w1476:bool)
        n809 = And(x=w1468, y=w1467) -> (x .and. y?=w1464:bool)
        n810 = And(x=w1459, y=w1460) -> (x .and. y?=w1449:bool)
        n811 = case shown="True" w1482 {
          tunnel: w1484 -> [_ w1517]
          tunnel: w1462 -> [_ w1516]
          tunnel: w1474 -> [w1513 w1515]
          tunnel: [w1513 w1514] -> w1472
          frame False {
          }
          frame True {
            n812 = call-poly <vilib>:"Write Delimited Spreadsheet.vi"("file path (dialog if empty)"=w1517, "2D data"=w1516, "error in (no error)"=w1515) -> ("error out"=w1514:errorcluster)  [unwired: 11 in, 1 out]
          }
        }
        n813 = case shown="True" w1476 {
          tunnel: w1475 -> [_ w1512]
          tunnel: w1455 -> [_ w1511]
          tunnel: w1473 -> [w1508 w1510]
          tunnel: [w1508 w1509] -> w1471
          frame False {
          }
          frame True {
            n814 = call-poly <vilib>:"Write Delimited Spreadsheet.vi"("file path (dialog if empty)"=w1512, "2D data"=w1511, "error in (no error)"=w1510) -> ("error out"=w1509:errorcluster)  [unwired: 11 in, 1 out]
          }
        }
        n815 = case shown="True" w1464 {
          tunnel: w1465 -> [w1498 w1505]
          tunnel: [w1498 w1506] -> w1461
          tunnel: w1463 -> [_ w1507]
          tunnel: w1450 -> [_ w1503]
          tunnel: w1443 -> [_ w1504]
          frame False {
          }
          frame True {
            n816 = call "SW_Create_Images_overlay.vi"("Blend factor"=0.15, "Background color"=u32 16777216, "Overlay Image"=w1503, "Background image"=w1504) -> ("Output Image"=w1502:u32[][])  [unwired: 1 in, 1 out]
            n817 = call <vilib>:"Flatten Pixmap.vi"("24-bit pixmap"=w1502) -> ("image data"=w1501:T76)  [unwired: 10 in]
            n818 = call <vilib>:"Write PNG File.vi"("error in (no error)"=w1505, "image data"=w1501, "path to PNG file"=w1507) -> ("error out"=w1506:errorcluster)  [unwired: 7 in, 1 out]
          }
        }
        n819 = case shown="True" w1449 {
          tunnel: w1448 -> [w1488 w1495]
          tunnel: [w1488 w1496] -> w1445
          tunnel: w1446 -> [_ w1497]
          tunnel: w1447 -> [_ w1493]
          tunnel: w1443 -> [_ w1494]
          frame False {
          }
          frame True {
            n820 = call "SW_Create_Images_overlay.vi"("Blend factor"=0.07, "Background color"=u32 16777216, "Overlay Image"=w1493, "Background image"=w1494) -> ("Output Image"=w1492:u32[][])  [unwired: 1 in, 1 out]
            n821 = call <vilib>:"Flatten Pixmap.vi"("24-bit pixmap"=w1492) -> ("image data"=w1491:T76)  [unwired: 10 in]
            n822 = call <vilib>:"Write PNG File.vi"("error in (no error)"=w1495, "image data"=w1491, "path to PNG file"=w1497) -> ("error out"=w1496:errorcluster)  [unwired: 7 in, 1 out]
          }
        }
        n823 = Merge Errors(w1472, w1471, w1461, w1445) -> (w1470:errorcluster)
        n824 = call <vilib>:"Unset Busy.vi"("error in (no error)"=w1470) -> ("error out"=w1451:errorcluster)  [unwired: 10 in]
      }
      frame "Upd. FPS" {
        n825 = Get Notifier Status(notifier=w1530, error in (no error)=w1529) -> (notifier out=w1520:refnum<notifier>, current notification=w1528:T46, error out=w1522:errorcluster)  [unwired: 2 out]
        n826 = Unbundle By Name(w1528) -> ("Acq. is ON"=w1524:bool, "Offline mode"=w1527:bool)
        n827 = Not(x=w1527) -> (.not. x?=w1526:bool)
        n828 = Not(x=w1524) -> (.not. x?=w1523:bool)
        n829 = And(x=w1523, y=w1526) -> (x .and. y?=w1525:bool)
        n830 = case shown="True" w1525 {
          tunnel: w1522 -> [w1532 w1547]
          tunnel: [w1532 w1537] -> w1521
          tunnel: w1519 -> [w1531 w1543]
          tunnel: [w1531 w1536] -> w1518
          frame False {
          }
          frame True {
            # "Change FPS while device is online, but acqusition is stopped."
            n831 = global read "SW_Globals_2.2+.vi" "Settings cluster"() -> (w1533:T16)
            n832 = Unbundle By Name(w1533) -> ("Defaults.VISA Resource Name"=w1552:string, "Recording and saving.Acquisition FPS"=w1551:T18)
            n833 = local read "Sensor board size"() -> (w1550:string)
            n834 = local read "FPS status"() -> (w1549:i32)
            n835 = call "LL_Set_FPS_on_device.vi"("VISA in"=w1552, "Desired FPS"=w1551, "Sensor board size"=w1550, "Current FPS"=w1549, "Error in (no error)"=w1547) -> ("FPS set on device"=w1548:i32, "Error out"=w1546:errorcluster)  [unwired: 9 in, 4 out]
            n836 = local write "FPS status"(w1548) -> ()
            n837 = call "Calibration will be executed"("error in (no error)"=w1546, "Enable"=TRUE) -> ("error out"=w1544:errorcluster)  [unwired: 8 in, 1 out]
            n838 = Enqueue Element(queue=w1543, element=CTL_Control_States."Play Stop", error in (no error)=w1544) -> (queue out=w1540:refnum<queue>, error out=w1539:errorcluster)  [unwired: 1 in, 1 out]
            n839 = Enqueue Element(queue=w1540, element=CTL_Control_States."Play Start", error in (no error)=w1539) -> (queue out=w1535:refnum<queue>, error out=w1538:errorcluster)  [unwired: 1 in, 1 out]
            n840 = Enqueue Element(queue=w1535, element=CTL_Control_States."Timings calibration start", error in (no error)=w1538) -> (queue out=w1536:refnum<queue>, error out=w1537:errorcluster)  [unwired: 1 in, 1 out]
          }
        }
      }
      frame "Upd. trace length" {
        (unwired) u32[] [14308646, 16156991, 16694328, 14206596, 6913947] ("Initial colors ramp array")
        w1555 = T77 [255, 65535, 6618880, 16776960, 16744448, 16711680] ("Initial colors ramp array")
        n841 = global read "SW_Globals_2.2+.vi" "All references"() -> (w1582:T36)
        n842 = local read "UI update period"() -> (w1580:i64)
        n843 = Unbundle By Name(w1582) -> ("Controls references.Trace, s"=w1581:refnum<vi>, "Controls references.Rainbow (time)"=w1573:refnum<vi>, "Controls references.Rainbow (speed)"=w1567:refnum<vi>)
        n844 = To Double Precision Float(number=i64 1000 ("x")) -> (double precision float=w1569:dbl)
        n845 = To Double Precision Float(number=w1580) -> (double precision float=w1568:dbl)
        n846 = Divide(x=w1569, y=w1568) -> (x/y=w1577:dbl)
        n847 = property class="Slide (strict)"(reference=w1581, error in=w1575) -> (error out=w1566:errorcluster, "Value"=w1578:u16)  [unwired: 1 out]
        n848 = Multiply(x=w1578, y=w1577) -> (x*y=w1576:dbl)
        n849 = To Unsigned Word Integer(number=w1576) -> (unsigned 16bit integer=w1560:u16)
        n850 = property class="Bool (strict)"(reference=w1567, error in=w1566) -> (error out=w1565:errorcluster, "Value"=w1558:bool)  [unwired: 1 out]
        n851 = Select(t=w1555, s=w1558, f=w1555) -> (s? t:f=w1562:T77)
        n852 = Select(t=u16 300, s=w1558, f=w1560) -> (s? t:f=w1564:u16)
        n853 = call "GEN_Colors_positions.vi"("Highest color position"=w1564, "Initial colors ramp array in"=w1562) -> ("Colors positions"=w1553:dbl[])  [unwired: 1 out]
        n854 = property class="Bool (strict)"(reference=w1573, error in=w1566) -> (error out=w1571:errorcluster, "Value"=w1570:bool)  [unwired: 1 out]
        n855 = call "SW_Generate_Color_Ramp.vi"("Colors rel. pos."=w1553, "Colors array"=w1562) -> ("Colors array"=w1557:u32[])
        n856 = local write "Trace length, samples"(w1560) -> ()
        n857 = local write "Colors array"(w1557) -> ()
        n858 = Or(x=w1570, y=w1558) -> (x .or. y?=w1559:bool)
        n859 = local write "Rainbow track"(w1559) -> ()
        n860 = local write "Rainbow is speed"(w1558) -> ()
        n861 = Merge Errors(w1566, w1571, w1565) -> (w1572:errorcluster)
        n862 = local read "Mouse drawing parameters"() -> (w1561:T2)
        n863 = Bundle By Name(cluster=w1561, "Trace length, samples"=w1560, "Rainbow track"=w1559, "Rainbow track is speed"=w1558, "Colors array"=w1557) -> (w1556:T2)
        n864 = local write "Mouse drawing parameters"(w1556) -> ()
      }
      frame "Timings calibration start" {
        n865 = Get Notifier Status(notifier=w1590, error in (no error)=w1589) -> (notifier out=w1588:refnum<notifier>, current notification=w1584:T46, error out=w1591:errorcluster)  [unwired: 2 out]
        n866 = Unbundle By Name(w1584) -> ("Offline mode"=w1587:bool)
        n867 = case shown="False" w1587 {
          tunnel: w1591 -> [w1605 w1607]
          tunnel: [w1594 w1607] -> w1586
          tunnel: w1588 -> [w1604 w1606]
          tunnel: [w1593 w1606] -> w1585
          tunnel: w1584 -> [w1603 _]
          frame False {
            # "This part is running when working online"
            n868 = call <vilib>:"Set Busy.vi"("error in (no error)"=w1605) -> ("error out"=w1600:errorcluster)  [unwired: 9 in, 1 out]
            n869 = local read "Calibration samples"() -> (w1592:i32)
            n870 = Bundle By Name(cluster=w1603, "Calibration mode"=TRUE) -> (w1601:T46)
            n871 = call <vilib>:"Launch Progress Bar.vi"("error in (no error)"=w1600, "Enable Cancellation? (T)"=FALSE, "Main Title (\"Working...\")"="Collecting samples..." ("Main Title (\"Working...\")"), "Total Count"=w1592) -> ("error out"=w1599:errorcluster, "Progress Bar Dialog"=w1595:refnum<class "Progress Bar Dialog.lvclass">)  [unwired: 6 in]
            n872 = local write "Progress Bar Dialog"(w1595) -> ()
            n873 = call "550 ms delay"("error in (no error)"=w1599) -> ("error out"=w1596:errorcluster)  [unwired: 10 in]
            n874 = Send Notification(notification=w1601, notifier=w1604, error in (no error)=w1596) -> (notifier out=w1593:refnum<notifier>, error out=w1594:errorcluster)
          }
          frame True {
            # "This part is running when working with the recorded data"
          }
        }
      }
      frame "Timings calibration finish" {
        n875 = Get Notifier Status(notifier=w1616, error in (no error)=w1615) -> (notifier out=w1614:refnum<notifier>, current notification=w1610:T46, error out=w1617:errorcluster)  [unwired: 2 out]
        n876 = Unbundle By Name(w1610) -> ("Stop and Exit"=w1613:bool)
        n877 = case shown="False" w1613 {
          tunnel: w1617 -> [w1642 w1645]
          tunnel: [w1641 w1645] -> w1612
          tunnel: w1614 -> [w1624 w1644]
          tunnel: [w1621 w1644] -> w1611
          tunnel: w1610 -> [w1620 _]
          tunnel: w1609 -> [w1631 w1643]
          tunnel: [w1630 w1643] -> w1608
          frame False {
            # "This part is running when working online"
            n878 = local read "Progress Bar Dialog"() -> (w1636:refnum<class "Progress Bar Dialog.lvclass">)
            n879 = local read "Calibration HW timings"() -> (w1639:u32[])
            n880 = local read "Calibration SW timings"() -> (w1638:dbl[])
            n881 = global read "SW_Globals_2.2+.vi" "Settings cluster"() -> (w1626:T16)
            n882 = global read "SW_Globals_2.2+.vi" "Paths"() -> (w1637:T68)
            n883 = Unbundle By Name(w1637) -> ("Program settings"=w1635:path)
            n884 = call <vilib>:"Close Progress Bar.vi"("error in (no error)"=w1642, "Progress Bar Dialog"=w1636) -> ("error out"=w1640:errorcluster)  [unwired: 9 in]
            n885 = call "HW_Timings_Calibration.vi"("Error In"=w1640, "Calibration SW timings"=w1638, "Calibration HW timings"=w1639, "Settings cluster in"=w1626) -> ("Error out"=w1633:T41, "Settings cluster out"=w1627:T16)  [unwired: 1 out]
            n886 = call "SW_Save_Settings_2.vi"("error in (no error)"=w1633, "Parameter group to save"=T52 "Calibration", "Settings cluster"=w1627, "Settings path in"=w1635) -> ("error out"=w1634:errorcluster)  [unwired: 5 in, 1 out]
            n887 = Unbundle By Name(w1627) -> ("Calibration parameters"=w1632:T23, "Calibration parameters.True frame time, s"=w1625:dbl)
            n888 = Bundle By Name(cluster=w1620, "Calibration mode"=FALSE) -> (w1619:T46)
            n889 = global write "SW_Globals_2.2+.vi" "Settings cluster"(w1627) -> ()
            n890 = local write "Settings cluster (local)"(w1627) -> ()
            n891 = local write "Calibration parameters"(w1632) -> ()
            n892 = Enqueue Element(queue=w1631, element=CTL_Control_States."Update filter", error in (no error)=w1634) -> (queue out=w1630:refnum<queue>, error out=w1623:errorcluster)  [unwired: 1 in, 1 out]
            n893 = local write "Act. frame time, s"(w1625) -> ()
            n894 = Send Notification(notification=w1619, notifier=w1624, error in (no error)=w1623) -> (notifier out=w1621:refnum<notifier>, error out=w1622:errorcluster)
            n895 = call <vilib>:"Unset Busy.vi"("error in (no error)"=w1622) -> ("error out"=w1641:errorcluster)  [unwired: 10 in]
          }
          frame True {
            # "This part is running when working with the recorded data"
          }
        }
      }
      frame "Dispension calibration" {
        n896 = global read "SW_Globals_2.2+.vi" "Settings cluster"() -> (w1646:T16)
        n897 = call "SW_Dispension_Calibration.vi"("error in (no error)"=w1654, "Settings cluster in"=w1646) -> ("error out"=w1648:errorcluster, "Settings cluster out"=w1647:T16)  [unwired: 8 in]
        n898 = global write "SW_Globals_2.2+.vi" "Settings cluster"(w1647) -> ()
        n899 = local write "Settings cluster (local)"(w1647) -> ()
        n900 = global read "SW_Globals_2.2+.vi" "Paths"() -> (w1653:T68)
        n901 = Unbundle By Name(w1653) -> ("Program settings"=w1651:path)
        n902 = Unbundle By Name(w1647) -> ("Calibration parameters"=w1652:T23)
        n903 = local write "Calibration parameters"(w1652) -> ()
        n904 = call "SW_Save_Settings_2.vi"("error in (no error)"=w1648, "Parameter group to save"=T52 "Calibration", "Settings cluster"=w1647, "Settings path in"=w1651) -> ("error out"=w1649:errorcluster)  [unwired: 5 in, 1 out]
      }
      frame "Add Reward condition" {
        n905 = local read "Settings cluster (local)"() -> (w1660:T16)
        n906 = local read "Array of conditions"() -> (w1673:T6)
        n907 = control-ref of="Reward and stimulation"() -> (w1670:refnum<vi>)
        n908 = local read "Calibration parameters"() -> (w1671:T23)
        n909 = Unbundle By Name(w1660) -> ("IO parameters"=w1659:T22)
        n910 = call "SW_Add_or_Modify_Reward_Condition.vi"("IO parameters cluster"=w1659, "Add or Modify?"=enum16{"Add", "Modify"}."Add", "error in (no error)"=w1674, "Main Tree Control in"=w1670, "Calibration parameters"=w1671, "Array of conditions in"=w1673) -> ("error out"=w1672:T41, "Main Tree Control out"=w1669:refnum<vi>, "Array of conditions out"=w1662:T6)  [unwired: 3 in]
        n911 = call "DATA_Reorder_after_condition_modification.vi"("Array of conditions"=w1662) -> ("Reordered conditions array"=w1661:T7[])  [unwired: 2 in]
        n912 = Bundle By Name(cluster=w1660, "Conditions presets array"=w1661) -> (w1657:T16)
        n913 = local write "Array of conditions"(w1661) -> ()
        n914 = call "SW_Generate_Full_Condition(s)_text.vi"("error in (no error)"=w1672, "Array of conditions in"=w1661, "Calibration parameters"=w1671, "TreeControl ref in"=w1669) -> ("error out"=w1667:errorcluster)  [unwired: 6 in, 1 out]
        n915 = Enqueue Element(queue=w1666, element=CTL_Control_States."Check Reward condition(s)", error in (no error)=w1667) -> (queue out=w1665:refnum<queue>, error out=w1664:errorcluster)  [unwired: 1 in, 1 out]
        n916 = call "Set Parameters and data.vi"("Data"=w1657, "Parameter"=CTL_Parameter_transfer_name."All parameters") -> ()  [unwired: 9 in, 1 out]
        n917 = local write "Settings cluster (local)"(w1657) -> ()
        n918 = global write "SW_Globals_2.2+.vi" "Settings cluster"(w1657) -> ()
      }
      frame "Modify Reward condition" {
        n919 = local read "Array of conditions"() -> (w1698:T6)
        n920 = control-ref of="Reward and stimulation"() -> (w1696:refnum<vi>)
        n921 = local read "Calibration parameters"() -> (w1688:T23)
        n922 = local read "Settings cluster (local)"() -> (w1687:T16)
        n923 = Unbundle By Name(w1687) -> ("IO parameters"=w1686:T22)
        n924 = call "SW_Add_or_Modify_Reward_Condition.vi"("IO parameters cluster"=w1686, "Add or Modify?"=enum16{"Add", "Modify"}."Modify", "error in (no error)"=w1699, "Main Tree Control in"=w1696, "Calibration parameters"=w1688, "Array of conditions in"=w1698) -> ("error out"=w1697:T41, "Main Tree Control out"=w1695:refnum<vi>, "Array of conditions out"=w1690:T6)  [unwired: 3 in]
        n925 = call "DATA_Reorder_after_condition_modification.vi"("Array of conditions"=w1690) -> ("Reordered conditions array"=w1689:T7[])  [unwired: 2 in]
        n926 = Bundle By Name(cluster=w1687, "Conditions presets array"=w1689) -> (w1677:T16)
        n927 = call "SW_Generate_Full_Condition(s)_text.vi"("error in (no error)"=w1697, "Array of conditions in"=w1689, "Calibration parameters"=w1688, "TreeControl ref in"=w1695) -> ("error out"=w1684:errorcluster, "TreeControl ref out"=w1685:refnum<vi>)  [unwired: 6 in]
        n928 = local write "Array of conditions"(w1689) -> ()
        n929 = property class="Tree (strict)"(reference=w1685, error in=w1684) -> (reference out=w1680:refnum<vi>, error out=w1681:errorcluster, "TopLeft"=w1679:T78)
        n930 = Unbundle By Name(w1679) -> ("Node"=w1678:string)
        n931 = local write "Settings cluster (local)"(w1677) -> ()
        n932 = global write "SW_Globals_2.2+.vi" "Settings cluster"(w1677) -> ()
        n933 = call "Set Parameters and data.vi"("Data"=w1677, "Parameter"=CTL_Parameter_transfer_name."All parameters") -> ()  [unwired: 9 in, 1 out]
        n934 = property class="Tree (strict)"(reference=w1680, error in=w1681, "Value"=w1678) -> (error out=w1682:errorcluster)  [unwired: 1 out]
        n935 = Enqueue Element(queue=w1692, element=CTL_Control_States."Check Reward condition(s)", error in (no error)=w1682) -> (queue out=w1691:refnum<queue>, error out=w1683:errorcluster)  [unwired: 1 in, 1 out]
      }
      frame "Delete Reward condition" {
        n936 = local read "Array of conditions"() -> (w1715:T6)
        n937 = control-ref of="Reward and stimulation"() -> (w1721:refnum<vi>)
        n938 = local read "Calibration parameters"() -> (w1723:T23)
        n939 = call "SW_Init_Array_of_Conditions.vi"("error in (no error)"=w1718) -> ("error out"=w1716:T41, "Array of conditions"=w1717:T6)  [unwired: 1 in]
        n940 = local read "Settings cluster (local)"() -> (w1722:T16)
        n941 = call "GET_Index_of_selected_Tree_element_and_N_Conditions.vi"("error in (no error)"=w1716, "TreeControl in"=w1721) -> ("error out"=w1719:errorcluster, "Index of selected element"=w1714:i32, "TreeControl out"=w1720:refnum<vi>)  [unwired: 6 in, 1 out]
        n942 = Index Array(array=w1717, index=w1714) -> (element=w1713:T7)
        n943 = Replace Array Subset(array=w1715, new element=w1713, index=w1714) -> (w1712:T6)
        n944 = call "DATA_Reorder_after_condition_modification.vi"("Array of conditions"=w1712) -> ("Reordered conditions array"=w1711:T7[])  [unwired: 2 in]
        n945 = call "SW_Generate_Full_Condition(s)_text.vi"("error in (no error)"=w1719, "Array of conditions in"=w1711, "Calibration parameters"=w1723, "TreeControl ref in"=w1720) -> ("error out"=w1705:errorcluster, "TreeControl ref out"=w1706:refnum<vi>)  [unwired: 6 in]
        n946 = Bundle By Name(cluster=w1722, "Conditions presets array"=w1711) -> (w1702:T16)
        n947 = local write "Array of conditions"(w1711) -> ()
        n948 = property class="Tree (strict)"(reference=w1706, error in=w1705, "Value"="") -> (error out=w1704:errorcluster)  [unwired: 1 out]
        n949 = local write "Settings cluster (local)"(w1702) -> ()
        n950 = global write "SW_Globals_2.2+.vi" "Settings cluster"(w1702) -> ()
        n951 = Enqueue Element(queue=w1708, element=CTL_Control_States."Check Reward condition(s)", error in (no error)=w1704) -> (queue out=w1707:refnum<queue>, error out=w1709:errorcluster)  [unwired: 1 in, 1 out]
        n952 = call "Set Parameters and data.vi"("Data"=w1702, "Parameter"=CTL_Parameter_transfer_name."All parameters") -> ()  [unwired: 9 in, 1 out]
      }
      frame "Check Reward condition(s)" {
        n953 = control-ref of="Reward and stimulation"() -> (w1735:refnum<vi>)
        n954 = call "GET_Index_of_selected_Tree_element_and_N_Conditions.vi"("error in (no error)"=w1734, "TreeControl in"=w1735) -> ("error out"=w1727:errorcluster, "Index of selected element"=w1733:i32, "Amount of conditions"=w1725:i32)  [unwired: 6 in, 1 out]
        n955 = Greater Than 0?(x=w1725) -> (x > 0?=w1732:bool)
        n956 = Greater Or Equal To 0?(x=w1733) -> (x >= 0?=w1731:bool)
        n957 = Build Array(w1732, w1731) -> (w1730:bool[])
        n958 = Boolean Array To Number(Boolean array=w1730) -> (number=w1729:u32)
        n959 = To Long Integer(number=w1729) -> (32bit integer=w1726:i32)
        n960 = case shown="3" w1726 {
          selector: w1726 -> [w1738 w1745 _]
          tunnel: w1725 -> [_ _ w1752]
          frame 0, Default {
            # "No elements selected, array is empty"
            n961 = feedback-in #1(w1738) -> ()
            n962 = feedback #1(-1) -> (w1739:i32)
            n963 = Not Equal?(x=w1739, y=w1738) -> (x != y?=w1737:bool)
            n964 = case shown="True" w1737 {
              frame False {
              }
              frame True {
                n965 = property on="Add Reward" class="Bool (strict)"("DisabledEnum"=T54."Enabled" ("Disabled")) -> ()  [unwired: 2 in, 2 out]
                n966 = property on="Modify Reward" class="Bool (strict)"("DisabledEnum"=T54."Disabled and Grayed Out" ("Disabled")) -> ()  [unwired: 2 in, 2 out]
                n967 = property on="Remove Reward" class="Bool (strict)"("DisabledEnum"=T54."Disabled and Grayed Out" ("Disabled")) -> ()  [unwired: 2 in, 2 out]
              }
            }
          }
          frame 1 {
            # "No elements selected, array is not empty"
            n968 = feedback-in #2(w1745) -> ()
            n969 = feedback #2(-1) -> (w1746:i32)
            n970 = Not Equal?(x=w1746, y=w1745) -> (x != y?=w1744:bool)
            n971 = case shown="True" w1744 {
              frame False {
              }
              frame True {
                n972 = property on="Add Reward" class="Bool (strict)"("DisabledEnum"=T54."Disabled and Grayed Out" ("f")) -> ()  [unwired: 2 in, 2 out]
                n973 = property on="Modify Reward" class="Bool (strict)"("DisabledEnum"=T54."Disabled and Grayed Out" ("Disabled")) -> ()  [unwired: 2 in, 2 out]
                n974 = property on="Remove Reward" class="Bool (strict)"("DisabledEnum"=T54."Disabled and Grayed Out" ("Disabled")) -> ()  [unwired: 2 in, 2 out]
              }
            }
          }
          frame 3 {
            # "Element selected, array is not empty"
            n975 = case shown="True" TRUE {
              tunnel: w1752 -> [_ w1758]
              frame False {
              }
              frame True {
                w1757 = 9  # Max number of conditions
                n976 = Less?(x=w1758, y=w1757) -> (x < y?=w1756:bool)
                n977 = Select(t=T54."Enabled" ("Disabled"), s=w1756, f=T54."Disabled and Grayed Out") -> (s? t:f=w1754:T54)
                n978 = property on="Add Reward" class="Bool (strict)"("DisabledEnum"=w1754) -> ()  [unwired: 2 in, 2 out]
                n979 = property on="Modify Reward" class="Bool (strict)"("DisabledEnum"=T54."Enabled" ("Disabled")) -> ()  [unwired: 2 in, 2 out]
                n980 = property on="Remove Reward" class="Bool (strict)"("DisabledEnum"=T54."Enabled" ("Disabled")) -> ()  [unwired: 2 in, 2 out]
              }
            }
          }
        }
      }
      frame "Save all settings" {
        n981 = global read "SW_Globals_2.2+.vi" "Paths"() -> (w1767:T68)
        n982 = Unbundle By Name(w1767) -> ("Program settings"=w1766:path)
        n983 = global read "SW_Globals_2.2+.vi" "Settings cluster"() -> (w1763:T16)
        n984 = call "SW_Save_Settings_2.vi"("error in (no error)"=w1761, "Parameter group to save"=T52 "All", "Settings cluster"=w1763, "Settings path in"=w1766) -> ("error out"=w1765:errorcluster)  [unwired: 5 in, 1 out]
      }
      frame "Save all settings to custom location" {
        n985 = global read "SW_Globals_2.2+.vi" "Paths"() -> (w1777:T68)
        n986 = call <vilib>:"Set Busy.vi"("error in (no error)"=w1783) -> ("error out"=w1778:errorcluster)  [unwired: 9 in, 1 out]
        n987 = Unbundle By Name(w1777) -> ("Folder"=w1776:path)
        n988 = Strip Path(path=w1776) -> (stripped path=w1775:path)  [unwired: 1 out]
        n989 = call "Save all settings"("start path"=w1775, "prompt"="Please enter save name and location", "button label"="Save", "default name"="Custom_settings", "error in"=w1778, "pattern (all files)"="*.trset", "pattern label"="Tracker settings") -> ("selected path"=w1781:path, "cancelled"=w1769:bool, "error out"=w1780:errorcluster)  [unwired: 5 in, 1 out]
        n990 = case shown="No Error" w1780 {
          selector: w1780 -> [w1789 w1800]
          tunnel: [w1792 w1799] -> w1784
          tunnel: w1781 -> [w1791 _]
          tunnel: w1769 -> [w1786 _]
          frame No Error {
            n991 = call-poly <userlib>:"Valid Path__ogtk.vi"("path"=w1791) -> ("valid"=w1790:bool)
            n992 = Not(x=w1786) -> (.not. x?=w1787:bool)
            n993 = And(x=w1787, y=w1790) -> (x .and. y?=w1788:bool)
            n994 = case shown="True" w1788 {
              tunnel: [w1793 w1798] -> w1792
              tunnel: w1791 -> [_ w1795]
              tunnel: w1789 -> [w1793 w1794]
              frame False {
              }
              frame True {
                n995 = global read "SW_Globals_2.2+.vi" "Settings cluster"() -> (w1796:T16)
                n996 = call "SW_Save_Settings_2.vi"("error in (no error)"=w1794, "Parameter group to save"=T52 "All", "Settings cluster"=w1796, "Settings path in"=w1795) -> ("error out"=w1798:errorcluster)  [unwired: 5 in, 1 out]
              }
            }
          }
          frame Error {
            n997 = call <vilib>:"Simple Error Handler.vi"("error in (no error)"=w1800) -> ("error out"=w1801:errorcluster)  [unwired: 4 in, 4 out]
            n998 = call <vilib>:"Clear Errors.vi"("error in (no error)"=w1801) -> ("error out"=w1799:errorcluster)  [unwired: 5 in, 1 out]
          }
        }
        n999 = call <vilib>:"Unset Busy.vi"("error in (no error)"=w1784) -> ("error out"=w1782:errorcluster)  [unwired: 10 in]
      }
      frame "Close App" {
        w1803 = 5.0 ("Timeout to Wait for Stop (s) (-1: no timeout)")
        w1828 = T79 128 items=["Flush Receive Buffer"=16, "Write Transmit Buffer to Device"=32, "Flush Receive Buffer (No I/O)"=64, "Flush Transmit Buffer"=128] ("Mask")
        n1000 = global read "SW_Globals_2.2+.vi" "Settings cluster"() -> (w1812:T16)
        n1001 = Unbundle By Name(w1812) -> ("Defaults.VISA Resource Name"=w1817:string)
        n1002 = disable-structure shown="Disabled" {
          disable-tunnel: [w1836 _] -> w1811
          disable-tunnel: w1803 -> [w1835 _]
          frame Disabled {
            n1003 = call "Stop Module.vi"("Timeout to Wait for Stop (s) (-1: no timeout)"=w1835) -> ("error out"=w1836:errorcluster)  [unwired: 10 in]
          }
          frame Enabled {
          }
        }
        n1004 = call "Prepare to Exit.vi"() -> ("error out"=w1809:errorcluster)  [unwired: 11 in]
        n1005 = call "Stop Module.vi"("Timeout to Wait for Stop (s) (-1: no timeout)"=w1803) -> ("error out"=w1808:errorcluster)  [unwired: 10 in]
        n1006 = call "Stop Module.vi"("Timeout to Wait for Stop (s) (-1: no timeout)"=w1803) -> ("error out"=w1802:errorcluster)  [unwired: 10 in]
        n1007 = call "HW_Acquisition_Stop.vi"("Error In"=w1815, "VISA resource name in"=w1817) -> ("Error Out"=w1805:errorcluster, "VISA resource name out"=w1816:refnum<visa-resource-name>)
        n1008 = Merge Errors(w1805, w1811, w1809, w1808, w1802) -> (w1810:errorcluster)
        n1009 = call "1.5s delay"("error in (no error)"=w1810) -> ("error out"=w1804:errorcluster)  [unwired: 10 in]
        n1010 = VISA Flush I/O Buffer(VISA resource name=w1816, mask (16)=w1828, error in (no error)=w1804) -> (VISA resource name out=w1829:refnum<visa-resource-name>, error out=w1830:errorcluster)
        n1011 = VISA Clear(VISA resource name=w1829, error in (no error)=w1830) -> (VISA resource name out=w1832:refnum<visa-resource-name>, error out=w1831:errorcluster)
        n1012 = VISA Close(VISA resource name=w1832, error in (no error)=w1831) -> (error out=w1833:errorcluster)
        n1013 = call <vilib>:"Clear Errors.vi"("error in (no error)"=w1833) -> ("error out"=w1825:errorcluster)  [unwired: 5 in, 1 out]
        n1014 = Get Notifier Status(notifier=w1826, error in (no error)=w1825) -> (notifier out=w1823:refnum<notifier>, current notification=w1822:T46, error out=w1824:errorcluster)  [unwired: 2 out]
        n1015 = Bundle By Name(cluster=w1822, "Stop and Exit"=TRUE) -> (w1821:T46)
        n1016 = Send Notification(notification=w1821, notifier=w1823, error in (no error)=w1824) -> (notifier out=w1819:refnum<notifier>, error out=w1806:errorcluster)
        n1017 = property class="App"() -> ("App.Kind"=w1818:T61)  [unwired: 2 in, 2 out]
        n1018 = call "IMAQ Dispose"("All Images? (No)"=TRUE, "error in (no error)"=w1806) -> ("error out"=w1813:errorcluster)  [unwired: 4 in]
        n1019 = case shown="\"invalid app kind\", Default" w1818 {
          tunnel: w1813 -> [w1838 w1841]
          tunnel: [w1837 w1841] -> w1807
          frame "invalid app kind", Default {
            # "Close FP only if app is compiled"
            n1020 = global read "SW_Globals_2.2+.vi" "All references"() -> (w1840:T36)
            n1021 = Unbundle By Name(w1840) -> ("Service references.This VI"=w1839:refnum<vi>)
            n1022 = invoke class="VI" method="FP.Close"(reference=w1839, error in=w1838) -> (error out=w1837:errorcluster)  [unwired: 1 in, 2 out]
          }
          frame "Development System" {
          }
        }
      }
    }
    n1023 = call "Error (IDL).vi"("Previous step"=w163, "Error In"=w165, "Queue In"=w167) -> ("Error Out"=w164:errorcluster, "Error data"=w162:variant, "Queue Out"=w166:refnum<queue>)  [unwired: 6 in]
    n1024 = node-c288(w164) -> ()  [unwired: 1 out]
  }
  n1025 = timed-loop {
    timing: w60 -> [_]
    timing-out: [_] -> w59
    tunnel: w23 -> [_]
    tunnel: w22 -> [w1857]
    border: "" -> [_]
    tunnel: [w1853] -> w27
    tunnel: [w1850] -> w26
    tunnel: [w1847] -> w28
    stop <- w1856 stop-if-true
    # "Data gathering and initial processing loop + recorded data streaming"
    n1026 = node-c288() -> (w1851:errorcluster)  [unwired: 1 in]
    n1027 = Get Notifier Status(notifier=w1857, error in (no error)=w1851) -> (current notification=w1848:T46, error out=w1852:errorcluster)  [unwired: 3 out]
    n1028 = Unbundle By Name(w1848) -> ("Acq. is ON"=w1855:bool, "Stop and Exit"=w1856:bool)
    n1029 = case shown="True" w1855 {
      tunnel: w1852 -> [w1859 w1918]
      tunnel: [w1860 w1912] -> w1854
      tunnel: [_ w1911] -> w1853
      tunnel: [_ w1910] -> w1850
      tunnel: [w1862 i64 1] -> w1849
      tunnel: w1848 -> [w1868 _]
      tunnel: [w1858 _] -> w1847
      frame False {
        # "This part in certain conditions will be used for offline data streaming from loaded files"
        n1030 = local read "Play/Pause"() -> (w1861:bool)
        n1031 = Unbundle By Name(w1868) -> ("Data loaded"=w1864:bool, "Offline mode"=w1866:bool, "Stop and Exit"=w1867:bool)
        n1032 = Not(x=w1867) -> (.not. x?=w1865:bool)
        n1033 = Compound Arithmetic op=AND(w1861, w1864, w1866, w1865) -> (w1863:bool)
        n1034 = case shown="True" w1863 {
          tunnel: [i64 101 w1876] -> w1862
          tunnel: [w1869 w1898] -> w1860
          tunnel: w1859 -> [w1869 w1898]
          tunnel: [_ w1887] -> w1858
          frame False {
            # "Some conditionas are not met"
          }
          frame True {
            # "Data loaded, oflline mode is on and we are good to stream loaded data"
            n1035 = local read "Timeline min&max indices"() -> (w1897:T26)
            n1036 = local read "Loaded.zones"() -> (w1880:i8[])
            n1037 = local read "Loaded.timeline"() -> (w1903:dbl[])
            n1038 = local read "Loaded.X"() -> (w1902:dbl[])
            n1039 = local read "Loaded.Y"() -> (w1901:dbl[])
            n1040 = local read "Loaded.alpha"() -> (w1900:dbl[])
            n1041 = local read "Loaded.speed"() -> (w1899:dbl[])
            n1042 = local read "Act. frame time, s"() -> (w1877:dbl)
            n1043 = Unbundle(w1897) -> ("Tl. min index"=w1894:i32, "Tl. max index"=w1884:i32)
            n1044 = local read "Playback speed"() -> (w1878:u16)
            n1045 = expression code="x * 8.333333"(w1877) -> (w1907:dbl)
            n1046 = local read "Cur. pos. slider index"() -> (w1886:i32)
            n1047 = local read "Update timeline index?"() -> (w1885:bool)
            n1048 = feedback #3(w1894) -> (w1881:i32)
            n1049 = Index Array(array=w1903, index=w1881) -> (element=w1893:dbl)
            n1050 = Index Array(array=w1902, index=w1881) -> (element=w1892:dbl)
            n1051 = Index Array(array=w1901, index=w1881) -> (element=w1891:dbl)
            n1052 = Index Array(array=w1900, index=w1881) -> (element=w1890:dbl)
            n1053 = Index Array(array=w1899, index=w1881) -> (element=w1889:dbl)
            n1054 = Index Array(array=w1880, index=w1881) -> (element=w1879:i8)
            n1055 = Build Array(w1893, w1892, w1891, w1890, w1889, w1879) -> (w1888:dbl[])
            n1056 = Increment(x=w1881) -> (x+1=w1883:i32)
            n1057 = Multiply(x=w1878, y=w1907) -> (x*y=w1873:dbl)
            n1058 = call <extravilib>:"Write.vi"("element"=w1888) -> ("channel"=w1887:T82)  [unwired: 8 in, 2 out]
            n1059 = feedback #4(0.0) -> (w1871:dbl)
            n1060 = Add(x=w1871, y=w1873) -> (x+y=w1872:dbl)
            n1061 = Select(t=w1886, s=w1885, f=w1883) -> (s? t:f=w1882:i32)
            n1062 = case shown="True" w1885 {
              frame False {
              }
              frame True {
                n1063 = local write "Update timeline index?"(FALSE ("Update timeline index?")) -> ()
              }
            }
            n1064 = Greater Or Equal?(x=w1882, y=w1884) -> (x >= y?=w1896:bool)
            n1065 = To Quad Integer(1:w1872) -> (0:w1906:i64)
            n1066 = Select(t=w1894, s=w1896, f=w1882) -> (s? t:f=w1895:i32)
            n1067 = feedback-in #3(w1895) -> ()
            n1068 = In Range and Coerce(upper limit=i64 1000, x=w1906, lower limit=i64 1) -> (coerced(x)=w1876:i64)  [unwired: 1 out]
            n1069 = Subtract(x=w1872, y=w1876) -> (x-y=w1874:dbl)
            n1070 = feedback-in #4(w1874) -> ()
          }
        }
      }
      frame True {
        # "Data gathering in online mode happens here"
        n1071 = local read "VISA resource name"() -> (w1916:refnum<visa-resource-name>)
        n1072 = call "HW_Get_data_flow_from_serial_port.vi"("error in"=w1918, "VISA resource name in"=w1916) -> ("Not empty?"=w1917:bool, "error out"=w1913:errorcluster, "Timestamp"=w1914:timestamp, "Data"=w1915:string)  [unwired: 2 in, 1 out]
        n1073 = case shown="True" w1917 {
          tunnel: w1915 -> [_ w1934]
          tunnel: w1914 -> [_ w1933]
          tunnel: w1913 -> [w1919 w1937]
          tunnel: [w1919 w1928] -> w1912
          tunnel: [_ w1923] -> w1911
          tunnel: [_ w1922] -> w1910
          frame False {
          }
          frame True {
            n1074 = global read "SW_Globals_2.2+.vi" "Settings cluster"() -> (w1925:T16)
            n1075 = local read "Ports IO config"() -> (w1931:bool[])
            n1076 = local read "SB size"() -> (w1924:u8)
            n1077 = feedback #5() -> (w1935:string)
            n1078 = Concatenate Strings(w1935, w1934) -> (w1932:string)
            n1079 = local read "Calibration parameters"() -> (w1921:T23)
            n1080 = Unbundle By Name(w1925) -> ("IO parameters.IO inversion config."=w1930:u16)
            n1081 = call "FL_Decode_RAW_to_DEC_2.vi"("SB size (loc. var. only)"=w1924, "IO ports config"=w1931, "Input string"=w1932, "Input timestamp"=w1933, "IO inversion config."=w1930, "Error In"=w1937) -> ("Output string leftover"=w1936:string, "DEC output cluster"=w1927:T83, "Error Out"=w1929:errorcluster)
            n1082 = feedback-in #5(w1936) -> ()
            n1083 = Unbundle By Name(w1927) -> ("Frame OK"=w1926:bool)
            n1084 = local read "Frame #"() -> (w1920:u32)
            n1085 = case shown="True" w1926 {
              tunnel: w1927 -> [_ w1966]
              tunnel: w1929 -> [w1938 w1941]
              tunnel: [w1938 w1941] -> w1928
              tunnel: w1925 -> [_ w1963]
              tunnel: w1924 -> [_ w1959]
              tunnel: [_ w1950] -> w1923
              tunnel: [_ w1943] -> w1922
              tunnel: w1921 -> [_ w1953]
              tunnel: w1920 -> [_ w1945]
              frame False {
              }
              frame True {
                n1086 = Unbundle By Name(w1953) -> ("True frame time, s"=w1952:dbl)
                n1087 = Unbundle By Name(w1963) -> ("Geometry.Bridge H. offset"=w1965:sgl, "Geometry.Bridge V. offset"=w1964:sgl, "Geometry.Magnets orientation"=w1940:sgl, "Geometry.Twisted neck"=w1957:bool, "Geometry.Bridge swap"=w1958:bool)
                n1088 = local read "Pre-filter params."() -> (w1954:T28)
                n1089 = Increment(x=w1945) -> (x+1=w1944:u32)
                n1090 = local write "Frame #"(w1944) -> ()
                n1091 = First Call?() -> (First Call?: T/F=w1955:bool)
                n1092 = Equal To 0?(x=w1940) -> (x = 0?=w1939:bool)
                n1093 = call "FL_Adjust_raw_magnets_coords.vi"("Offset H."=w1965, "Offset V."=w1964, "Alternative magnets orientation"=w1939, "DEC cluster in"=w1966) -> ("DEC cluster out"=w1962:T83)  [unwired: 3 in]
                n1094 = call "FL_DEC_split_3_and_prefilter_(online).vi"("Initialize? (F)"=w1955, "Pre-filter params."=w1954, "DEC input cluster"=w1962) -> ("Magnets coords raw"=w1946:T84, "Magnets coords"=w1961:cluster{"X1":dbl, "Y1":dbl, "X2":dbl, "Y2":dbl}, "TTLs"=w1948:cluster{"TTL input":i16, "TTL output":i16}, "Times"=w1949:T85)  [unwired: 3 in]
                n1095 = call "FL_Calculate_Coordinates_Diff_R_Center.vi"("Frame time, s"=w1952, "Magnets coords in"=w1961) -> ("Output cluster of data"=w1960:T86)  [unwired: 1 in]
                n1096 = call "CALC_Phi_theta_etc_3_(online).vi"("Current frame #"=w1944, "Twisted neck"=w1957, "Use alternative magnets orientation"=w1939, "Bridge swap"=w1958, "SB size"=w1959, "Input cluster of data"=w1960) -> ("Animal coordinates"=w1947:T25)  [unwired: 1 in]
                n1097 = Bundle By Name(cluster=T80 {"Times"={"ms since ON"=0, "delta time"=0, "Frame timestamp"=timestamp(0 s since 1904-01-01)}, "TTLs"={"TTL input"=0, "TTL output"=0}, "Animal coordinates"={"R from center"=0.0, "phi (mouse angular position in the cage)"=0.0, "alpha (mouse rot. angle)"=0.0, "X"=0.0, "Y"=0.0, "theta (from center towards mouse)"=0.0, "beta (cage rot. against mouse)"=0.0, "w (mouse angle to wall)"=0.0, "Speed (filtered)"=0.0}, "Magnets coords raw"={"X1 raw"=0.0, "Y1 raw"=0.0, "X2 raw"=0.0, "Y2 raw"=0.0}, "Measurements and statistics"={"Zone #"=0, "Histogram"=[], "Running, perc. of time"=0.0, "Run, meters"=0.0, "Avg. speed"=0.0}} ("Data in"), "Times"=w1949, "TTLs"=w1948, "Animal coordinates"=w1947, "Magnets coords raw"=w1946) -> (w1942:T80)
                n1098 = call <extravilib>:"Write.vi"("element"=w1947) -> ("channel"=w1950:T87)  [unwired: 8 in, 2 out]
                n1099 = call <extravilib>:"Write.vi"("size (unlimited)"=250, "element"=w1942) -> ("channel"=w1943:T88)  [unwired: 7 in, 2 out]
              }
            }
          }
        }
      }
    }
    n1100 = node-c288(w1854, w1849) -> ()  [unwired: 1 out]
  }
  n1101 = node-c288(w19, i64 499 ("Period"), 100 ("Priority"), "Whatchdog" ("Structure Name"), w37) -> (w43:T48)
  n1102 = node-c288(w19, i64 2 ("Period"), 45000 ("Priority"), "Proc_and_save" ("Structure Name"), w24) -> (w35:T48)
  n1103 = node-c288(w19, i64 53 ("Period"), 1000 ("Priority"), "UI_response" ("Structure Name"), w17) -> (w65:T48)
  n1104 = timed-loop {
    timing: w43 -> [_]
    timing-out: [_] -> w42
    tunnel: w22 -> [w2001]
    tunnel: w23 -> [w1990]
    tunnel: w36 -> [w1995]
    stop <- w1998 stop-if-true
    # "Whatchdog and slow stuff loop"
    n1105 = node-c288() -> (w2000:errorcluster, w1996:i64)  [unwired: 1 in]
    n1106 = Get Notifier Status(notifier=w2001, error in (no error)=w2000) -> (current notification=w1999:T46, error out=w1997:errorcluster)  [unwired: 3 out]
    n1107 = local read "UI update period"() -> (w1993:i64)
    n1108 = call "SW_Get_CPU_load.vi"("error in (no error)"=w1997, "Buffer length, sec"=5.0, "Scan interval, ms"=w1996, "CPU monitor .NET reference in"=w1995) -> ("error out"=w1989:errorcluster, "Historical CPU load, %"=w1988:sgl)  [unwired: 2 out]
    n1109 = call "SW_Adjust_UI_draw_interwal.vi"("UI update period (l.v.o.) in"=w1993, "Historical CPU load, %"=w1988) -> ("Updated?"=w1991:bool, "UI update period (l.v.o.) out"=w1992:i64)
    n1110 = Unbundle By Name(w1999) -> ("Stop and Exit"=w1998:bool, "Acq. is ON"=w1984:bool, "Offline mode"=w1985:bool, "Recording now"=w1973:bool)
    n1111 = local write "CPU load"(w1988) -> ()
    n1112 = local write "UI update period"(w1992) -> ()
    n1113 = case shown="True" w1991 {
      tunnel: w1990 -> [w2014 w2019]
      tunnel: w1989 -> [w2015 w2018]
      tunnel: [w2015 w2017] -> w1986
      tunnel: [w2014 w2016] -> w1976
      frame False {
        # "No update"
      }
      frame True {
        # "Update trace length"
        n1114 = Enqueue Element(queue=w2019, element=CTL_Control_States."Upd. trace length", error in (no error)=w2018) -> (queue out=w2016:refnum<queue>, error out=w2017:errorcluster)  [unwired: 1 in, 1 out]
      }
    }
    n1115 = Not(x=w1985) -> (.not. x?=w1983:bool)
    n1116 = And(x=w1984, y=w1983) -> (x .and. y?=w1974:bool)
    n1117 = local read "Since track start"() -> (w1977:dbl)
    n1118 = global read "SW_Globals_2.2+.vi" "All references"() -> (w1987:T36)
    n1119 = global read "SW_Globals_2.2+.vi" "Settings cluster"() -> (w1982:T16)
    n1120 = Unbundle By Name(w1982) -> ("Recording and saving.\"Stop at\" enabled"=w1981:bool, "Recording and saving.Stop at"=w1978:dbl)
    n1121 = call "UI_Set_Slider_values_when_online.vi"("error in (no error)"=w1986, "Online? (F)"=w1974, "Since track start"=w1977, "All references"=w1987) -> ("error out"=w1979:errorcluster)  [unwired: 7 in]
    n1122 = Compound Arithmetic op=AND(w1974, w1973, w1981) -> (w1975:bool)
    n1123 = case shown="True" w1975 {
      tunnel: [w2002 w2003] -> w1980
      tunnel: w1979 -> [w2002 w2005]
      tunnel: w1978 -> [_ w2007]
      tunnel: w1977 -> [_ w2008]
      tunnel: w1976 -> [_ w2004]
      frame False {
      }
      frame True {
        n1124 = Greater Or Equal?(x=w2008, y=w2007) -> (x >= y?=w2006:bool)
        n1125 = case shown="True" w2006 {
          tunnel: [w2009 w2013] -> w2003
          tunnel: w2005 -> [w2009 w2012]
          tunnel: w2004 -> [_ w2011]
          frame False {
          }
          frame True {
            n1126 = Enqueue Element(queue=w2011, element=CTL_Control_States."Stop Recording", error in (no error)=w2012) -> (error out=w2013:errorcluster)  [unwired: 1 in, 2 out]
          }
        }
      }
    }
    n1127 = node-c288(w1980) -> ()  [unwired: 1 out]
  }
  n1128 = timed-loop {
    timing: w35 -> [_]
    timing-out: [_] -> w34
    tunnel: w22 -> [w2045]
    tunnel: w26 -> [w2044]
    tunnel: w23 -> [w2031]
    tunnel: [w2027] -> w25
    stop <- w2028 stop-if-true
    # "Data processing, saving and calibration loop"
    n1129 = node-c288() -> (w2034:errorcluster)  [unwired: 1 in]
    n1130 = call <extravilib>:"Read.vi"("timeout in ms (-1)"=563, "channel"=w2044) -> ("element"=w2036:T80, "timed out?"=w2039:bool, "count"=w2038:i32)  [unwired: 5 in, 2 out]
    n1131 = Get Notifier Status(notifier=w2045, error in (no error)=w2034) -> (notifier out=w2030:refnum<notifier>, current notification=w2029:T46, error out=w2035:errorcluster)  [unwired: 2 out]
    n1132 = Not(x=w2039) -> (.not. x?=w2042:bool)
    n1133 = Equal To 0?(x=w2038) -> (x = 0?=w2041:bool)
    n1134 = Unbundle By Name(w2029) -> ("Stop and Exit"=w2028:bool)
    n1135 = Not(x=w2028) -> (.not. x?=w2040:bool)
    n1136 = Compound Arithmetic op=AND(w2042, w2041, w2040) -> (w2037:bool)
    n1137 = case shown="True" w2037 {
      tunnel: w2036 -> [_ w2056]
      tunnel: w2034 -> [w2046 w2055]
      tunnel: [w2046 w2054] -> w2032
      tunnel: w2031 -> [_ w2053]
      tunnel: w2030 -> [_ w2049]
      tunnel: w2029 -> [_ w2048]
      tunnel: [_ w2047] -> w2027
      frame False {
      }
      frame True {
        n1138 = Unbundle By Name(w2048) -> ("Calibration mode"=w2052:bool)
        n1139 = feedback-in #6(w2052) -> ()
        n1140 = feedback #6(FALSE ("Calibration mode")) -> (w2050:bool)
        n1141 = case shown="False" w2052 {
          tunnel: w2056 -> [w2077 w2093]
          tunnel: w2055 -> [w2078 w2097]
          tunnel: [w2058 w2089] -> w2054
          tunnel: w2053 -> [w2074 w2095]
          tunnel: w2050 -> [_ w2086]
          tunnel: w2049 -> [w2076 w2091]
          tunnel: [w2062 _] -> w2047
          frame False {
            # "Regular samples are recorded/tested here"
            n1142 = local read "IO parameters"() -> (w2079:T22)
            n1143 = call "FL_React_on_incoming_TTLs.vi"("IO parameters in"=w2079, "Data in"=w2077, "Notifier in"=w2076, "Queue in"=w2074, "error in (no error)"=w2078) -> ("TTL received at (HW)"=w2070:u32, "TTL received at (SW)"=w2075:timestamp, "Data out"=w2067:T80, "Notifier out"=w2072:refnum<notifier>, "error out"=w2066:errorcluster)  [unwired: 5 in, 1 out]
            n1144 = local write "TTL in time (SW)"(w2075) -> ()
            n1145 = local write "TTL in time (HW)"(w2070) -> ()
            n1146 = local read "Stats parameters (online)"() -> (w2069:T1)
            n1147 = local read "Reset barplot"() -> (w2068:bool)
            n1148 = call "GET_Statistics_(online).vi"("Animal coordinates in"=w2067, "Stats parameters (online)"=w2069, "Reset? (F)"=w2068, "error in (no error)"=w2066) -> ("Animal coordinates out"=w2060:T80, "error out"=w2065:T41)  [unwired: 3 in]
            n1149 = Get Notifier Status(notifier=w2072, error in (no error)=w2065) -> (current notification=w2073:T89, error out=w2064:errorcluster)  [unwired: 3 out]
            n1150 = Unbundle By Name(w2073) -> ("Recording now"=w2071:bool)
            n1151 = case shown="True" w2071 {
              tunnel: w2064 -> [w2080 w2084]
              tunnel: [w2080 w2081] -> w2059
              tunnel: w2060 -> [_ w2083]
              frame False {
              }
              frame True {
                n1152 = local read "Key_pressed"() -> (w2082:string)
                n1153 = local read "TDMS ref."() -> (w2085:refnum<k34>)
                n1154 = call "PR_Write_tracker_stream_to_TDMS.vi"("error in (no error)"=w2084, "Key_pressed"=w2082, "Data in"=w2083, "TDMS ref. in"=w2085) -> ("error out"=w2081:errorcluster)  [unwired: 6 in, 1 out]
              }
            }
            n1155 = Unbundle By Name(w2060) -> ("Measurements and statistics"=w2063:T81)
            n1156 = call "Send Frame.vi"("error in (no error)"=w2059, "Data in"=w2060) -> ("error out"=w2061:errorcluster)  [unwired: 9 in]
            n1157 = call "Send frame.vi"("error in (no error)"=w2059, "Coordinates and speed"=w2060) -> ("error out"=w2057:errorcluster)  [unwired: 9 in]
            n1158 = call <extravilib>:"Write.vi"("element"=w2063) -> ("channel"=w2062:T90)  [unwired: 8 in, 2 out]
            n1159 = Merge Errors(w2061, w2057) -> (w2058:errorcluster)
          }
          frame True {
            # "Calibration samples acquisition happens here"
            n1160 = local read "Progress Bar Dialog"() -> (w2096:refnum<class "Progress Bar Dialog.lvclass">)
            n1161 = local read "Calibration samples"() -> (w2092:i32)
            n1162 = Not(x=w2086) -> (.not. x?=w2094:bool)
            n1163 = call "FL_Collect_Timings_Data.vi"("Control"=w2095, "Progress Bar Dialog in"=w2096, "States"=w2091, "Calibration buffer length, samples"=w2092, "Reset"=w2094, "error in (no error)"=w2097, "Data in"=w2093) -> ("Calibration HW timings"=w2088:u32[], "Calibration SW timings"=w2087:dbl[], "Done"=w2090:bool, "error out"=w2089:errorcluster)  [unwired: 5 in]
            n1164 = case shown="True" w2090 {
              tunnel: w2088 -> [_ w2099]
              tunnel: w2087 -> [_ w2098]
              frame False {
              }
              frame True {
                n1165 = local write "Calibration HW timings"(w2099) -> ()
                n1166 = local write "Calibration SW timings"(w2098) -> ()
              }
            }
          }
        }
      }
    }
    n1167 = Merge Errors(w2032, w2035) -> (w2033:errorcluster)
    n1168 = node-c288(w2033) -> ()  [unwired: 1 out]
  }
  n1169 = timed-loop {
    timing: w54 -> [_]
    timing-out: [_] -> w53
    tunnel: w23 -> [_]
    tunnel: w22 -> [w2129]
    tunnel: w27 -> [w2128]
    tunnel: w28 -> [w2114]
    tunnel: w25 -> [w2107]
    stop <- w2117 stop-if-true
    # "UI drawings and plots update loop"
    n1170 = node-c288() -> (w2105:errorcluster)  [unwired: 1 in]
    n1171 = Get Notifier Status(notifier=w2129, error in (no error)=w2105) -> (current notification=w2130:T46, error out=w2116:errorcluster)  [unwired: 3 out]
    n1172 = local read "Play/Pause"() -> (w2119:bool)
    n1173 = Unbundle By Name(w2130) -> ("Calibration mode"=w2106:bool, "Updating layout"=w2109:bool, "Offline mode"=w2112:bool, "Data loaded"=w2118:bool, "Stop and Exit"=w2117:bool)
    n1174 = Not(x=w2109) -> (.not. x?=w2108:bool)
    n1175 = Not(x=w2117) -> (.not. x?=w2125:bool)
    n1176 = Select(t=0, s=w2112, f=563 ("timeout in ms (-1)")) -> (s? t:f=w2111:i32)
    n1177 = call <extravilib>:"Read.vi"("channel"=w2128, "timeout in ms (-1)"=w2111) -> ("element"=w2127:T25, "count"=w2121:i32, "timed out?"=w2126:bool)  [unwired: 4 in, 3 out]
    n1178 = Not(x=w2126) -> (.not. x?=w2123:bool)
    n1179 = Equal To 0?(x=w2121) -> (x = 0?=w2124:bool)
    n1180 = Compound Arithmetic op=AND(w2119, w2123, w2124, w2125, w2108) -> (w2122:bool)
    n1181 = case shown="False" w2122 {
      tunnel: w2127 -> [_ w2214]
      tunnel: w2119 -> [w2131 _]
      tunnel: w2118 -> [w2140 _]
      tunnel: w2112 -> [w2139 _]
      tunnel: w2117 -> [w2138 _]
      tunnel: w2116 -> [w2136 w2218]
      tunnel: [w2135 w2217] -> w2115
      tunnel: w2114 -> [w2133 _]
      tunnel: w2108 -> [w2132 _]
      tunnel: w2107 -> [_ w2213]
      tunnel: w2106 -> [_ w2206]
      frame False {
        # "Offline stuff here"
        n1182 = Not(x=w2138) -> (.not. x?=w2137:bool)
        n1183 = Compound Arithmetic op=AND(w2140, w2139, w2137, w2132) -> (w2134:bool)
        n1184 = case shown="True" w2131 {
          tunnel: w2136 -> [w2151 w2188]
          tunnel: [w2150 w2187] -> w2135
          tunnel: w2134 -> [w2144 w2186]
          tunnel: w2133 -> [w2149 _]
          frame True {
            # "Draw this when Play is active"
            n1185 = call <extravilib>:"Read.vi"("channel"=w2149, "timeout in ms (-1)"=563) -> ("element"=w2141:dbl[], "count"=w2146:i32, "timed out?"=w2147:bool)  [unwired: 4 in, 3 out]
            n1186 = Equal To 0?(x=w2146) -> (x = 0?=w2143:bool)
            n1187 = Not(x=w2147) -> (.not. x?=w2142:bool)
            n1188 = Compound Arithmetic op=AND(w2142, w2143, w2144) -> (w2145:bool)
            n1189 = case shown="True" w2145 {
              tunnel: w2151 -> [w2152 w2177]
              tunnel: [w2152 w2181] -> w2150
              tunnel: w2141 -> [_ w2178]
              frame False {
              }
              frame True {
                n1190 = local read "Timeline min&max"() -> (w2175:cluster{"Tl. min":dbl, "TL. max":dbl})
                n1191 = Index Array(array=w2178) -> (element #1=w2155:dbl, element #2=w2171:dbl, element #3=w2170:dbl, element #4=w2169:dbl, element #5=w2157:dbl, element #6=w2164:dbl)  [unwired: 6 in]
                n1192 = Unbundle(w2175) -> ("Tl. min"=w2174:dbl, "TL. max"=w2173:dbl)
                n1193 = To Time Stamp(1:w2155) -> (0:w2166:timestamp)
                n1194 = local write "Since track start"(w2155) -> ()
                n1195 = Build Array(w2157) -> (w2167:dbl[])
                n1196 = Bundle By Name(cluster=T25 {"R from center"=0.0, "phi (mouse angular position in the cage)"=0.0, "alpha (mouse rot. angle)"=0.0, "X"=0.0, "Y"=0.0, "theta (from center towards mouse)"=0.0, "beta (cage rot. against mouse)"=0.0, "w (mouse angle to wall)"=0.0, "Speed (filtered)"=0.0} ("Animal coordinates and speed"), "X"=w2171, "Y"=w2170, "alpha (mouse rot. angle)"=w2169, "Speed (filtered)"=w2157) -> (w2168:T25)
                n1197 = Bundle("Tl. min"=w2174, "TL. max"=w2173, "Numeric"=w2155) -> (w2176:T91)  [unwired: 1 in]
                n1198 = local write "Timeline"(w2176) -> ()
                n1199 = Bundle By Name("t0"=w2166, "Y"=w2167) -> (w2165:waveform(dbl))  [unwired: 1 in]
                n1200 = local read "Diagram (generated)"() -> (w2185:T15)
                n1201 = local read "Reset buffers?"() -> (w2180:bool)
                n1202 = local read "Track show state"() -> (w2183:u32)
                n1203 = local read "Overlays cluster"() -> (w2182:T27)
                n1204 = local write "Mouse speed"(w2165) -> ()
                n1205 = local read "Mouse drawing parameters"() -> (w2153:T2)
                n1206 = local write "Current position"(w2168) -> ()
                n1207 = call "DRAW_Mouse_DAQmx_w_overlay.vi"("Overlay track show state"=w2183, "Reset buffers? (F)"=w2180, "Overlays cluster"=w2182, "Error In (no error)"=w2177, "Mouse position"=w2168, "Mouse drawing parameters"=w2153, "Image In"=w2185) -> ("Error Out"=w2181:errorcluster, "Reset buffers out"=w2179:bool, "Image Out"=w2184:T15)  [unwired: 1 in]
                n1208 = To Byte Integer(number=w2164) -> (8bit integer=w2159:i8)
                n1209 = local write "Diagram (display)"(w2184) -> ()
                n1210 = local write "Mouse speed, mm/s"(w2157) -> ()
                n1211 = local write "Reset buffers?"(w2179) -> ()
                n1212 = Decrement(x=w2159) -> (x-1=w2162:i8)
                n1213 = local read "Start time (SW)"() -> (w2156:timestamp)
                n1214 = Replace Array Subset(array=bool[] [FALSE, FALSE, FALSE, FALSE, FALSE, FALSE, FALSE, FALSE, FALSE, FALSE, FALSE, FALSE, FALSE, FALSE, FALSE, FALSE], new element=TRUE ("new element/subarray"), index=w2162) -> (w2160:bool[])
                n1215 = Add(x=w2155, y=w2156) -> (x+y=w2154:timestamp)
                n1216 = local write "Current Time"(w2154) -> ()
                n1217 = Array To Cluster(array=w2160) -> (cluster=w2158:T92)
                n1218 = local write "Current zone"(w2158) -> ()
              }
            }
          }
          frame False {
            # "Draw this when Play is Off"
            n1219 = case shown="True" w2186 {
              tunnel: w2188 -> [w2191 w2196]
              tunnel: [w2191 w2195] -> w2187
              frame False {
                n1220 = Get Date/Time In Seconds() -> (seconds since 1Jan1904=w2190:timestamp)
                n1221 = local write "Current Time"(w2190) -> ()
                n1222 = Wait Until Next ms Multiple(millisecond multiple=u32 500) -> ()  [unwired: 1 out]
              }
              frame True {
                n1223 = local read "Mouse drawing parameters"() -> (w2201:T2)
                n1224 = local read "Diagram (generated)"() -> (w2200:T15)
                n1225 = local read "Track show state"() -> (w2198:u32)
                n1226 = local read "Overlays cluster"() -> (w2197:T27)
                n1227 = local read "Current position"() -> (w2192:T25)
                n1228 = local read "Reset buffers?"() -> (w2193:bool)
                n1229 = call "DRAW_Mouse_DAQmx_w_overlay.vi"("Overlay track show state"=w2198, "Reset buffers? (F)"=w2193, "Overlays cluster"=w2197, "Error In (no error)"=w2196, "Mouse position"=w2192, "Mouse drawing parameters"=w2201, "Image In"=w2200) -> ("Error Out"=w2195:errorcluster, "Reset buffers out"=w2194:bool, "Image Out"=w2199:T15)  [unwired: 1 in]
                n1230 = local write "Diagram (display)"(w2199) -> ()
                n1231 = local write "Reset buffers?"(w2194) -> ()
              }
            }
          }
        }
      }
      frame True {
        # "Online activities here (Play or Record)"
        n1232 = Not(x=w2206) -> (.not. x?=w2205:bool)
        n1233 = call <extravilib>:"Read.vi"("channel"=w2213, "timeout in ms (-1)"=563) -> ("element"=w2212:T81, "element valid?"=w2211:bool, "timed out?"=w2207:bool)  [unwired: 4 in, 3 out]
        n1234 = Not(x=w2207) -> (.not. x?=w2208:bool)
        n1235 = local read "Mouse drawing parameters"() -> (w2222:T2)
        n1236 = local read "Diagram (generated)"() -> (w2224:T15)
        n1237 = local read "Start time (SW)"() -> (w2220:timestamp)
        n1238 = Compound Arithmetic op=AND(w2211, w2208, w2205) -> (w2209:bool)
        n1239 = Get Date/Time In Seconds() -> (seconds since 1Jan1904=w2202:timestamp)
        n1240 = Subtract(x=w2202, y=w2220) -> (x-y=w2216:dbl)
        n1241 = local write "Since track start"(w2216) -> ()
        n1242 = Unbundle By Name(w2214) -> ("Speed (filtered)"=w2204:dbl)
        n1243 = To Time Stamp(1:w2216) -> (0:w2219:timestamp)
        n1244 = call "SW_Draw_mouse_DAQmx.vi"("Size of the image (480x480)"=T73 {"Numeric Control"=480.0, "Numeric Control"=480.0}, "Error In (no error)"=w2218, "Mouse position"=w2214, "Mouse drawing parameters"=w2222, "Image In"=w2224) -> ("Error Out"=w2217:errorcluster, "Image Out"=w2223:T15)  [unwired: 2 in]
        n1245 = Build Array(w2204) -> (w2221:dbl[])
        n1246 = Bundle By Name("t0"=w2219, "Y"=w2221) -> (w2203:waveform(dbl))  [unwired: 1 in]
        n1247 = case shown="True" w2209 {
          tunnel: w2212 -> [_ w2232]
          tunnel: w2204 -> [_ w2226]
          tunnel: w2203 -> [_ w2231]
          frame False {
          }
          frame True {
            n1248 = Unbundle By Name(w2232) -> ("Zone #"=w2239:i8, "Histogram"=w2236:dbl[], "Running, perc. of time"=w2234:dbl, "Run, meters"=w2233:dbl, "Avg. speed"=w2230:dbl)
            n1249 = local read "Hist. X axis"() -> (w2235:dbl[])
            n1250 = Decrement(x=w2239) -> (x-1=w2243:i8)
            n1251 = local write "Average speed, mm/s"(w2230) -> ()
            n1252 = local write "Running, perc. of time"(w2234) -> ()
            n1253 = Bundle By Name(cluster=T32 {"X Values"=[15.0, 45.0, 75.0, 105.0, 135.0, 165.0, 195.0, 225.0, 255.0, 285.0], "Histogram: h(x)"=[-1.0, -1.0, 0.0, 1.0, 2.0, 1.0, 0.0, -1.0, -1.0, -1.0]} ("XY Graph - Light"), "X Values"=w2235, "Histogram: h(x)"=w2236) -> (w2237:T32)
            n1254 = Replace Array Subset(array=bool[] [FALSE, FALSE, FALSE, FALSE, FALSE, FALSE, FALSE, FALSE, FALSE, FALSE, FALSE, FALSE, FALSE, FALSE, FALSE, FALSE], new element=TRUE ("new element/subarray"), index=w2243) -> (w2241:bool[])
            n1255 = local write "Mouse speed"(w2231) -> ()
            n1256 = Array To Cluster(array=w2241) -> (cluster=w2240:T92)
            n1257 = local write "Histograms"(w2237) -> ()
            n1258 = local write "Current zone"(w2240) -> ()
            n1259 = local write "Run distance, m"(w2233) -> ()
            n1260 = local read "Speed threshold"() -> (w2227:dbl)
            n1261 = Greater?(x=w2226, y=w2227) -> (0:w2225:bool)
            n1262 = Select(t=w2226, s=w2225, f=0.0) -> (s? t:f=w2228:dbl)
            n1263 = local write "Mouse speed, mm/s"(w2228) -> ()
          }
        }
        n1264 = local write "Current Time"(w2202) -> ()
        n1265 = local write "Diagram (display)"(w2223) -> ()
      }
    }
    n1266 = local read "UI update period"() -> (w2120:i64)
    n1267 = node-c288(w2115, w2120) -> ()  [unwired: 1 out]
  }
  n1268 = timed-loop {
    timing: w65 -> [_]
    timing-out: [_] -> w64
    tunnel: w23 -> [w2257]
    tunnel: w22 -> [w2256]
    tunnel: w13 -> [w2252]
    tunnel: [w2251] -> w12
    stop <- w2258 stop-if-true
    # "UI response loop"
    n1269 = node-c288() -> (w2254:errorcluster)  [unwired: 1 in]
    n1270 = event shown="[2] Menu Selection (User)" {
      selector: w2252 -> [_ _ _ _ _ _ _ _ _ _ _ _ _ _ _ _ _ _ _ _ _ _ _ _ _ _ _ _ _]
      dyn-events: [_ _ _ _ _ _ _ _ _ _ _ _ _ _ _ _ _ _ _ _ _ _ _ _ _ _ _ _ _] -> w2251
      timeout: _ -> [_ _ _ _ _ _ _ _ _ _ _ _ _ _ _ _ _ _ _ _ _ _ _ _ _ _ _ _ _]
      tunnel: [_ TRUE w2272 _ _ _ _ _ _ _ _ _ _ _ _ _ _ _ _ _ _ _ _ _ _ _ _ _ _] -> w2258
      tunnel: w2257 -> [_ w2268 w2273 w2373 w2383 w2389 w2403 w2417 w2421 _ w2494 w2519 w2524 w2529 w2534 _ _ w2577 _ w2588 w2623 w2640 w2652 w2654 _ w2665 w2681 _ _]
      tunnel: w2256 -> [_ _ _ _ _ _ _ _ _ _ _ _ _ _ _ _ _ _ _ w2585 w2620 _ _ _ _ _ _ _ _]
      tunnel: w2254 -> [w2260 w2266 w2271 w2366 w2377 w2387 w2401 w2415 w2428 w2461 w2493 w2521 w2526 w2531 w2536 w2545 w2568 w2573 w2578 w2584 w2619 w2638 w2650 w2653 w2660 w2664 w2680 w2683 w2694]
      tunnel: [w2259 w2265 w2270 w2367 w2376 w2386 w2396 w2410 w2419 w2460 w2479 w2520 w2525 w2530 w2535 w2537 w2567 w2574 w2578 w2586 w2621 w2637 w2649 w2656 w2660 w2663 w2677 w2682 w2693] -> w2253
      event Timeout {
        n1271 = event-data() -> ()  [unwired: 1 in, 3 out]
        n1272 = global read "SW_Globals_2.2+.vi" "All references"() -> (w2262:T36)
        n1273 = Get Date/Time In Seconds() -> (seconds since 1Jan1904=w2263:timestamp)
        n1274 = Unbundle By Name(w2262) -> ("Indicators references.Current Time"=w2261:refnum<vi>)
        n1275 = property class="AbsTime (strict)"(reference=w2261, error in=w2260, "Value"=w2263) -> (error out=w2259:errorcluster)  [unwired: 1 out]
      }
      event Panel Close? {
        n1276 = event-data() -> ()  [unwired: 1 in, 4 out]
        n1277 = Enqueue Element(queue=w2268, element=CTL_Control_States."Close App", error in (no error)=w2266) -> (error out=w2265:errorcluster)  [unwired: 1 in, 2 out]
        n1278 = event-data("Discard?"=TRUE) -> ()  [unwired: 1 in, 1 out]
      }
      event Menu Selection (User) {
        n1279 = event-data() -> ("ItemTag"=w2274:string)  [unwired: 1 in, 6 out]
        n1280 = case shown="\"Exit\"" w2274 {
          tunnel: w2273 -> [_ w2278 w2287 w2293 w2302 w2308 w2312 w2316 w2320 w2324 w2328 w2332 w2336 _ w2342 w2346 w2350 _]
          tunnel: [_ TRUE _ _ _ _ _ _ _ _ _ _ _ _ _ _ _ _] -> w2272
          tunnel: w2271 -> [w2275 w2280 w2285 w2294 w2303 w2306 w2310 w2314 w2318 w2322 w2326 w2330 w2334 w2338 w2340 w2344 w2348 w2356]
          tunnel: [w2275 w2281 w2284 w2296 w2298 w2305 w2309 w2313 w2317 w2321 w2325 w2329 w2333 w2337 w2339 w2343 w2347 w2353] -> w2270
          frame "", Default {
          }
          frame "Exit" {
            n1281 = Enqueue Element(queue=w2278, element=CTL_Control_States."Save all settings", error in (no error)=w2280) -> (queue out=w2277:refnum<queue>, error out=w2279:errorcluster)  [unwired: 1 in, 1 out]
            n1282 = Enqueue Element(queue=w2277, element=CTL_Control_States."Close App", error in (no error)=w2279) -> (error out=w2281:errorcluster)  [unwired: 1 in, 2 out]
          }
          frame "Configure port(s)" {
            n1283 = Enqueue Element(queue=w2287, element=CTL_Control_States."Configure port(s)", error in (no error)=w2285) -> (error out=w2284:errorcluster)  [unwired: 1 in, 2 out]
          }
          frame "Timings calibration" {
            n1284 = Enqueue Element(queue=w2293, element=CTL_Control_States."Play Stop", error in (no error)=w2294) -> (queue out=w2291:refnum<queue>, error out=w2292:errorcluster)  [unwired: 1 in, 1 out]
            n1285 = Enqueue Element(queue=w2291, element=CTL_Control_States."Play Start", error in (no error)=w2292) -> (queue out=w2289:refnum<queue>, error out=w2290:errorcluster)  [unwired: 1 in, 1 out]
            n1286 = Enqueue Element(queue=w2289, element=CTL_Control_States."Timings calibration start", error in (no error)=w2290) -> (error out=w2296:errorcluster)  [unwired: 1 in, 2 out]
          }
          frame "Dispension rate calibration" {
            n1287 = Enqueue Element(queue=w2302, element=CTL_Control_States."Play Stop", error in (no error)=w2303) -> (queue out=w2300:refnum<queue>, error out=w2301:errorcluster)  [unwired: 1 in, 1 out]
            n1288 = Enqueue Element(queue=w2300, element=CTL_Control_States."Dispension calibration", error in (no error)=w2301) -> (error out=w2298:errorcluster)  [unwired: 1 in, 2 out]
          }
          frame "I/O Configuration" {
            n1289 = Enqueue Element(queue=w2308, element=CTL_Control_States."Set I/O config", error in (no error)=w2306) -> (error out=w2305:errorcluster)  [unwired: 1 in, 2 out]
          }
          frame "Cage and Recording" {
            n1290 = Enqueue Element(queue=w2312, element=CTL_Control_States."Cage and recording settings", error in (no error)=w2310) -> (error out=w2309:errorcluster)  [unwired: 1 in, 2 out]
          }
          frame "Play Start" {
            n1291 = Enqueue Element(queue=w2316, element=CTL_Control_States."Play Start", error in (no error)=w2314) -> (error out=w2313:errorcluster)  [unwired: 1 in, 2 out]
          }
          frame "Play Stop" {
            n1292 = Enqueue Element(queue=w2320, element=CTL_Control_States."Play Stop", error in (no error)=w2318) -> (error out=w2317:errorcluster)  [unwired: 1 in, 2 out]
          }
          frame "Start Recording" {
            n1293 = Enqueue Element(queue=w2324, element=CTL_Control_States."Start Recording", error in (no error)=w2322) -> (error out=w2321:errorcluster)  [unwired: 1 in, 2 out]
          }
          frame "Stop Recording" {
            n1294 = Enqueue Element(queue=w2328, element=CTL_Control_States."Stop Recording", error in (no error)=w2326) -> (error out=w2325:errorcluster)  [unwired: 1 in, 2 out]
          }
          frame "Start Over" {
            n1295 = Enqueue Element(queue=w2332, element=CTL_Control_States."Start over", error in (no error)=w2330) -> (error out=w2329:errorcluster)  [unwired: 1 in, 2 out]
          }
          frame "Fix broken track" {
            n1296 = Enqueue Element(queue=w2336, element=CTL_Control_States."Recalculate track with new settings", error in (no error)=w2334) -> (error out=w2333:errorcluster)  [unwired: 1 in, 2 out]
          }
          frame "Stream Data" {
            n1297 = call "Show Panel.vi"("error in (no error)"=w2338) -> ("error out"=w2337:errorcluster)  [unwired: 10 in]
          }
          frame "Save density maps" {
            n1298 = Enqueue Element(queue=w2342, element=CTL_Control_States."Save density map(s)", error in (no error)=w2340) -> (error out=w2339:errorcluster)  [unwired: 1 in, 2 out]
          }
          frame "Save Settings" {
            n1299 = Enqueue Element(queue=w2346, element=CTL_Control_States."Save all settings to custom location", error in (no error)=w2344) -> (error out=w2343:errorcluster)  [unwired: 1 in, 2 out]
          }
          frame "Load Settings" {
            n1300 = Enqueue Element(queue=w2350, element=CTL_Control_States."Load custom settings", error in (no error)=w2348) -> (error out=w2347:errorcluster)  [unwired: 1 in, 2 out]
          }
          frame "Open Manual" {
            n1301 = call <vilib>:"Application Directory.vi"() -> ("Application Directory"=w2351:path)
            n1302 = call "Get Abs Manual File Path.vi"("error in (no error)"=w2356, "Application directory"=w2351) -> ("error out"=w2355:errorcluster, "Manual file path"=w2352:path)
            n1303 = call-poly <userlib>:"File Exists__ogtk.vi"("file path"=w2352) -> ("exists"=w2354:bool)  [unwired: 6 in, 1 out]
            n1304 = case shown="False" w2354 {
              tunnel: w2355 -> [w2362 w2365]
              tunnel: [w2361 w2364] -> w2353
              tunnel: w2352 -> [w2360 w2363]
              frame False {
                n1305 = Path To String(path=w2360) -> (string=w2359:string)
                n1306 = Concatenate Strings("Help file not found: " ("string"), w2359) -> (w2358:string)
                n1307 = call "Display Message to User"("error in (no error)"=w2362, "Message"=w2358) -> ("error out"=w2361:errorcluster)  [unwired: 8 in, 1 out]
              }
              frame True {
                n1308 = call <vilib>:"Open a Document on Disk.vi"("error in (no error)"=w2365, "document path"=w2363) -> ("error out"=w2364:errorcluster)  [unwired: 5 in]
              }
            }
          }
        }
      }
      event "Check HW connection": Value Change {
        n1309 = event-data() -> ("CtlRef"=w2368:refnum<vi>, "OldVal"=w2369:bool)  [unwired: 1 in, 4 out]
        n1310 = Enqueue Element(queue=w2373, element=CTL_Control_States."HW Init", error in (no error)=w2366) -> (error out=w2371:errorcluster)  [unwired: 1 in, 2 out]
        n1311 = flat-sequence {
          tunnel: w2371 -> [w2374]
          tunnel: [w2374] -> w2370
          frame #0 {
            n1312 = Wait (ms)(milliseconds to wait=u32 500) -> ()  [unwired: 1 out]
          }
        }
        n1313 = property class="Bool (strict)"(reference=w2368, error in=w2370, "Value"=w2369) -> (error out=w2367:errorcluster)  [unwired: 1 out]
      }
      event "Set IO config": Value Change {
        n1314 = event-data() -> ("CtlRef"=w2378:refnum<vi>, "OldVal"=w2379:bool)  [unwired: 1 in, 4 out]
        n1315 = Enqueue Element(queue=w2383, element=CTL_Control_States."Set I/O config", error in (no error)=w2377) -> (error out=w2381:errorcluster)  [unwired: 1 in, 2 out]
        n1316 = flat-sequence {
          tunnel: w2381 -> [w2384]
          tunnel: [w2384] -> w2380
          frame #0 {
            n1317 = Wait (ms)(milliseconds to wait=u32 300) -> ()  [unwired: 1 out]
          }
        }
        n1318 = property class="Bool (strict)"(reference=w2378, error in=w2380, "Value"=w2379) -> (error out=w2376:errorcluster)  [unwired: 1 out]
      }
      event "Show zones", "Show magnets": Value Change {
        n1319 = event-data() -> ()  [unwired: 1 in, 6 out]
        n1320 = Enqueue Element(queue=w2389, element=CTL_Control_States."Zones layout update", error in (no error)=w2387) -> (error out=w2386:errorcluster)  [unwired: 1 in, 2 out]
      }
      event "Rainbow (time)": Value Change {
        w2391 = FALSE ("Rainbow (speed)")
        n1321 = event-data() -> ("NewVal"=w2392:bool)  [unwired: 1 in, 5 out]
        n1322 = Enqueue Element(queue=w2403, element=CTL_Control_States."Upd. trace length", error in (no error)=w2401) -> (error out=w2397:errorcluster)  [unwired: 1 in, 2 out]
        n1323 = Select(t=i64 53 ("Period"), s=w2392, f=i64 31 ("Period")) -> (s? t:f=w2400:i64)
        n1324 = local read "Show heatmap"() -> (w2390:bool)
        n1325 = local read "Show full track"() -> (w2395:bool)
        n1326 = property on="Rainbow (speed)" class="Bool (strict)"(error in=w2397, "Value"=w2391) -> (error out=w2396:errorcluster)  [unwired: 1 in, 1 out]
        n1327 = local write "UI update period"(w2400) -> ()
        n1328 = Build Array(w2392, w2391, w2395, w2390) -> (w2394:bool[])
        n1329 = Boolean Array To Number(Boolean array=w2394) -> (number=w2393:u32)
        n1330 = local write "Track show state"(w2393) -> ()
      }
      event "Rainbow (speed)": Value Change {
        w2405 = FALSE ("Rainbow (speed)")
        n1331 = event-data() -> ("NewVal"=w2406:bool)  [unwired: 1 in, 5 out]
        n1332 = Enqueue Element(queue=w2417, element=CTL_Control_States."Upd. trace length", error in (no error)=w2415) -> (error out=w2411:errorcluster)  [unwired: 1 in, 2 out]
        n1333 = Select(t=i64 53 ("Period"), s=w2406, f=i64 31 ("Period")) -> (s? t:f=w2414:i64)
        n1334 = local read "Show heatmap"() -> (w2404:bool)
        n1335 = local read "Show full track"() -> (w2409:bool)
        n1336 = property on="Rainbow (time)" class="Bool (strict)"(error in=w2411, "Value"=w2405) -> (error out=w2410:errorcluster)  [unwired: 1 in, 1 out]
        n1337 = local write "UI update period"(w2414) -> ()
        n1338 = Build Array(w2405, w2406, w2409, w2404) -> (w2408:bool[])
        n1339 = Boolean Array To Number(Boolean array=w2408) -> (number=w2407:u32)
        n1340 = local write "Track show state"(w2407) -> ()
      }
      event "Show heatmap": Value Change {
        n1341 = event-data() -> ("NewVal"=w2430:bool)  [unwired: 1 in, 5 out]
        n1342 = local read "Timeline"() -> (w2427:T37)
        n1343 = Unbundle By Name(w2427) -> ("Slider"=w2426:dbl, "Slider"=w2425:dbl)
        n1344 = First Call?() -> (First Call?: T/F=w2418:bool)
        n1345 = call <vilib>:"Value Has Changed PtByPt.vi"("input data point"=w2426, "initialize"=w2418) -> ("has changed"=w2423:bool)  [unwired: 1 out]
        n1346 = call <vilib>:"Value Has Changed PtByPt.vi"("input data point"=w2425, "initialize"=w2418) -> ("has changed"=w2422:bool)  [unwired: 1 out]
        n1347 = Compound Arithmetic op=OR(w2423, w2422) -> (w2424:bool)
        n1348 = case shown="True" w2430 {
          selector: w2430 -> [_ w2454]
          tunnel: w2428 -> [w2450 w2456]
          tunnel: [w2442 w2456] -> w2420
          tunnel: [w2448 w2453] -> w2429
          frame True {
            w2449 = FALSE ("Show full track")
            n1349 = local read "Rainbow (time)"() -> (w2446:bool)
            n1350 = local read "Rainbow (speed)"() -> (w2447:bool)
            n1351 = local read "Show heatmap"() -> (w2451:bool)
            n1352 = property on="Show full track" class="Bool (strict)"(error in=w2450, "Value"=w2449) -> (error out=w2443:errorcluster)  [unwired: 1 in, 1 out]
            n1353 = Select(t=w2446, s=w2447, f=TRUE) -> (s? t:f=w2444:bool)
            n1354 = property on="Rainbow (time)" class="Bool (strict)"(error in=w2443, "Value"=w2444) -> (error out=w2442:errorcluster)  [unwired: 1 in, 1 out]
            n1355 = Build Array(w2444, w2447, w2449, w2451) -> (w2452:bool[])
            n1356 = Boolean Array To Number(Boolean array=w2452) -> (number=w2448:u32)
          }
          frame False {
            n1357 = local read "Rainbow (time)"() -> (w2458:bool)
            n1358 = local read "Rainbow (speed)"() -> (w2457:bool)
            n1359 = local read "Show full track"() -> (w2455:bool)
            n1360 = Build Array(w2458, w2457, w2455, w2454) -> (w2459:bool[])
            n1361 = Boolean Array To Number(Boolean array=w2459) -> (number=w2453:u32)
          }
        }
        n1362 = case shown="True" w2424 {
          tunnel: w2421 -> [_ w2435]
          tunnel: w2420 -> [w2431 w2432]
          tunnel: [w2431 w2439] -> w2419
          frame False {
          }
          frame True {
            n1363 = Enqueue Element(queue=w2435, element=CTL_Control_States."Overlay tracks update", error in (no error)=w2432) -> (queue out=w2433:refnum<queue>, error out=w2436:errorcluster)  [unwired: 1 in, 1 out]
            n1364 = Enqueue Element(queue=w2433, element=CTL_Control_States."Location map update", error in (no error)=w2436) -> (queue out=w2438:refnum<queue>, error out=w2440:errorcluster)  [unwired: 1 in, 1 out]
            n1365 = Enqueue Element(queue=w2438, element=CTL_Control_States."Speed map update", error in (no error)=w2440) -> (error out=w2439:errorcluster)  [unwired: 1 in, 2 out]
          }
        }
        n1366 = local write "Track show state"(w2429) -> ()
      }
      event "Show full track": Value Change {
        n1367 = event-data() -> ("NewVal"=w2463:bool)  [unwired: 1 in, 5 out]
        n1368 = case shown="False" w2463 {
          tunnel: w2461 -> [w2466 w2473]
          tunnel: [w2468 w2475] -> w2462
          tunnel: [w2464 w2473] -> w2460
          frame True {
            w2465 = FALSE ("Show full track")
            n1369 = local read "Rainbow (time)"() -> (w2470:bool)
            n1370 = local read "Rainbow (speed)"() -> (w2469:bool)
            n1371 = local read "Show full track"() -> (w2467:bool)
            n1372 = property on="Show heatmap" class="Bool (strict)"(error in=w2466, "Value"=w2465) -> (error out=w2464:errorcluster)  [unwired: 1 in, 1 out]
            n1373 = Build Array(w2470, w2469, w2467, w2465) -> (w2471:bool[])
            n1374 = Boolean Array To Number(Boolean array=w2471) -> (number=w2468:u32)
          }
          frame False {
            n1375 = local read "Rainbow (time)"() -> (w2477:bool)
            n1376 = local read "Rainbow (speed)"() -> (w2476:bool)
            n1377 = local read "Show full track"() -> (w2474:bool)
            n1378 = local read "Show heatmap"() -> (w2472:bool)
            n1379 = Build Array(w2477, w2476, w2474, w2472) -> (w2478:bool[])
            n1380 = Boolean Array To Number(Boolean array=w2478) -> (number=w2475:u32)
          }
        }
        n1381 = local write "Track show state"(w2462) -> ()
      }
      event "Timeline": Mouse Up {
        n1382 = event-data() -> ()  [unwired: 1 in, 8 out]
        n1383 = local read "Timeline"() -> (w2491:T37)
        n1384 = Unbundle By Name(w2491) -> ("Slider"=w2490:dbl, "Slider"=w2489:dbl, "Slider"=w2486:dbl)
        n1385 = First Call?() -> (First Call?: T/F=w2484:bool)
        n1386 = local read "Play/Pause"() -> (w2492:bool)
        n1387 = Not(x=w2492) -> (.not. x?=w2485:bool)
        n1388 = call <vilib>:"Value Has Changed PtByPt.vi"("input data point"=w2486, "initialize"=w2484) -> ("has changed"=w2483:bool)  [unwired: 1 out]
        n1389 = call <vilib>:"Value Has Changed PtByPt.vi"("input data point"=w2490, "initialize"=w2484) -> ("has changed"=w2482:bool)  [unwired: 1 out]
        n1390 = call <vilib>:"Value Has Changed PtByPt.vi"("input data point"=w2489, "initialize"=w2484) -> ("has changed"=w2481:bool)  [unwired: 1 out]
        n1391 = Compound Arithmetic op=OR(w2482, w2481, w2483) -> (w2487:bool)
        n1392 = And(x=w2485, y=w2487) -> (x .and. y?=w2488:bool)
        n1393 = Or(x=w2482, y=w2481) -> (x .or. y?=w2480:bool)
        n1394 = case shown="True" w2488 {
          tunnel: w2494 -> [w2495 w2502]
          tunnel: w2493 -> [w2496 w2503]
          tunnel: [w2496 w2500] -> w2479
          tunnel: [w2495 w2499] -> _
          tunnel: w2480 -> [_ w2501]
          frame False {
          }
          frame True {
            n1395 = Enqueue Element(queue=w2502, element=CTL_Control_States."Timeline update", error in (no error)=w2503) -> (queue out=w2498:refnum<queue>, error out=w2497:errorcluster)  [unwired: 1 in, 1 out]
            n1396 = case shown="True" w2501 {
              tunnel: [w2506 w2513] -> w2500
              tunnel: [w2505 w2512] -> w2499
              tunnel: w2498 -> [w2505 w2510]
              tunnel: w2497 -> [w2506 w2509]
              frame False {
              }
              frame True {
                n1397 = Enqueue Element(queue=w2510, element=CTL_Control_States."Overlay tracks update", error in (no error)=w2509) -> (queue out=w2508:refnum<queue>, error out=w2507:errorcluster)  [unwired: 1 in, 1 out]
                n1398 = Enqueue Element(queue=w2508, element=CTL_Control_States."Location map update", error in (no error)=w2507) -> (queue out=w2516:refnum<queue>, error out=w2515:errorcluster)  [unwired: 1 in, 1 out]
                n1399 = Enqueue Element(queue=w2516, element=CTL_Control_States."Speed map update", error in (no error)=w2515) -> (queue out=w2512:refnum<queue>, error out=w2513:errorcluster)  [unwired: 1 in, 1 out]
              }
            }
          }
        }
      }
      event "Add Reward": Value Change {
        n1400 = event-data() -> ("OldVal"=w2522:bool)  [unwired: 1 in, 5 out]
        n1401 = local write "Add Reward"(w2522) -> ()
        n1402 = Enqueue Element(queue=w2519, element=CTL_Control_States."Add Reward condition", error in (no error)=w2521) -> (error out=w2520:errorcluster)  [unwired: 1 in, 2 out]
      }
      event "Modify Reward": Value Change {
        n1403 = event-data() -> ("OldVal"=w2527:bool)  [unwired: 1 in, 5 out]
        n1404 = local write "Modify Reward"(w2527) -> ()
        n1405 = Enqueue Element(queue=w2524, element=CTL_Control_States."Modify Reward condition", error in (no error)=w2526) -> (error out=w2525:errorcluster)  [unwired: 1 in, 2 out]
      }
      event "Remove Reward": Value Change {
        n1406 = event-data() -> ("OldVal"=w2532:bool)  [unwired: 1 in, 5 out]
        n1407 = local write "Remove Reward"(w2532) -> ()
        n1408 = Enqueue Element(queue=w2529, element=CTL_Control_States."Delete Reward condition", error in (no error)=w2531) -> (error out=w2530:errorcluster)  [unwired: 1 in, 2 out]
      }
      event "Reward and stimulation": Value Change; "Reward and stimulation": Double Click; "Reward and stimulation": Mouse Down {
        n1409 = event-data() -> ()  [unwired: 1 in, 4 out]
        n1410 = Enqueue Element(queue=w2534, element=CTL_Control_States."Check Reward condition(s)", error in (no error)=w2536) -> (error out=w2535:errorcluster)  [unwired: 1 in, 2 out]
      }
      event "Diagram (display)": Mouse Up {
        n1411 = event-data() -> ()  [unwired: 1 in, 8 out]
        n1412 = property on="Diagram (display)" class="ImageControl"(error in=w2545) -> (error out=w2538:errorcluster, "ROI"=w2544:T29)  [unwired: 1 in, 1 out]
        n1413 = local write "ROIs"(w2544) -> ()
        n1414 = Unbundle By Name(w2544) -> ("Contours"=w2543:T93)
        n1415 = for {
          tunnel: w2543 -> [w2553] mode=indexing
          tunnel: [w2550] -> w2541 mode=indexing
          tunnel: [w2546] -> w2542 mode=indexing
          i -> [w2552]
          n1416 = Unbundle By Name(w2553) -> ("ROI Type"=w2547:u32)
          n1417 = Increment(x=w2552) -> (x+1=w2551:i32)
          n1418 = case shown="0, Default" w2547 {
            tunnel: ["Unknown" "Rect" "Rot. rect" "Polygon" "Freehand" "Oval" "Annulus"] -> w2546
            frame 0, Default {
            }
            frame 3 {
            }
            frame 12 {
            }
            frame 5 {
            }
            frame 6 {
            }
            frame 4 {
            }
            frame 7 {
            }
          }
          n1419 = Format Value(string ("")="ROI #" ("string"), format string="%02u", value (0)=w2551) -> (output string=w2550:string)
        }
        n1420 = Build Array(w2542) -> (w2540:string[][])
        n1421 = Transpose 2D Array(2D array=w2540) -> (transposed array=w2539:string[][])
        n1422 = property on="ROIs list" class="MCListbox (strict)"(error in=w2538, "ItemNames"=w2539, "RowHdrs[]"=w2541) -> (error out=w2537:errorcluster)  [unwired: 1 in, 1 out]
      }
      event "Multiplyer of chart RX": Value Change {
        n1423 = event-data() -> ("NewVal"=w2561:u8)  [unwired: 1 in, 5 out]
        n1424 = property on="Mouse speed" class="WFChart (strict)"(error in=w2568) -> (error out=w2562:errorcluster, "XScale.Minimum"=w2565:dbl)  [unwired: 1 in, 1 out]
        n1425 = Scale By Power Of 2(n=w2561, x=10) -> (x*2^n=w2564:i32)
        n1426 = Add(x=w2565, y=w2564) -> (x+y=w2563:dbl)
        n1427 = property on="Mouse speed" class="WFChart (strict)"(error in=w2562, "XScale.Maximum"=w2563) -> (error out=w2567:errorcluster)  [unwired: 1 in, 1 out]
      }
      event Value Change {
        n1428 = event-data() -> ("NewVal"=w2570:T14)  [unwired: 1 in, 5 out]
        n1429 = local read "Settings cluster (local)"() -> (w2572:T16)
        n1430 = call "SW_Update_radial_segmentation_variable_info.vi"("error in (no error)"=w2573, "NewVal"=w2570, "Settings cluster (local) in"=w2572) -> ("error out"=w2569:errorcluster, "Settings cluster (local) out"=w2571:T16)  [unwired: 1 in]
        n1431 = Enqueue Element(queue=w2577, element=CTL_Control_States."Zones layout update", error in (no error)=w2569) -> (error out=w2575:errorcluster)  [unwired: 1 in, 2 out]
        n1432 = local write "Settings cluster (local)"(w2571) -> ()
        n1433 = call "100 ms"("error in (no error)"=w2575) -> ("error out"=w2574:errorcluster)  [unwired: 10 in]
      }
      event User Event {
        n1434 = event-data() -> ("Active rules"=w2580:bool[])  [unwired: 1 in, 4 out]
        n1435 = Array To Cluster(array=w2580) -> (cluster=w2579:T94)
        n1436 = local write "Active rules"(w2579) -> ()
      }
      event "Play/Pause": Value Change {
        n1437 = event-data() -> ("NewVal"=w2587:bool)  [unwired: 1 in, 5 out]
        n1438 = Get Notifier Status(notifier=w2585, error in (no error)=w2584) -> (current notification=w2582:T46, error out=w2583:errorcluster)  [unwired: 3 out]
        n1439 = Unbundle By Name(w2582) -> ("Offline mode"=w2581:bool)
        n1440 = case shown="False" w2581 {
          tunnel: w2588 -> [w2592 w2604]
          tunnel: w2587 -> [w2591 w2603]
          tunnel: w2583 -> [w2590 w2602]
          tunnel: [w2589 w2601] -> w2586
          frame True {
            # "Offline mode"
            n1441 = case shown="True" w2591 {
              tunnel: w2592 -> [w2595 w2600]
              tunnel: w2590 -> [w2594 w2598]
              tunnel: [w2593 w2597] -> w2589
              frame True {
                # "Play Start"
                n1442 = Enqueue Element(queue=w2595, element=CTL_Control_States."Play Start", error in (no error)=w2594) -> (error out=w2593:errorcluster)  [unwired: 1 in, 2 out]
              }
              frame False {
                # "Play Stop"
                n1443 = Enqueue Element(queue=w2600, element=CTL_Control_States."Play Stop", error in (no error)=w2598) -> (error out=w2597:errorcluster)  [unwired: 1 in, 2 out]
              }
            }
          }
          frame False {
            # "Online mode"
            n1444 = case shown="True" w2603 {
              tunnel: w2604 -> [w2605 w2615]
              tunnel: w2602 -> [w2610 w2613]
              tunnel: [w2607 w2612] -> w2601
              frame True {
                # "Play Start"
                n1445 = call <vilib>:"Set Busy.vi"("error in (no error)"=w2610) -> ("error out"=w2609:errorcluster)  [unwired: 9 in, 1 out]
                n1446 = Enqueue Element(queue=w2605, element=CTL_Control_States."Play Start", error in (no error)=w2609) -> (error out=w2608:errorcluster)  [unwired: 1 in, 2 out]
                n1447 = call "1.5s delay"("error in (no error)"=w2608) -> ("error out"=w2606:errorcluster)  [unwired: 10 in]
                n1448 = call <vilib>:"Unset Busy.vi"("error in (no error)"=w2606) -> ("error out"=w2607:errorcluster)  [unwired: 10 in]
              }
              frame False {
                # "Play Stop"
                n1449 = Enqueue Element(queue=w2615, element=CTL_Control_States."Play Stop", error in (no error)=w2613) -> (error out=w2612:errorcluster)  [unwired: 1 in, 2 out]
              }
            }
          }
        }
      }
      event "Start over": Value Change {
        n1450 = event-data() -> ("NewVal"=w2622:bool)  [unwired: 1 in, 5 out]
        n1451 = Get Notifier Status(notifier=w2620, error in (no error)=w2619) -> (current notification=w2617:T46, error out=w2618:errorcluster)  [unwired: 3 out]
        n1452 = Unbundle By Name(w2617) -> ("Offline mode"=w2616:bool)
        n1453 = case shown="True" w2616 {
          tunnel: w2623 -> [w2627 _]
          tunnel: w2622 -> [w2626 _]
          tunnel: w2618 -> [w2625 w2636]
          tunnel: [w2624 w2636] -> w2621
          frame True {
            # "Offline mode"
            n1454 = case shown="True" w2626 {
              tunnel: w2627 -> [w2630 w2635]
              tunnel: w2625 -> [w2629 w2633]
              tunnel: [w2628 w2632] -> w2624
              frame True {
                # "Play Start"
                n1455 = Enqueue Element(queue=w2630, element=CTL_Control_States."Start over", error in (no error)=w2629) -> (error out=w2628:errorcluster)  [unwired: 1 in, 2 out]
              }
              frame False {
                # "Play Stop"
                n1456 = Enqueue Element(queue=w2635, element=CTL_Control_States."Play Stop", error in (no error)=w2633) -> (error out=w2632:errorcluster)  [unwired: 1 in, 2 out]
              }
            }
          }
          frame False {
            # "Online mode"
          }
        }
      }
      event "Record/Stop": Value Change {
        n1457 = event-data() -> ("NewVal"=w2639:bool)  [unwired: 1 in, 5 out]
        n1458 = case shown="False" w2639 {
          tunnel: w2640 -> [w2643 w2648]
          tunnel: w2638 -> [w2642 w2646]
          tunnel: [w2641 w2645] -> w2637
          frame True {
            # "Record Start"
            n1459 = Enqueue Element(queue=w2643, element=CTL_Control_States."Start Recording", error in (no error)=w2642) -> (error out=w2641:errorcluster)  [unwired: 1 in, 2 out]
          }
          frame False {
            # "Recording Stop"
            n1460 = Enqueue Element(queue=w2648, element=CTL_Control_States."Stop Recording", error in (no error)=w2646) -> (error out=w2645:errorcluster)  [unwired: 1 in, 2 out]
          }
        }
      }
      event "Trace, s": Value Change {
        n1461 = event-data() -> ()  [unwired: 1 in, 6 out]
        n1462 = Enqueue Element(queue=w2652, element=CTL_Control_States."Upd. trace length", error in (no error)=w2650) -> (error out=w2649:errorcluster)  [unwired: 1 in, 2 out]
      }
      event "Open File": Value Change {
        n1463 = event-data() -> ("OldVal"=w2657:bool)  [unwired: 1 in, 5 out]
        n1464 = local write "Open File"(w2657) -> ()
        n1465 = Enqueue Element(queue=w2654, element=CTL_Control_States."Load recorded data", error in (no error)=w2653) -> (error out=w2656:errorcluster)  [unwired: 1 in, 2 out]
      }
      event "Reset barplot": Value Change {
        n1466 = event-data() -> ("OldVal"=w2658:bool)  [unwired: 1 in, 5 out]
        n1467 = flat-sequence {
          tunnel: [w2662] -> w2659
          tunnel: w2658 -> [w2662]
          frame #0 {
            n1468 = Wait (ms)(milliseconds to wait=u32 10) -> ()  [unwired: 1 out]
          }
        }
        n1469 = local write "Reset barplot"(w2659) -> ()
      }
      event Value Change {
        n1470 = event-data() -> ("NewVal"=w2667:T38)  [unwired: 1 in, 5 out]
        n1471 = To Unsigned Byte Integer(number=w2667) -> (unsigned 8bit integer=w2668:u8)
        n1472 = Build Array(w2668) -> (w2666:u8[])
        n1473 = flat-sequence {
          tunnel: w2666 -> [w2669]
          tunnel: w2665 -> [w2673]
          tunnel: w2664 -> [w2672]
          tunnel: [w2671] -> w2663
          frame #0 {
            n1474 = global write "SW_Globals_2.2+.vi" "Regions to mark selected"(w2669) -> ()
          }
          frame #1 {
            n1475 = Wait (ms)(milliseconds to wait=u32 50) -> ()  [unwired: 1 out]
          }
          frame #2 {
            n1476 = Enqueue Element(queue=w2673, element=CTL_Control_States."Zones layout update", error in (no error)=w2672) -> (error out=w2671:errorcluster)  [unwired: 1 in, 2 out]
          }
        }
      }
      event "Speed threshold": Value Change {
        n1477 = event-data() -> ()  [unwired: 1 in, 6 out]
        n1478 = Enqueue Element(queue=w2681, element=CTL_Control_States."Zones layout update", error in (no error)=w2680) -> (queue out=w2676:refnum<queue>, error out=w2678:errorcluster)  [unwired: 1 in, 1 out]
        n1479 = Enqueue Element(queue=w2676, element=CTL_Control_States."Overlay tracks update", error in (no error)=w2678) -> (error out=w2677:errorcluster)  [unwired: 1 in, 2 out]
      }
      event Key Down {
        n1480 = event-data() -> ("VKey"=w2684:T95, "ScanCode"=w2685:i16)  [unwired: 1 in, 8 out]
        n1481 = case shown="72, 75, 77, 80" w2685 {
          tunnel: w2684 -> [_ w2690]
          tunnel: w2683 -> [w2686 w2689]
          tunnel: [w2686 w2688] -> w2682
          frame Default {
          }
          frame 72, 75, 77, 80 {
            n1482 = Format Into String(format string="%s", error in=w2689, w2690) -> (resulting string=w2687:string, error out=w2688:errorcluster)  [unwired: 1 in]
            n1483 = local write "Key_pressed"(w2687) -> ()
          }
        }
      }
      event Key Up {
        n1484 = event-data() -> ("ScanCode"=w2692:i16, "Mods"=w2695:cluster{"Num Pad":bool, "Menu Key":bool})  [unwired: 1 in, 5 out]
        n1485 = case shown="72, 75, 77, 80" w2692 {
          tunnel: w2695 -> [_ _]
          tunnel: w2694 -> [w2696 w2698]
          tunnel: [w2696 w2698] -> w2693
          frame Default {
          }
          frame 72, 75, 77, 80 {
            n1486 = local write "Key_pressed"("----" ("Key_pressed")) -> ()
          }
        }
      }
    }
    n1487 = call <vilib>:"Simple Error Handler.vi"("error in (no error)"=w2253) -> ("error out"=w2255:errorcluster)  [unwired: 4 in, 4 out]
    n1488 = node-c288(w2255) -> ()  [unwired: 1 out]
  }
  n1489 = node-c288(w42) -> (w3:errorcluster)
  n1490 = node-c288(w34) -> (w30:errorcluster)
  n1491 = node-c288(w64) -> (w46:errorcluster)
  n1492 = node-c288(w53) -> (w29:errorcluster)
  n1493 = node-c288(w59) -> (w47:errorcluster)
  n1494 = node-c288(w71) -> (w48:errorcluster)
  n1495 = Flush Queue(queue=w67, error in (no error)=w48) -> (queue out=w66:refnum<queue>, error out=w49:errorcluster)  [unwired: 1 out]
  n1496 = Merge Errors(w29, w30, w3) -> (w38:errorcluster)
  n1497 = Release Queue(queue=w66, error in (no error)=w49) -> (error out=w45:errorcluster)  [unwired: 1 in, 2 out]
  n1498 = Merge Errors(w45, w46, w47, w38) -> (w11:errorcluster)
  n1499 = Unregister For Events(event registration refnum=w12, error in=w11) -> (error out=w10:errorcluster)
  n1500 = Release Notifier(notifier=w44, error in (no error)=w10) -> (error out=w21:errorcluster)  [unwired: 1 in, 2 out]
  n1501 = call <vilib>:"Clear Timing Source.vi"("error in (no error)"=w21, "name"=w19) -> ("error out"=→"error out":errorcluster)  [unwired: 8 in, 1 out]
